vi "string parse mathematica list assosiated array -- V2.vi"(6 "pattern":string="^[\\t \\r \\n \\s \\, ]*\\\"(.+?)\\\"[\\t \\r \\n \\s]*\\-\\>[\\t \\r \\n \\s]*\\<\\|([^\\|]+)\\|\\>", 7 "action":T2=enum."create string", 8 "array of inds":dbl[](array[numeric]), 9 "array of IDs":string[](array[string]), 10 "Map IN":map{string, map{T1, dbl}}(c390), 11 "string IN":string="\n8048 -> <|\"\\[Zeta]\" -> 0.264284777894, \"\\[Tau]1\" -> 0.029921918685, \n   \"\\[Tau]S\" -> 0.192386764745, \"\\[Tau]N\" -> 0.181403587913, \n   \"\\[Tau]C\" -> 0.001052808010, \"\\[Kappa]0\" -> 0.000000000660, \n   \"mm1\" -> 0.000000000000, \"mm2\" -> 0.000000000000, \n   \"mm3\" -> 0.000000000000, \"T\" -> 0.170000000000, \n   \"B\" -> 12, \"\\[Theta]\" -> 0.000000000000|>, \n8049 -> <|\"\\[Zeta]\" -> 0.201102232421, \"\\[Tau]1\" -> 0.027404257658, \n   \"\\[Tau]S\" -> 0.119081991530, \"\\[Tau]N\" -> 0.102233037825, \n   \"\\[Tau]C\" -> 0.001034759526, \"\\[Kappa]0\" -> 0.000000000924, \n   \"mm1\" -> 0.000000000000, \"mm2\" -> 0.000000000000, \n   \"mm3\" -> 0.000000000000, \"T\" -> 0.200000000000, \n   \"B\" -> 12, \"\\[Theta]\" -> 0.000000000000|>, \n8050 -> <|\"\\[Zeta]\" -> 0.169063131197, \"\\[Tau]1\" -> 0.023551252455, \n   \"\\[Tau]S\" -> 0.088556796938, \"\\[Tau]N\" -> 0.073591360902, \n   \"\\[Tau]C\" -> 0.001008773464, \"\\[Kappa]0\" -> 0.000000001052, \n   \"mm1\" -> 0.000000000000, \"mm2\" -> 0.000000000000, \n   \"mm3\" -> 0.000000000000, \"T\" -> 0.220000000000, \n   \"B\" -> 12, \"\\[Theta]\" -> 0.000000000000|>, \n8051 -> <|\"\\[Zeta]\" -> 0.091539753140, \"\\[Tau]1\" -> 0.021589342173, \n   \"\\[Tau]S\" -> 0.069591266812, \"\\[Tau]N\" -> 0.024713101747, \n   \"\\[Tau]C\" -> 0.001578835918, \"\\[Kappa]0\" -> 0.000000001376, \n   \"mm1\" -> 0.000000000000, \"mm2\" -> 0.000000000000, \n   \"mm3\" -> 0.000000000000, \"T\" -> 0.280000000000, \n   \"B\" -> 12, \"\\[Theta]\" -> 0.000000000000|>, \n8052 -> <|\"\\[Zeta]\" -> 0.064241434685, \"\\[Tau]1\" -> 0.021883189624, \n   \"\\[Tau]S\" -> 0.054526069267, \"\\[Tau]N\" -> 0.012051949674, \n   \"\\[Tau]C\" -> 0.001858120134, \"\\[Kappa]0\" -> 0.000000001749, \n   \"mm1\" -> 0.000000000000, \"mm2\" -> 0.000000000000, \n   \"mm3\" -> 0.000000000000, \"T\" -> 0.330000000000, \n   \"B\" -> 12, \"\\[Theta]\" -> 0.000000000000|>, \n8053 -> <|\"\\[Zeta]\" -> 0.046671238462, \"\\[Tau]1\" -> 0.021035137247, \n   \"\\[Tau]S\" -> 0.044251032051, \"\\[Tau]N\" -> 0.006393660877, \n   \"\\[Tau]C\" -> 0.002341606240, \"\\[Kappa]0\" -> 0.000000002165, \n   \"mm1\" -> 0.000000000000, \"mm2\" -> 0.000000000000, \n   \"mm3\" -> 0.000000000000, \"T\" -> 0.400000000000, \n   \"B\" -> 12, \"\\[Theta]\" -> 0.000000000000|>, \n 8054 -> <|\"\\[Zeta]\" -> 0.036507468942, \"\\[Tau]1\" -> 0.016809078537, \n   \"\\[Tau]S\" -> 0.036180977899, \"\\[Tau]N\" -> 0.004191377428, \n   \"\\[Tau]C\" -> 0.002304673955, \"\\[Kappa]0\" -> 0.000000002675, \n   \"mm1\" -> 0.000000000000, \"mm2\" -> 0.000000000000, \n   \"mm3\" -> 0.000000000000, \"T\" -> 0.480000000000, \n   \"B\" -> 12, \"\\[Theta]\" -> 0.000000000000|>, \n 8055 -> <|\"\\[Zeta]\" -> 0.030833243094, \"\\[Tau]1\" -> 0.018820733306, \n   \"\\[Tau]S\" -> 0.030309186701, \"\\[Tau]N\" -> 0.002241639015, \n   \"\\[Tau]C\" -> 0.002272740822, \"\\[Kappa]0\" -> 0.000000003352, \n   \"mm1\" -> 0.000000000000, \"mm2\" -> 0.000000000000, \n   \"mm3\" -> 0.000000000000, \"T\" -> 0.580000000000, \n   \"B\" -> 12, \"\\[Theta]\" -> 0.000000000000|>, \n 8056 -> <|\"\\[Zeta]\" -> 0.019920170845, \"\\[Tau]1\" -> 0.016368892412, \n   \"\\[Tau]S\" -> 0.030579536580, \"\\[Tau]N\" -> 0.001736017565, \n   \"\\[Tau]C\" -> 0.004971418152, \"\\[Kappa]0\" -> 0.000000004410, \n   \"mm1\" -> 0.000000000000, \"mm2\" -> 0.000000000000, \n   \"mm3\" -> 0.000000000000, \"T\" -> 0.680000000000, \n   \"B\" -> 12, \"\\[Theta]\" -> 0.000000000000|>, \n 8057 -> <|\"\\[Zeta]\" -> 0.017558473054, \"\\[Tau]1\" -> 0.014545104284, \n   \"\\[Tau]S\" -> 0.022979681288, \"\\[Tau]N\" -> 0.000840829385, \n   \"\\[Tau]C\" -> 0.005228030240, \"\\[Kappa]0\" -> 0.000000006068, \n   \"mm1\" -> 0.000000000000, \"mm2\" -> 0.000000000000, \n   \"mm3\" -> 0.000000000000, \"T\" -> 0.910000000000, \n   \"B\" -> 12, \"\\[Theta]\" -> 0.000000000000|>, \n 8058 -> <|\"\\[Zeta]\" -> 0.011916480594, \"\\[Tau]1\" -> 0.012551282481, \n   \"\\[Tau]S\" -> 0.018233218660, \"\\[Tau]N\" -> 0.000345702746, \n   \"\\[Tau]C\" -> 0.004699451527, \"\\[Kappa]0\" -> 0.000000008451, \n   \"mm1\" -> 0.000000000000, \"mm2\" -> 0.000000000000, \n   \"mm3\" -> 0.000000000000, \"T\" -> 1.230000000000, \n   \"B\" -> 12, \"\\[Theta]\" -> 0.000000000000|>, \n 8059 -> <|\"\\[Zeta]\" -> 0.012831327568, \"\\[Tau]1\" -> 0.013315909415, \n   \"\\[Tau]S\" -> 0.012590836847, \"\\[Tau]N\" -> 0.000065003013, \n   \"\\[Tau]C\" -> 0.005276356243, \"\\[Kappa]0\" -> 0.000000013610, \n   \"mm1\" -> 0.000000000000, \"mm2\" -> 0.000000000000, \n   \"mm3\" -> 0.000000000000, \"T\" -> 1.970000000000, \n   \"B\" -> 12, \"\\[Theta]\" -> 0.000000000000|>, \n 8060 -> <|\"\\[Zeta]\" -> 0.019774146838, \"\\[Tau]1\" -> 0.013257273421, \n   \"\\[Tau]S\" -> 0.007064131508, \"\\[Tau]N\" -> 0.000028000819, \n   \"\\[Tau]C\" -> 0.006942241845, \"\\[Kappa]0\" -> 0.000000023477, \n   \"mm1\" -> 0.000000000000, \"mm2\" -> 0.000000000000, \n   \"mm3\" -> 0.000000000000, \"T\" -> 3.190000000000, \n   \"B\" -> 12, \"\\[Theta]\" -> 0.000000000000|>, \n 8061 -> <|\"\\[Zeta]\" -> 0.029251354442, \"\\[Tau]1\" -> 0.014634751206, \n   \"\\[Tau]S\" -> 0.003873958746, \"\\[Tau]N\" -> 0.000007000487, \n   \"\\[Tau]C\" -> 0.006827504775, \"\\[Kappa]0\" -> 0.000000056438, \n   \"mm1\" -> 0.000000000000, \"mm2\" -> 0.000000000000, \n   \"mm3\" -> 0.000000000000, \"T\" -> 5.820000000000, \n   \"B\" -> 12, \"\\[Theta]\" -> 0.000000000000 |>, \n   \n 8070 -> <|\"\\[Zeta]\" -> 0.192260325342, \"\\[Tau]1\" -> 0.068971960572, \n   \"\\[Tau]S\" -> 0.034724103146, \"\\[Tau]N\" -> 0.116916926394, \n   \"\\[Tau]C\" -> 0.001339007531, \"\\[Kappa]0\" -> 0.000000000920, \n   \"mm1\" -> 0.000000000000, \"mm2\" -> 0.000000000000, \n   \"mm3\" -> 0.000000000000, \"T\" -> 0.200000000000, \n   \"B\" -> 12, \"\\[Theta]\" -> 90.000000000000 |>, \n   \n 8071 -> <|\"\\[Zeta]\" -> 0.287121975239, \"\\[Tau]1\" -> 0.116231019165, \n   \"\\[Tau]S\" -> 0.066964365948, \"\\[Tau]N\" -> 1.031943818405, \n   \"\\[Tau]C\" -> 0.001579683432, \"\\[Kappa]0\" -> 0.000000000546, \n   \"mm1\" -> 0.000000000000, \"mm2\" -> 0.000000000000, \n   \"mm3\" -> 0.000000000000, \"T\" -> 0.140000000000, \n   \"B\" -> 12, \"\\[Theta]\" -> 90.000000000000 |>, \n   \n 8072 -> <|\"\\[Zeta]\" -> 0.256563977847, \"\\[Tau]1\" -> 0.091128230148, \n   \"\\[Tau]S\" -> 0.042349271948, \"\\[Tau]N\" -> 0.264223732455, \n   \"\\[Tau]C\" -> 0.001175524600, \"\\[Kappa]0\" -> 0.000000000659, \n   \"mm1\" -> 0.000000000000, \"mm2\" -> 0.000000000000, \n   \"mm3\" -> 0.000000000000, \"T\" -> 0.180000000000, \n   \"B\" -> 12, \"\\[Theta]\" -> 90.000000000000|>, \n 8073 -> <|\"\\[Zeta]\" -> 0.166463706425, \"\\[Tau]1\" -> 0.068258677765, \n   \"\\[Tau]S\" -> 0.032169678694, \"\\[Tau]N\" -> 0.089325850968, \n   \"\\[Tau]C\" -> 0.001296501731, \"\\[Kappa]0\" -> 0.000000001072, \n   \"mm1\" -> 0.000000000000, \"mm2\" -> 0.000000000000, \n   \"mm3\" -> 0.000000000000, \"T\" -> 0.220000000000, \n   \"B\" -> 12, \"\\[Theta]\" -> 90.000000000000|>, \n 8074 -> <|\"\\[Zeta]\" -> 0.096966986681, \"\\[Tau]1\" -> 0.051268159149, \n   \"\\[Tau]S\" -> 0.027100433808, \"\\[Tau]N\" -> 0.035158364681, \n   \"\\[Tau]C\" -> 0.001794012368, \"\\[Kappa]0\" -> 0.000000001377, \n   \"mm1\" -> 0.000000000000, \"mm2\" -> 0.000000000000, \n   \"mm3\" -> 0.000000000000, \"T\" -> 0.270000000000, \n   \"B\" -> 12, \"\\[Theta]\" -> 90.000000000000|>, \n 8075 -> <|\"\\[Zeta]\" -> 0.069751073871, \"\\[Tau]1\" -> 0.043839592936, \n   \"\\[Tau]S\" -> 0.023745040482, \"\\[Tau]N\" -> 0.017573258627, \n   \"\\[Tau]C\" -> 0.001911807541, \"\\[Kappa]0\" -> 0.000000001743, \n   \"mm1\" -> 0.000000000000, \"mm2\" -> 0.000000000000, \n   \"mm3\" -> 0.000000000000, \"T\" -> 0.330000000000, \n   \"B\" -> 12, \"\\[Theta]\" -> 90.000000000000|>, \n 8076 -> <|\"\\[Zeta]\" -> 0.051456166730, \"\\[Tau]1\" -> 0.036962114127, \n   \"\\[Tau]S\" -> 0.021589166615, \"\\[Tau]N\" -> 0.010172333923, \n   \"\\[Tau]C\" -> 0.002367575609, \"\\[Kappa]0\" -> 0.000000002122, \n   \"mm1\" -> 0.000000000000, \"mm2\" -> 0.000000000000, \n   \"mm3\" -> 0.000000000000, \"T\" -> 0.390000000000, \n   \"B\" -> 12, \"\\[Theta]\" -> 90.000000000000|>, \n 8077 -> <|\"\\[Zeta]\" -> 0.038526442831, \"\\[Tau]1\" -> 0.026952038906, \n   \"\\[Tau]S\" -> 0.019853633024, \"\\[Tau]N\" -> 0.005229312619, \n   \"\\[Tau]C\" -> 0.002387050238, \"\\[Kappa]0\" -> 0.000000002669, \n   \"mm1\" -> 0.000000000000, \"mm2\" -> 0.000000000000, \n   \"mm3\" -> 0.000000000000, \"T\" -> 0.480000000000, \n   \"B\" -> 12, \"\\[Theta]\" -> 90.000000000000|>, \n 8078 -> <|\"\\[Zeta]\" -> 0.031217986851, \"\\[Tau]1\" -> 0.022324330444, \n   \"\\[Tau]S\" -> 0.018861062526, \"\\[Tau]N\" -> 0.002718571339, \n   \"\\[Tau]C\" -> 0.002455004531, \"\\[Kappa]0\" -> 0.000000003343, \n   \"mm1\" -> 0.000000000000, \"mm2\" -> 0.000000000000, \n   \"mm3\" -> 0.000000000000, \"T\" -> 0.580000000000, \n   \"B\" -> 12, \"\\[Theta]\" -> 90.000000000000|>, \n 8079 -> <|\"\\[Zeta]\" -> 0.020568815513, \"\\[Tau]1\" -> 0.023045965648, \n   \"\\[Tau]S\" -> 0.020791387386, \"\\[Tau]N\" -> 0.002229171297, \n   \"\\[Tau]C\" -> 0.004427475438, \"\\[Kappa]0\" -> 0.000000004398, \n   \"mm1\" -> 0.000000000000, \"mm2\" -> 0.000000000000, \n   \"mm3\" -> 0.000000000000, \"T\" -> 0.680000000000, \n   \"B\" -> 12, \"\\[Theta]\" -> 90.000000000000|>, \n 8080 -> <|\"\\[Zeta]\" -> 0.016159836955, \"\\[Tau]1\" -> 0.019958638777, \n   \"\\[Tau]S\" -> 0.018730096307, \"\\[Tau]N\" -> 0.000899236968, \n   \"\\[Tau]C\" -> 0.005152267403, \"\\[Kappa]0\" -> 0.000000006087, \n   \"mm1\" -> 0.000000000000, \"mm2\" -> 0.000000000000, \n   \"mm3\" -> 0.000000000000, \"T\" -> 0.910000000000, \n   \"B\" -> 12, \"\\[Theta]\" -> 90.000000000000|>, \n 8081 -> <|\"\\[Zeta]\" -> 0.014495870556, \"\\[Tau]1\" -> 0.019990087457, \n   \"\\[Tau]S\" -> 0.016832201384, \"\\[Tau]N\" -> 0.000455517238, \n   \"\\[Tau]C\" -> 0.005555782498, \"\\[Kappa]0\" -> 0.000000008420, \n   \"mm1\" -> 0.000000000000, \"mm2\" -> 0.000000000000, \n   \"mm3\" -> 0.000000000000, \"T\" -> 1.230000000000, \n   \"B\" -> 12, \"\\[Theta]\" -> 90.000000000000|>, \n 8082 -> <|\"\\[Zeta]\" -> 0.014043763709, \"\\[Tau]1\" -> 0.018292068543, \n   \"\\[Tau]S\" -> 0.011311396743, \"\\[Tau]N\" -> 0.000128802259, \n   \"\\[Tau]C\" -> 0.008087849636, \"\\[Kappa]0\" -> 0.000000014258, \n   \"mm1\" -> 0.000000000000, \"mm2\" -> 0.000000000000, \n   \"mm3\" -> 0.000000000000, \"T\" -> 2.050000000000, \n   \"B\" -> 12, \"\\[Theta]\" -> 90.000000000000|>, \n 8083 -> <|\"\\[Zeta]\" -> 0.016187684631, \"\\[Tau]1\" -> 0.018325345271, \n   \"\\[Tau]S\" -> 0.007510087776, \"\\[Tau]N\" -> 0.000028419157, \n   \"\\[Tau]C\" -> 0.008115463080, \"\\[Kappa]0\" -> 0.000000024747, \n   \"mm1\" -> 0.000000000000, \"mm2\" -> 0.000000000000, \n   \"mm3\" -> 0.000000000000, \"T\" -> 3.310000000000, \n   \"B\" -> 12, \"\\[Theta]\" -> 90.000000000000|>, \n 8084 -> <|\"\\[Zeta]\" -> 0.027897403691, \"\\[Tau]1\" -> 0.014639690770, \n   \"\\[Tau]S\" -> 0.004105291179, \"\\[Tau]N\" -> 0.000006999171, \n   \"\\[Tau]C\" -> 0.007414449545, \"\\[Kappa]0\" -> 0.000000059701, \n   \"mm1\" -> 0.000000000000, \"mm2\" -> 0.000000000000, \n   \"mm3\" -> 0.000000000000, \"T\" -> 6.000000000000, \n   \"B\" -> 12, \"\\[Theta]\" -> 90.000000000000|>,") -> (2 "Map OUT":map{string, map{T1, dbl}}(c390), 3 "string out":string="  \"IDS0158_210310_RAW_cal__ref_\" ->   <| \"ζ\"->  0.331549170129  , \"τ1\"-> 0.031957261989  , \"τS\"-> 0.245155954508  , \"τN\"-> 0.327332604975  , \"τC\"-> 0.001044440547  , \"κ0\"-> 0.000000000511  , \"mm1\"-> 0.000000000000  , \"mm2\"-> 0.000000000000  , \"mm3\"-> 0.000000000000  , \"T\"->  0.140000000000  , \"B\"-> 12.000000000000  , \"θ\"-> 0.000000000000  , \"Reoff\"-> 0.000000000000  ,  \"Imoff\"-> 0.000000000000  |>   , \r\"IDS0158_210310_RAW_cal__sam_\" ->   <| \"ζ\"->  0.286336668596  , \"τ1\"-> 0.037477267671  , \"τS\"-> 0.354459287884  , \"τN\"-> 0.444916383639  , \"τC\"-> 0.001225600579  , \"κ0\"-> 0.000000000596  , \"mm1\"-> 0.000000000000  , \"mm2\"-> 0.000000000000  , \"mm3\"-> 0.000000000000  , \"T\"->  0.140000000000  , \"B\"-> 12.000000000000  , \"θ\"-> 0.000000000000  , \"Reoff\"-> 0.000000000000  ,  \"Imoff\"-> 0.000000000000  |>   , \r\"IDS0159_210310_RAW_cal__ref_\" ->   <| \"ζ\"->  0.269623663752  , \"τ1\"-> 0.029946823009  , \"τS\"-> 0.193020268264  , \"τN\"-> 0.181925572107  , \"τC\"-> 0.001029221853  , \"κ0\"-> 0.000000000645  , \"mm1\"-> 0.000000000000  , \"mm2\"-> 0.000000000000  , \"mm3\"-> 0.000000000000  , \"T\"->  0.170000000000  , \"B\"-> 12.000000000000  , \"θ\"-> 0.000000000000  , \"Reoff\"-> 0.000000000000  ,  \"Imoff\"-> 0.000000000000  |>   , \r\"IDS0159_210310_RAW_cal__sam_\" ->   <| \"ζ\"->  0.219100303741  , \"τ1\"-> 0.028643012604  , \"τS\"-> 0.279362928811  , \"τN\"-> 0.246156444058  , \"τC\"-> 0.001272401549  , \"κ0\"-> 0.000000000760  , \"mm1\"-> 0.000000000000  , \"mm2\"-> 0.000000000000  , \"mm3\"-> 0.000000000000  , \"T\"->  0.170000000000  , \"B\"-> 12.000000000000  , \"θ\"-> 0.000000000000  , \"Reoff\"-> 0.000000000000  ,  \"Imoff\"-> 0.000000000000  |>   , \r\"IDS0160_210310_RAW_cal__ref_\" ->   <| \"ζ\"->  0.207047266456  , \"τ1\"-> 0.027475093360  , \"τS\"-> 0.117497913331  , \"τN\"-> 0.102020652890  , \"τC\"-> 0.000950950989  , \"κ0\"-> 0.000000000918  , \"mm1\"-> 0.000000000000  , \"mm2\"-> 0.000000000000  , \"mm3\"-> 0.000000000000  , \"T\"->  0.200000000000  , \"B\"-> 12.000000000000  , \"θ\"-> 0.000000000000  , \"Reoff\"-> 0.000000000000  ,  \"Imoff\"-> 0.000000000000  |>   , \r\"IDS0160_210310_RAW_cal__sam_\" ->   <| \"ζ\"->  0.170488637524  , \"τ1\"-> 0.029234231120  , \"τS\"-> 0.149095458227  , \"τN\"-> 0.151792620275  , \"τC\"-> 0.001113424175  , \"κ0\"-> 0.000000001042  , \"mm1\"-> 0.000000000000  , \"mm2\"-> 0.000000000000  , \"mm3\"-> 0.000000000000  , \"T\"->  0.200000000000  , \"B\"-> 12.000000000000  , \"θ\"-> 0.000000000000  , \"Reoff\"-> 0.000000000000  ,  \"Imoff\"-> 0.000000000000  |>   , \r\"IDS0161_210310_RAW_cal__ref_\" ->   <| \"ζ\"->  0.165418845287  , \"τ1\"-> 0.025256902580  , \"τS\"-> 0.095232124148  , \"τN\"-> 0.068477414693  , \"τC\"-> 0.001100413424  , \"κ0\"-> 0.000000001058  , \"mm1\"-> 0.000000000000  , \"mm2\"-> 0.000000000000  , \"mm3\"-> 0.000000000000  , \"T\"->  0.220000000000  , \"B\"-> 12.000000000000  , \"θ\"-> 0.000000000000  , \"Reoff\"-> 0.000000000000  ,  \"Imoff\"-> 0.000000000000  |>   , \r\"IDS0161_210310_RAW_cal__sam_\" ->   <| \"ζ\"->  0.130531197151  , \"τ1\"-> 0.025704482770  , \"τS\"-> 0.129606657196  , \"τN\"-> 0.091602369165  , \"τC\"-> 0.001441379995  , \"κ0\"-> 0.000000001211  , \"mm1\"-> 0.000000000000  , \"mm2\"-> 0.000000000000  , \"mm3\"-> 0.000000000000  , \"T\"->  0.220000000000  , \"B\"-> 12.000000000000  , \"θ\"-> 0.000000000000  , \"Reoff\"-> 0.000000000000  ,  \"Imoff\"-> 0.000000000000  |>   , \r\"IDS0162_210310_RAW_cal__ref_\" ->   <| \"ζ\"->  0.094488415983  , \"τ1\"-> 0.023440091411  , \"τS\"-> 0.070629137621  , \"τN\"-> 0.023695223047  , \"τC\"-> 0.001462465509  , \"κ0\"-> 0.000000001371  , \"mm1\"-> 0.000000000000  , \"mm2\"-> 0.000000000000  , \"mm3\"-> 0.000000000000  , \"T\"->  0.280000000000  , \"B\"-> 12.000000000000  , \"θ\"-> 0.000000000000  , \"Reoff\"-> 0.000000000000  ,  \"Imoff\"-> 0.000000000000  |>   , \r\"IDS0162_210310_RAW_cal__sam_\" ->   <| \"ζ\"->  0.078258046754  , \"τ1\"-> 0.028009840731  , \"τS\"-> 0.092122038762  , \"τN\"-> 0.030129595899  , \"τC\"-> 0.001641062244  , \"κ0\"-> 0.000000001543  , \"mm1\"-> 0.000000000000  , \"mm2\"-> 0.000000000000  , \"mm3\"-> 0.000000000000  , \"T\"->  0.280000000000  , \"B\"-> 12.000000000000  , \"θ\"-> 0.000000000000  , \"Reoff\"-> 0.000000000000  ,  \"Imoff\"-> 0.000000000000  |>   , \r\"IDS0163_210310_RAW_cal__ref_\" ->   <| \"ζ\"->  0.066045279838  , \"τ1\"-> 0.021690723483  , \"τS\"-> 0.054398710223  , \"τN\"-> 0.012159058060  , \"τC\"-> 0.001677829713  , \"κ0\"-> 0.000000001745  , \"mm1\"-> 0.000000000000  , \"mm2\"-> 0.000000000000  , \"mm3\"-> 0.000000000000  , \"T\"->  0.330000000000  , \"B\"-> 12.000000000000  , \"θ\"-> 0.000000000000  , \"Reoff\"-> 0.000000000000  ,  \"Imoff\"-> 0.000000000000  |>   , \r\"IDS0163_210310_RAW_cal__sam_\" ->   <| \"ζ\"->  0.054088186012  , \"τ1\"-> 0.023838802615  , \"τS\"-> 0.069079396629  , \"τN\"-> 0.016435267456  , \"τC\"-> 0.002025071743  , \"κ0\"-> 0.000000001955  , \"mm1\"-> 0.000000000000  , \"mm2\"-> 0.000000000000  , \"mm3\"-> 0.000000000000  , \"T\"->  0.330000000000  , \"B\"-> 12.000000000000  , \"θ\"-> 0.000000000000  , \"Reoff\"-> 0.000000000000  ,  \"Imoff\"-> 0.000000000000  |>   , \r\"IDS0164_210310_RAW_cal__ref_\" ->   <| \"ζ\"->  0.046429657722  , \"τ1\"-> 0.021005913305  , \"τS\"-> 0.044250298502  , \"τN\"-> 0.006399419767  , \"τC\"-> 0.002349605146  , \"κ0\"-> 0.000000002166  , \"mm1\"-> 0.000000000000  , \"mm2\"-> 0.000000000000  , \"mm3\"-> 0.000000000000  , \"T\"->  0.400000000000  , \"B\"-> 12.000000000000  , \"θ\"-> 0.000000000000  , \"Reoff\"-> 0.000000000000  ,  \"Imoff\"-> 0.000000000000  |>   , \r\"IDS0164_210310_RAW_cal__sam_\" ->   <| \"ζ\"->  0.039314966212  , \"τ1\"-> 0.020712803909  , \"τS\"-> 0.055413767550  , \"τN\"-> 0.008474403424  , \"τC\"-> 0.002674063387  , \"κ0\"-> 0.000000002415  , \"mm1\"-> 0.000000000000  , \"mm2\"-> 0.000000000000  , \"mm3\"-> 0.000000000000  , \"T\"->  0.400000000000  , \"B\"-> 12.000000000000  , \"θ\"-> 0.000000000000  , \"Reoff\"-> 0.000000000000  ,  \"Imoff\"-> 0.000000000000  |>   , \r\"IDS0165_210310_RAW_cal__ref_\" ->   <| \"ζ\"->  0.033449822896  , \"τ1\"-> 0.018946770596  , \"τS\"-> 0.035864277160  , \"τN\"-> 0.004007639534  , \"τC\"-> 0.003128970761  , \"κ0\"-> 0.000000002686  , \"mm1\"-> 0.000000000000  , \"mm2\"-> 0.000000000000  , \"mm3\"-> 0.000000000000  , \"T\"->  0.480000000000  , \"B\"-> 12.000000000000  , \"θ\"-> 0.000000000000  , \"Reoff\"-> 0.000000000000  ,  \"Imoff\"-> 0.000000000000  |>   , \r\"IDS0165_210310_RAW_cal__sam_\" ->   <| \"ζ\"->  0.031945976845  , \"τ1\"-> 0.019000922826  , \"τS\"-> 0.045624146388  , \"τN\"-> 0.005314716063  , \"τC\"-> 0.002488383471  , \"κ0\"-> 0.000000002954  , \"mm1\"-> 0.000000000000  , \"mm2\"-> 0.000000000000  , \"mm3\"-> 0.000000000000  , \"T\"->  0.480000000000  , \"B\"-> 12.000000000000  , \"θ\"-> 0.000000000000  , \"Reoff\"-> 0.000000000000  ,  \"Imoff\"-> 0.000000000000  |>   , \r\"IDS0166_210310_RAW_cal__ref_\" ->   <| \"ζ\"->  0.026131121682  , \"τ1\"-> 0.018837612836  , \"τS\"-> 0.029051745056  , \"τN\"-> 0.002477027845  , \"τC\"-> 0.003638595201  , \"κ0\"-> 0.000000003369  , \"mm1\"-> 0.000000000000  , \"mm2\"-> 0.000000000000  , \"mm3\"-> 0.000000000000  , \"T\"->  0.580000000000  , \"B\"-> 12.000000000000  , \"θ\"-> 0.000000000000  , \"Reoff\"-> 0.000000000000  ,  \"Imoff\"-> 0.000000000000  |>   , \r\"IDS0166_210310_RAW_cal__sam_\" ->   <| \"ζ\"->  0.023031239946  , \"τ1\"-> 0.018268814012  , \"τS\"-> 0.037269400776  , \"τN\"-> 0.002696792890  , \"τC\"-> 0.003257395394  , \"κ0\"-> 0.000000003720  , \"mm1\"-> 0.000000000000  , \"mm2\"-> 0.000000000000  , \"mm3\"-> 0.000000000000  , \"T\"->  0.580000000000  , \"B\"-> 12.000000000000  , \"θ\"-> 0.000000000000  , \"Reoff\"-> 0.000000000000  ,  \"Imoff\"-> 0.000000000000  |>   , \r\"IDS0167_210310_RAW_cal__ref_\" ->   <| \"ζ\"->  0.026557278794  , \"τ1\"-> 0.016933945977  , \"τS\"-> 0.022881111855  , \"τN\"-> 0.001392473895  , \"τC\"-> 0.004119437148  , \"κ0\"-> 0.000000003981  , \"mm1\"-> 0.000000000000  , \"mm2\"-> 0.000000000000  , \"mm3\"-> 0.000000000000  , \"T\"->  0.680000000000  , \"B\"-> 12.000000000000  , \"θ\"-> 0.000000000000  , \"Reoff\"-> 0.000000000000  ,  \"Imoff\"-> 0.000000000000  |>   , \r\"IDS0167_210310_RAW_cal__sam_\" ->   <| \"ζ\"->  0.019920170845  , \"τ1\"-> 0.016368892412  , \"τS\"-> 0.030579536580  , \"τN\"-> 0.001736017565  , \"τC\"-> 0.004971418152  , \"κ0\"-> 0.000000004410  , \"mm1\"-> 0.000000000000  , \"mm2\"-> 0.000000000000  , \"mm3\"-> 0.000000000000  , \"T\"->  0.680000000000  , \"B\"-> 12.000000000000  , \"θ\"-> 0.000000000000  , \"Reoff\"-> 0.000000000000  ,  \"Imoff\"-> 0.000000000000  |>   , \r\"IDS0168_210310_RAW_cal__ref_\" ->   <| \"ζ\"->  0.022041296958  , \"τ1\"-> 0.014045615335  , \"τS\"-> 0.018889590451  , \"τN\"-> 0.000813465770  , \"τC\"-> 0.004122617309  , \"κ0\"-> 0.000000005540  , \"mm1\"-> 0.000000000000  , \"mm2\"-> 0.000000000000  , \"mm3\"-> 0.000000000000  , \"T\"->  0.910000000000  , \"B\"-> 12.000000000000  , \"θ\"-> 0.000000000000  , \"Reoff\"-> 0.000000000000  ,  \"Imoff\"-> 0.000000000000  |>   , \r\"IDS0168_210310_RAW_cal__sam_\" ->   <| \"ζ\"->  0.017558473054  , \"τ1\"-> 0.014545104284  , \"τS\"-> 0.022979681288  , \"τN\"-> 0.000840829385  , \"τC\"-> 0.005228030240  , \"κ0\"-> 0.000000006068  , \"mm1\"-> 0.000000000000  , \"mm2\"-> 0.000000000000  , \"mm3\"-> 0.000000000000  , \"T\"->  0.910000000000  , \"B\"-> 12.000000000000  , \"θ\"-> 0.000000000000  , \"Reoff\"-> 0.000000000000  ,  \"Imoff\"-> 0.000000000000  |>   , \r\"IDS0169_210310_RAW_cal__ref_\" ->   <| \"ζ\"->  0.021090283514  , \"τ1\"-> 0.013945744068  , \"τS\"-> 0.014386606899  , \"τN\"-> 0.000345175874  , \"τC\"-> 0.004902956629  , \"κ0\"-> 0.000000007742  , \"mm1\"-> 0.000000000000  , \"mm2\"-> 0.000000000000  , \"mm3\"-> 0.000000000000  , \"T\"->  1.230000000000  , \"B\"-> 12.000000000000  , \"θ\"-> 0.000000000000  , \"Reoff\"-> 0.000000000000  ,  \"Imoff\"-> 0.000000000000  |>   , \r\"IDS0169_210310_RAW_cal__sam_\" ->   <| \"ζ\"->  0.011916480594  , \"τ1\"-> 0.012551282481  , \"τS\"-> 0.018233218660  , \"τN\"-> 0.000345702746  , \"τC\"-> 0.004699451527  , \"κ0\"-> 0.000000008451  , \"mm1\"-> 0.000000000000  , \"mm2\"-> 0.000000000000  , \"mm3\"-> 0.000000000000  , \"T\"->  1.230000000000  , \"B\"-> 12.000000000000  , \"θ\"-> 0.000000000000  , \"Reoff\"-> 0.000000000000  ,  \"Imoff\"-> 0.000000000000  |>   , \r\"IDS0170_210310_RAW_cal__ref_\" ->   <| \"ζ\"->  0.021449250230  , \"τ1\"-> 0.014564522147  , \"τS\"-> 0.008878867204  , \"τN\"-> 0.000064984242  , \"τC\"-> 0.006207353748  , \"κ0\"-> 0.000000012530  , \"mm1\"-> 0.000000000000  , \"mm2\"-> 0.000000000000  , \"mm3\"-> 0.000000000000  , \"T\"->  1.970000000000  , \"B\"-> 12.000000000000  , \"θ\"-> 0.000000000000  , \"Reoff\"-> 0.000000000000  ,  \"Imoff\"-> 0.000000000000  |>   , \r\"IDS0170_210310_RAW_cal__sam_\" ->   <| \"ζ\"->  0.012831327568  , \"τ1\"-> 0.013315909415  , \"τS\"-> 0.012590836847  , \"τN\"-> 0.000065003013  , \"τC\"-> 0.005276356243  , \"κ0\"-> 0.000000013610  , \"mm1\"-> 0.000000000000  , \"mm2\"-> 0.000000000000  , \"mm3\"-> 0.000000000000  , \"T\"->  1.970000000000  , \"B\"-> 12.000000000000  , \"θ\"-> 0.000000000000  , \"Reoff\"-> 0.000000000000  ,  \"Imoff\"-> 0.000000000000  |>   , \r\"IDS0171_210310_RAW_cal__ref_\" ->   <| \"ζ\"->  0.024633693577  , \"τ1\"-> 0.014940694735  , \"τS\"-> 0.006137734482  , \"τN\"-> 0.000014567254  , \"τC\"-> 0.005080683927  , \"κ0\"-> 0.000000022488  , \"mm1\"-> 0.000000000000  , \"mm2\"-> 0.000000000000  , \"mm3\"-> 0.000000000000  , \"T\"->  3.190000000000  , \"B\"-> 12.000000000000  , \"θ\"-> 0.000000000000  , \"Reoff\"-> 0.000000000000  ,  \"Imoff\"-> 0.000000000000  |>   , \r\"IDS0171_210310_RAW_cal__sam_\" ->   <| \"ζ\"->  0.019774146838  , \"τ1\"-> 0.013257273421  , \"τS\"-> 0.007064131508  , \"τN\"-> 0.000028000819  , \"τC\"-> 0.006942241845  , \"κ0\"-> 0.000000023477  , \"mm1\"-> 0.000000000000  , \"mm2\"-> 0.000000000000  , \"mm3\"-> 0.000000000000  , \"T\"->  3.190000000000  , \"B\"-> 12.000000000000  , \"θ\"-> 0.000000000000  , \"Reoff\"-> 0.000000000000  ,  \"Imoff\"-> 0.000000000000  |>   , \r\"IDS0172_210310_RAW_cal__ref_\" ->   <| \"ζ\"->  0.027835388666  , \"τ1\"-> 0.013976390421  , \"τS\"-> 0.003539188638  , \"τN\"-> 0.000003774856  , \"τC\"-> 0.004420299329  , \"κ0\"-> 0.000000055482  , \"mm1\"-> 0.000000000000  , \"mm2\"-> 0.000000000000  , \"mm3\"-> 0.000000000000  , \"T\"->  5.800000000000  , \"B\"-> 12.000000000000  , \"θ\"-> 0.000000000000  , \"Reoff\"-> 0.000000000000  ,  \"Imoff\"-> 0.000000000000  |>   , \r\"IDS0172_210310_RAW_cal__sam_\" ->   <| \"ζ\"->  0.029251354442  , \"τ1\"-> 0.014634751206  , \"τS\"-> 0.003873958746  , \"τN\"-> 0.000007000487  , \"τC\"-> 0.006827504775  , \"κ0\"-> 0.000000056438  , \"mm1\"-> 0.000000000000  , \"mm2\"-> 0.000000000000  , \"mm3\"-> 0.000000000000  , \"T\"->  5.800000000000  , \"B\"-> 12.000000000000  , \"θ\"-> 0.000000000000  , \"Reoff\"-> 0.000000000000  ,  \"Imoff\"-> 0.000000000000  |>   , \r\"IDS0181_210310_RAW_cal__ref_\" ->   <| \"ζ\"->  0.194847779603  , \"τ1\"-> 0.071300022200  , \"τS\"-> 0.034370433557  , \"τN\"-> 0.000031210012  , \"τC\"-> 0.001245041457  , \"κ0\"-> 0.000000000909  , \"mm1\"-> 0.000000000000  , \"mm2\"-> 0.000000000000  , \"mm3\"-> 0.000000000000  , \"T\"->  0.179000000000  , \"B\"-> 12.000000000000  , \"θ\"-> 90.000000000000  , \"Reoff\"-> -60594059.405940592300  ,  \"Imoff\"-> 0.000000000000  |>   , \r\"IDS0181_210310_RAW_cal__sam_\" ->   <| \"ζ\"->  0.161975781729  , \"τ1\"-> 0.073089805113  , \"τS\"-> 0.045018408115  , \"τN\"-> 0.161987434028  , \"τC\"-> 0.001482104484  , \"κ0\"-> 0.000000001038  , \"mm1\"-> 0.000000000000  , \"mm2\"-> 0.000000000000  , \"mm3\"-> 0.000000000000  , \"T\"->  0.179000000000  , \"B\"-> 12.000000000000  , \"θ\"-> 90.000000000000  , \"Reoff\"-> 0.000000000000  ,  \"Imoff\"-> 0.000000000000  |>   , \r\"IDS0183_210310_RAW_cal__ref_\" ->   <| \"ζ\"->  0.368639553991  , \"τ1\"-> 0.116941860160  , \"τS\"-> 0.051705641175  , \"τN\"-> 0.670097053448  , \"τC\"-> 0.001215131262  , \"κ0\"-> 0.000000000441  , \"mm1\"-> 0.000000000000  , \"mm2\"-> 0.000000000000  , \"mm3\"-> 0.000000000000  , \"T\"->  0.120000000000  , \"B\"-> 12.000000000000  , \"θ\"-> 90.000000000000  , \"Reoff\"-> 0.000000000000  ,  \"Imoff\"-> 0.000000000000  |>   , \r\"IDS0183_210310_RAW_cal__sam_\" ->   <| \"ζ\"->  0.300863384227  , \"τ1\"-> 0.104924004009  , \"τS\"-> 0.071070599729  , \"τN\"-> 0.992887187112  , \"τC\"-> 0.001721587800  , \"κ0\"-> 0.000000000548  , \"mm1\"-> 0.000000000000  , \"mm2\"-> 0.000000000000  , \"mm3\"-> 0.000000000000  , \"T\"->  0.120000000000  , \"B\"-> 12.000000000000  , \"θ\"-> 90.000000000000  , \"Reoff\"-> 0.000000000000  ,  \"Imoff\"-> 0.000000000000  |>   , \r\"IDS0184_210310_RAW_cal__ref_\" ->   <| \"ζ\"->  0.260731272629  , \"τ1\"-> 0.088447317905  , \"τS\"-> 0.043671964304  , \"τN\"-> 0.000045653762  , \"τC\"-> 0.001151280234  , \"κ0\"-> 0.000000000662  , \"mm1\"-> 0.000000000000  , \"mm2\"-> 0.000000000000  , \"mm3\"-> 0.000000000000  , \"T\"->  0.148000000000  , \"B\"-> 12.000000000000  , \"θ\"-> 90.000000000000  , \"Reoff\"-> -60594059.405940592300  ,  \"Imoff\"-> 0.000000000000  |>   , \r\"IDS0184_210310_RAW_cal__sam_\" ->   <| \"ζ\"->  0.215697702358  , \"τ1\"-> 0.095971807771  , \"τS\"-> 0.069319630290  , \"τN\"-> 0.366712218878  , \"τC\"-> 0.001526252261  , \"κ0\"-> 0.000000000784  , \"mm1\"-> 0.000000000000  , \"mm2\"-> 0.000000000000  , \"mm3\"-> 0.000000000000  , \"T\"->  0.148000000000  , \"B\"-> 12.000000000000  , \"θ\"-> 90.000000000000  , \"Reoff\"-> 0.000000000000  ,  \"Imoff\"-> 0.000000000000  |>   , \r\"IDS0185_210310_RAW_cal__ref_\" ->   <| \"ζ\"->  0.194847779603  , \"τ1\"-> 0.071300022200  , \"τS\"-> 0.034370433557  , \"τN\"-> 0.000025767219  , \"τC\"-> 0.197000000000  , \"κ0\"-> 0.000000000909  , \"mm1\"-> 0.000000000000  , \"mm2\"-> 0.000000000000  , \"mm3\"-> 0.000000000000  , \"T\"->  0.197000000000  , \"B\"-> 12.000000000000  , \"θ\"-> 90.000000000000  , \"Reoff\"-> -60594059.405940592300  ,  \"Imoff\"-> 0.000000000000  |>   , \r\"IDS0185_210310_RAW_cal__sam_\" ->   <| \"ζ\"->  0.139117463690  , \"τ1\"-> 0.070330410174  , \"τS\"-> 0.040829719954  , \"τN\"-> 0.122434321115  , \"τC\"-> 0.001436112939  , \"κ0\"-> 0.000000001208  , \"mm1\"-> 0.000000000000  , \"mm2\"-> 0.000000000000  , \"mm3\"-> 0.000000000000  , \"T\"->  0.197000000000  , \"B\"-> 12.000000000000  , \"θ\"-> 90.000000000000  , \"Reoff\"-> 0.000000000000  ,  \"Imoff\"-> 0.000000000000  |>   , \r\"IDS0186_210310_RAW_cal__ref_\" ->   <| \"ζ\"->  0.194847779603  , \"τ1\"-> 0.071300022200  , \"τS\"-> 0.034370433557  , \"τN\"-> 0.000016128772  , \"τC\"-> 0.249000000000  , \"κ0\"-> 0.000000000909  , \"mm1\"-> 0.000000000000  , \"mm2\"-> 0.000000000000  , \"mm3\"-> 0.000000000000  , \"T\"->  0.249000000000  , \"B\"-> 12.000000000000  , \"θ\"-> 90.000000000000  , \"Reoff\"-> -60594059.405940592300  ,  \"Imoff\"-> 0.000000000000  |>   , \r\"IDS0186_210310_RAW_cal__sam_\" ->   <| \"ζ\"->  0.079912790251  , \"τ1\"-> 0.053932962768  , \"τS\"-> 0.033847624645  , \"τN\"-> 0.047947649984  , \"τC\"-> 0.001828917906  , \"κ0\"-> 0.000000001546  , \"mm1\"-> 0.000000000000  , \"mm2\"-> 0.000000000000  , \"mm3\"-> 0.000000000000  , \"T\"->  0.249000000000  , \"B\"-> 12.000000000000  , \"θ\"-> 90.000000000000  , \"Reoff\"-> 0.000000000000  ,  \"Imoff\"-> 0.000000000000  |>   , \r\"IDS0187_210310_RAW_cal__ref_\" ->   <| \"ζ\"->  0.070401604603  , \"τ1\"-> 0.043684283216  , \"τS\"-> 0.023756676354  , \"τN\"-> 0.017570167589  , \"τC\"-> 0.001809460237  , \"κ0\"-> 0.000000001742  , \"mm1\"-> 0.000000000000  , \"mm2\"-> 0.000000000000  , \"mm3\"-> 0.000000000000  , \"T\"->  0.300000000000  , \"B\"-> 12.000000000000  , \"θ\"-> 90.000000000000  , \"Reoff\"-> 0.000000000000  ,  \"Imoff\"-> 0.000000000000  |>   , \r\"IDS0187_210310_RAW_cal__sam_\" ->   <| \"ζ\"->  0.057938569833  , \"τ1\"-> 0.045244527663  , \"τS\"-> 0.029709028064  , \"τN\"-> 0.023577376257  , \"τC\"-> 0.002006607539  , \"κ0\"-> 0.000000001948  , \"mm1\"-> 0.000000000000  , \"mm2\"-> 0.000000000000  , \"mm3\"-> 0.000000000000  , \"T\"->  0.300000000000  , \"B\"-> 12.000000000000  , \"θ\"-> 90.000000000000  , \"Reoff\"-> 0.000000000000  ,  \"Imoff\"-> 0.000000000000  |>   , \r\"IDS0188_210310_RAW_cal__ref_\" ->   <| \"ζ\"->  0.052039078112  , \"τ1\"-> 0.037833987996  , \"τS\"-> 0.021664376950  , \"τN\"-> 0.010364100672  , \"τC\"-> 0.002302914949  , \"κ0\"-> 0.000000002119  , \"mm1\"-> 0.000000000000  , \"mm2\"-> 0.000000000000  , \"mm3\"-> 0.000000000000  , \"T\"->  0.360000000000  , \"B\"-> 12.000000000000  , \"θ\"-> 90.000000000000  , \"Reoff\"-> 0.000000000000  ,  \"Imoff\"-> 0.000000000000  |>   , \r\"IDS0188_210310_RAW_cal__sam_\" ->   <| \"ζ\"->  0.044154556051  , \"τ1\"-> 0.038823125235  , \"τS\"-> 0.027069314930  , \"τN\"-> 0.013601990730  , \"τC\"-> 0.002287979276  , \"κ0\"-> 0.000000002359  , \"mm1\"-> 0.000000000000  , \"mm2\"-> 0.000000000000  , \"mm3\"-> 0.000000000000  , \"T\"->  0.360000000000  , \"B\"-> 12.000000000000  , \"θ\"-> 90.000000000000  , \"Reoff\"-> 0.000000000000  ,  \"Imoff\"-> 0.000000000000  |>   , \r\"IDS0189_210310_RAW_cal__ref_\" ->   <| \"ζ\"->  0.040584680050  , \"τ1\"-> 0.030359591877  , \"τS\"-> 0.019792901852  , \"τN\"-> 0.005324821183  , \"τC\"-> 0.002700986774  , \"κ0\"-> 0.000000002671  , \"mm1\"-> 0.000000000000  , \"mm2\"-> 0.000000000000  , \"mm3\"-> 0.000000000000  , \"T\"->  0.430000000000  , \"B\"-> 12.000000000000  , \"θ\"-> 90.000000000000  , \"Reoff\"-> 0.000000000000  ,  \"Imoff\"-> 0.000000000000  |>   , \r\"IDS0189_210310_RAW_cal__sam_\" ->   <| \"ζ\"->  0.032748569996  , \"τ1\"-> 0.031072007290  , \"τS\"-> 0.024343937548  , \"τN\"-> 0.006961654481  , \"τC\"-> 0.002967111565  , \"κ0\"-> 0.000000002964  , \"mm1\"-> 0.000000000000  , \"mm2\"-> 0.000000000000  , \"mm3\"-> 0.000000000000  , \"T\"->  0.430000000000  , \"B\"-> 12.000000000000  , \"θ\"-> 90.000000000000  , \"Reoff\"-> 0.000000000000  ,  \"Imoff\"-> 0.000000000000  |>   , \r\"IDS0190_210310_RAW_cal__ref_\" ->   <| \"ζ\"->  0.030700897923  , \"τ1\"-> 0.026935085078  , \"τS\"-> 0.018364864329  , \"τN\"-> 0.002898516959  , \"τC\"-> 0.003150649099  , \"κ0\"-> 0.000000003342  , \"mm1\"-> 0.000000000000  , \"mm2\"-> 0.000000000000  , \"mm3\"-> 0.000000000000  , \"T\"->  0.512000000000  , \"B\"-> 12.000000000000  , \"θ\"-> 90.000000000000  , \"Reoff\"-> 0.000000000000  ,  \"Imoff\"-> 0.000000000000  |>   , \r\"IDS0190_210310_RAW_cal__sam_\" ->   <| \"ζ\"->  0.027599263457  , \"τ1\"-> 0.026239105728  , \"τS\"-> 0.022370859308  , \"τN\"-> 0.003857632966  , \"τC\"-> 0.003499360499  , \"κ0\"-> 0.000000003681  , \"mm1\"-> 0.000000000000  , \"mm2\"-> 0.000000000000  , \"mm3\"-> 0.000000000000  , \"T\"->  0.512000000000  , \"B\"-> 12.000000000000  , \"θ\"-> 90.000000000000  , \"Reoff\"-> 0.000000000000  ,  \"Imoff\"-> 0.000000000000  |>   , \r\"IDS0191_210310_RAW_cal__ref_\" ->   <| \"ζ\"->  0.025322625458  , \"τ1\"-> 0.023401812401  , \"τS\"-> 0.017347416709  , \"τN\"-> 0.002020498851  , \"τC\"-> 0.003594259467  , \"κ0\"-> 0.000000003970  , \"mm1\"-> 0.000000000000  , \"mm2\"-> 0.000000000000  , \"mm3\"-> 0.000000000000  , \"T\"->  0.610000000000  , \"B\"-> 12.000000000000  , \"θ\"-> 90.000000000000  , \"Reoff\"-> 0.000000000000  ,  \"Imoff\"-> 0.000000000000  |>   , \r\"IDS0191_210310_RAW_cal__sam_\" ->   <| \"ζ\"->  0.020568815513  , \"τ1\"-> 0.023045965648  , \"τS\"-> 0.020791387386  , \"τN\"-> 0.002229171297  , \"τC\"-> 0.004427475438  , \"κ0\"-> 0.000000004398  , \"mm1\"-> 0.000000000000  , \"mm2\"-> 0.000000000000  , \"mm3\"-> 0.000000000000  , \"T\"->  0.610000000000  , \"B\"-> 12.000000000000  , \"θ\"-> 90.000000000000  , \"Reoff\"-> 0.000000000000  ,  \"Imoff\"-> 0.000000000000  |>   , \r\"IDS0192_210310_RAW_cal__ref_\" ->   <| \"ζ\"->  0.022100596026  , \"τ1\"-> 0.020519097823  , \"τS\"-> 0.015555141042  , \"τN\"-> 0.000889956832  , \"τC\"-> 0.004354791503  , \"κ0\"-> 0.000000005560  , \"mm1\"-> 0.000000000000  , \"mm2\"-> 0.000000000000  , \"mm3\"-> 0.000000000000  , \"T\"->  0.810000000000  , \"B\"-> 12.000000000000  , \"θ\"-> 90.000000000000  , \"Reoff\"-> 0.000000000000  ,  \"Imoff\"-> 0.000000000000  |>   , \r\"IDS0192_210310_RAW_cal__sam_\" ->   <| \"ζ\"->  0.016548170999  , \"τ1\"-> 0.020108887890  , \"τS\"-> 0.018558394948  , \"τN\"-> 0.001160732495  , \"τC\"-> 0.004746126241  , \"κ0\"-> 0.000000005882  , \"mm1\"-> 0.000000000000  , \"mm2\"-> 0.000000000000  , \"mm3\"-> 0.000000000000  , \"T\"->  0.810000000000  , \"B\"-> 12.000000000000  , \"θ\"-> 90.000000000000  , \"Reoff\"-> 0.000000000000  ,  \"Imoff\"-> 0.000000000000  |>   , \r\"IDS0193_210310_RAW_cal__ref_\" ->   <| \"ζ\"->  0.020969814378  , \"τ1\"-> 0.020016820130  , \"τS\"-> 0.013372894745  , \"τN\"-> 0.000454586591  , \"τC\"-> 0.005292751338  , \"κ0\"-> 0.000000007771  , \"mm1\"-> 0.000000000000  , \"mm2\"-> 0.000000000000  , \"mm3\"-> 0.000000000000  , \"T\"->  1.100000000000  , \"B\"-> 12.000000000000  , \"θ\"-> 90.000000000000  , \"Reoff\"-> 0.000000000000  ,  \"Imoff\"-> 0.000000000000  |>   , \r\"IDS0193_210310_RAW_cal__sam_\" ->   <| \"ζ\"->  0.014495870556  , \"τ1\"-> 0.019990087457  , \"τS\"-> 0.016832201384  , \"τN\"-> 0.000455517238  , \"τC\"-> 0.005555782498  , \"κ0\"-> 0.000000008420  , \"mm1\"-> 0.000000000000  , \"mm2\"-> 0.000000000000  , \"mm3\"-> 0.000000000000  , \"T\"->  1.100000000000  , \"B\"-> 12.000000000000  , \"θ\"-> 90.000000000000  , \"Reoff\"-> 0.000000000000  ,  \"Imoff\"-> 0.000000000000  |>   , \r\"IDS0194_210310_RAW_cal__ref_\" ->   <| \"ζ\"->  0.020900896759  , \"τ1\"-> 0.018288874472  , \"τS\"-> 0.009095511262  , \"τN\"-> 0.000107884456  , \"τC\"-> 0.006896232004  , \"κ0\"-> 0.000000013449  , \"mm1\"-> 0.000000000000  , \"mm2\"-> 0.000000000000  , \"mm3\"-> 0.000000000000  , \"T\"->  1.800000000000  , \"B\"-> 12.000000000000  , \"θ\"-> 90.000000000000  , \"Reoff\"-> 0.000000000000  ,  \"Imoff\"-> 0.000000000000  |>   , \r\"IDS0194_210310_RAW_cal__sam_\" ->   <| \"ζ\"->  0.014043763709  , \"τ1\"-> 0.018292068543  , \"τS\"-> 0.011311396743  , \"τN\"-> 0.000128802259  , \"τC\"-> 0.008087849636  , \"κ0\"-> 0.000000014258  , \"mm1\"-> 0.000000000000  , \"mm2\"-> 0.000000000000  , \"mm3\"-> 0.000000000000  , \"T\"->  1.800000000000  , \"B\"-> 12.000000000000  , \"θ\"-> 90.000000000000  , \"Reoff\"-> 0.000000000000  ,  \"Imoff\"-> 0.000000000000  |>   , \r\"IDS0195_210310_RAW_cal__ref_\" ->   <| \"ζ\"->  0.019765118173  , \"τ1\"-> 0.018324978618  , \"τS\"-> 0.006054329354  , \"τN\"-> 0.000028420666  , \"τC\"-> 0.006398306925  , \"κ0\"-> 0.000000023958  , \"mm1\"-> 0.000000000000  , \"mm2\"-> 0.000000000000  , \"mm3\"-> 0.000000000000  , \"T\"->  3.000000000000  , \"B\"-> 12.000000000000  , \"θ\"-> 90.000000000000  , \"Reoff\"-> 0.000000000000  ,  \"Imoff\"-> 0.000000000000  |>   , \r\"IDS0195_210310_RAW_cal__sam_\" ->   <| \"ζ\"->  0.016187684631  , \"τ1\"-> 0.018325345271  , \"τS\"-> 0.007510087776  , \"τN\"-> 0.000028419157  , \"τC\"-> 0.008115463080  , \"κ0\"-> 0.000000024747  , \"mm1\"-> 0.000000000000  , \"mm2\"-> 0.000000000000  , \"mm3\"-> 0.000000000000  , \"T\"->  3.000000000000  , \"B\"-> 12.000000000000  , \"θ\"-> 90.000000000000  , \"Reoff\"-> 0.000000000000  ,  \"Imoff\"-> 0.000000000000  |>   , \r\"IDS0196_210310_RAW_cal__ref_\" ->   <| \"ζ\"->  0.030164668817  , \"τ1\"-> 0.012822215558  , \"τS\"-> 0.004108197943  , \"τN\"-> 0.000006999504  , \"τC\"-> 0.004420975765  , \"κ0\"-> 0.000000058872  , \"mm1\"-> 0.000000000000  , \"mm2\"-> 0.000000000000  , \"mm3\"-> 0.000000000000  , \"T\"->  5.700000000000  , \"B\"-> 12.000000000000  , \"θ\"-> 90.000000000000  , \"Reoff\"-> 0.000000000000  ,  \"Imoff\"-> 0.000000000000  |>   , \r\"IDS0196_210310_RAW_cal__sam_\" ->   <| \"ζ\"->  0.027897403691  , \"τ1\"-> 0.014639690770  , \"τS\"-> 0.004105291179  , \"τN\"-> 0.000006999171  , \"τC\"-> 0.007414449545  , \"κ0\"-> 0.000000059701  , \"mm1\"-> 0.000000000000  , \"mm2\"-> 0.000000000000  , \"mm3\"-> 0.000000000000  , \"T\"->  5.700000000000  , \"B\"-> 12.000000000000  , \"θ\"-> 90.000000000000  , \"Reoff\"-> 0.000000000000  ,  \"Imoff\"-> 0.000000000000  |>   , \r\"IDS0208_210310_RAW_cal__ref_\" ->   <| \"ζ\"->  0.000000000000  , \"τ1\"-> 0.000000000000  , \"τS\"-> 0.000000000000  , \"τN\"-> 0.000000000000  , \"τC\"-> 0.000000000000  , \"κ0\"-> 0.000000000000  , \"mm1\"-> 0.000000000000  , \"mm2\"-> 0.000000000000  , \"mm3\"-> 0.000000000000  , \"T\"->  0.197000000000  , \"B\"-> 0.000000000000  , \"θ\"-> 0.000000000000  , \"Reoff\"-> 0.000000000000  ,  \"Imoff\"-> 0.000000000000  |>   , \r\"IDS0208_210310_RAW_cal__sam_\" ->   <| \"ζ\"->  0.000000000000  , \"τ1\"-> 0.000000000000  , \"τS\"-> 0.000000000000  , \"τN\"-> 0.000000000000  , \"τC\"-> 0.000000000000  , \"κ0\"-> 0.000000000000  , \"mm1\"-> 0.000000000000  , \"mm2\"-> 0.000000000000  , \"mm3\"-> 0.000000000000  , \"T\"->  0.197000000000  , \"B\"-> 0.000000000000  , \"θ\"-> 0.000000000000  , \"Reoff\"-> 0.000000000000  ,  \"Imoff\"-> 0.000000000000  |>   , \r\"IDS0209_210310_RAW_cal__ref_\" ->   <| \"ζ\"->  0.163571654798  , \"τ1\"-> 0.020520714675  , \"τS\"-> 0.073117323271  , \"τN\"-> 0.020627224399  , \"τC\"-> 0.001336341391  , \"κ0\"-> 0.000000001061  , \"mm1\"-> 0.000000000000  , \"mm2\"-> 0.000000000000  , \"mm3\"-> 0.000000000000  , \"T\"->  0.197000000000  , \"B\"-> 0.000000000000  , \"θ\"-> 0.000000000000  , \"Reoff\"-> 0.000000000000  ,  \"Imoff\"-> 0.000000000000  |>   , \r\"IDS0209_210310_RAW_cal__sam_\" ->   <| \"ζ\"->  0.132901556203  , \"τ1\"-> 0.022795175616  , \"τS\"-> 0.082481385864  , \"τN\"-> 0.041432545456  , \"τC\"-> 0.001408424074  , \"κ0\"-> 0.000000001182  , \"mm1\"-> 0.000000000000  , \"mm2\"-> 0.000000000000  , \"mm3\"-> 0.000000000000  , \"T\"->  0.197000000000  , \"B\"-> 0.000000000000  , \"θ\"-> 0.000000000000  , \"Reoff\"-> 0.000000000000  ,  \"Imoff\"-> 0.000000000000  |>   , \r\"IDS0210_210310_RAW_cal__ref_\" ->   <| \"ζ\"->  0.000000000000  , \"τ1\"-> 0.000000000000  , \"τS\"-> 0.000000000000  , \"τN\"-> 0.000000000000  , \"τC\"-> 0.000000000000  , \"κ0\"-> 0.000000000000  , \"mm1\"-> 0.000000000000  , \"mm2\"-> 0.000000000000  , \"mm3\"-> 0.000000000000  , \"T\"->  0.148000000000  , \"B\"-> 6.000000000000  , \"θ\"-> 0.000000000000  , \"Reoff\"-> 0.000000000000  ,  \"Imoff\"-> 0.000000000000  |>   , \r\"IDS0210_210310_RAW_cal__sam_\" ->   <| \"ζ\"->  0.000000000000  , \"τ1\"-> 0.000000000000  , \"τS\"-> 0.000000000000  , \"τN\"-> 0.000000000000  , \"τC\"-> 0.000000000000  , \"κ0\"-> 0.000000000000  , \"mm1\"-> 0.000000000000  , \"mm2\"-> 0.000000000000  , \"mm3\"-> 0.000000000000  , \"T\"->  0.148000000000  , \"B\"-> 6.000000000000  , \"θ\"-> 0.000000000000  , \"Reoff\"-> 0.000000000000  ,  \"Imoff\"-> 0.000000000000  |>   , \r\"IDS0211_210310_RAW_cal__ref_\" ->   <| \"ζ\"->  0.160882265826  , \"τ1\"-> 0.034919932965  , \"τS\"-> 0.043973777096  , \"τN\"-> 0.047289018614  , \"τC\"-> 0.001339652100  , \"κ0\"-> 0.000000001069  , \"mm1\"-> 0.000000000000  , \"mm2\"-> 0.000000000000  , \"mm3\"-> 0.000000000000  , \"T\"->  0.197000000000  , \"B\"-> 9.000000000000  , \"θ\"-> 0.000000000000  , \"Reoff\"-> 0.000000000000  ,  \"Imoff\"-> 0.000000000000  |>   , \r\"IDS0211_210310_RAW_cal__sam_\" ->   <| \"ζ\"->  0.132534999612  , \"τ1\"-> 0.042581417401  , \"τS\"-> 0.054103824371  , \"τN\"-> 0.072163013930  , \"τC\"-> 0.001421040158  , \"κ0\"-> 0.000000001190  , \"mm1\"-> 0.000000000000  , \"mm2\"-> 0.000000000000  , \"mm3\"-> 0.000000000000  , \"T\"->  0.197000000000  , \"B\"-> 9.000000000000  , \"θ\"-> 0.000000000000  , \"Reoff\"-> 0.000000000000  ,  \"Imoff\"-> 0.000000000000  |>   , \r\"IDS0212_210310_RAW_cal__ref_\" ->   <| \"ζ\"->  0.154351103049  , \"τ1\"-> 0.051844552801  , \"τS\"-> 0.034651211615  , \"τN\"-> 0.065884588100  , \"τC\"-> 0.001166375427  , \"κ0\"-> 0.000000001084  , \"mm1\"-> 0.000000000000  , \"mm2\"-> 0.000000000000  , \"mm3\"-> 0.000000000000  , \"T\"->  0.197000000000  , \"B\"-> 11.000000000000  , \"θ\"-> 0.000000000000  , \"Reoff\"-> 0.000000000000  ,  \"Imoff\"-> 0.000000000000  |>   , \r\"IDS0212_210310_RAW_cal__sam_\" ->   <| \"ζ\"->  0.124414912597  , \"τ1\"-> 0.052685716706  , \"τS\"-> 0.041788480794  , \"τN\"-> 0.092820346766  , \"τC\"-> 0.001183564004  , \"κ0\"-> 0.000000001217  , \"mm1\"-> 0.000000000000  , \"mm2\"-> 0.000000000000  , \"mm3\"-> 0.000000000000  , \"T\"->  0.197000000000  , \"B\"-> 11.000000000000  , \"θ\"-> 0.000000000000  , \"Reoff\"-> 0.000000000000  ,  \"Imoff\"-> 0.000000000000  |>   , \r\"IDS0213_210310_RAW_cal__ref_\" ->   <| \"ζ\"->  0.158514180755  , \"τ1\"-> 0.046388884826  , \"τS\"-> 0.038847986012  , \"τN\"-> 0.058494864948  , \"τC\"-> 0.001325817289  , \"κ0\"-> 0.000000001072  , \"mm1\"-> 0.000000000000  , \"mm2\"-> 0.000000000000  , \"mm3\"-> 0.000000000000  , \"T\"->  0.197000000000  , \"B\"-> 10.000000000000  , \"θ\"-> 0.000000000000  , \"Reoff\"-> 0.000000000000  ,  \"Imoff\"-> 0.000000000000  |>   , \r\"IDS0213_210310_RAW_cal__sam_\" ->   <| \"ζ\"->  0.130083148284  , \"τ1\"-> 0.046211117525  , \"τS\"-> 0.046173592526  , \"τN\"-> 0.081942172735  , \"τC\"-> 0.001380184863  , \"κ0\"-> 0.000000001209  , \"mm1\"-> 0.000000000000  , \"mm2\"-> 0.000000000000  , \"mm3\"-> 0.000000000000  , \"T\"->  0.197000000000  , \"B\"-> 10.000000000000  , \"θ\"-> 0.000000000000  , \"Reoff\"-> 0.000000000000  ,  \"Imoff\"-> 0.000000000000  |>   , \r\"IDS0214_210310_RAW_cal__ref_\" ->   <| \"ζ\"->  0.154362032240  , \"τ1\"-> 0.030258273194  , \"τS\"-> 0.049523350330  , \"τN\"-> 0.040015703513  , \"τC\"-> 0.001328953616  , \"κ0\"-> 0.000000001075  , \"mm1\"-> 0.000000000000  , \"mm2\"-> 0.000000000000  , \"mm3\"-> 0.000000000000  , \"T\"->  0.197000000000  , \"B\"-> 8.000000000000  , \"θ\"-> 0.000000000000  , \"Reoff\"-> 0.000000000000  ,  \"Imoff\"-> 0.000000000000  |>   , \r\"IDS0214_210310_RAW_cal__sam_\" ->   <| \"ζ\"->  0.126440702434  , \"τ1\"-> 0.034118036572  , \"τS\"-> 0.060921114440  , \"τN\"-> 0.059832148427  , \"τC\"-> 0.001404471084  , \"κ0\"-> 0.000000001199  , \"mm1\"-> 0.000000000000  , \"mm2\"-> 0.000000000000  , \"mm3\"-> 0.000000000000  , \"T\"->  0.197000000000  , \"B\"-> 8.000000000000  , \"θ\"-> 0.000000000000  , \"Reoff\"-> 0.000000000000  ,  \"Imoff\"-> 0.000000000000  |>   , \r\"IDS0215_210310_RAW_cal__ref_\" ->   <| \"ζ\"->  0.162645417184  , \"τ1\"-> 0.023693851446  , \"τS\"-> 0.062400062170  , \"τN\"-> 0.026326088223  , \"τC\"-> 0.001322053294  , \"κ0\"-> 0.000000001070  , \"mm1\"-> 0.000000000000  , \"mm2\"-> 0.000000000000  , \"mm3\"-> 0.000000000000  , \"T\"->  0.197000000000  , \"B\"-> 7.000000000000  , \"θ\"-> 0.000000000000  , \"Reoff\"-> 0.000000000000  ,  \"Imoff\"-> 0.000000000000  |>   , \r\"IDS0215_210310_RAW_cal__sam_\" ->   <| \"ζ\"->  0.131383255045  , \"τ1\"-> 0.026827335842  , \"τS\"-> 0.071725959535  , \"τN\"-> 0.047510049318  , \"τC\"-> 0.001407613780  , \"κ0\"-> 0.000000001187  , \"mm1\"-> 0.000000000000  , \"mm2\"-> 0.000000000000  , \"mm3\"-> 0.000000000000  , \"T\"->  0.197000000000  , \"B\"-> 7.000000000000  , \"θ\"-> 0.000000000000  , \"Reoff\"-> 0.000000000000  ,  \"Imoff\"-> 0.000000000000  |>   , \r\"IDS0216_210310_RAW_cal__ref_\" ->   <| \"ζ\"->  0.149904026692  , \"τ1\"-> 0.020347243982  , \"τS\"-> 0.075273674904  , \"τN\"-> 0.020640082408  , \"τC\"-> 0.001432916876  , \"κ0\"-> 0.000000001050  , \"mm1\"-> 0.000000000000  , \"mm2\"-> 0.000000000000  , \"mm3\"-> 0.000000000000  , \"T\"->  0.197000000000  , \"B\"-> 5.000000000000  , \"θ\"-> 0.000000000000  , \"Reoff\"-> 0.000000000000  ,  \"Imoff\"-> 0.000000000000  |>   , \r\"IDS0216_210310_RAW_cal__sam_\" ->   <| \"ζ\"->  0.125455081262  , \"τ1\"-> 0.021777951907  , \"τS\"-> 0.089086097551  , \"τN\"-> 0.033580911935  , \"τC\"-> 0.001437991682  , \"κ0\"-> 0.000000001167  , \"mm1\"-> 0.000000000000  , \"mm2\"-> 0.000000000000  , \"mm3\"-> 0.000000000000  , \"T\"->  0.197000000000  , \"B\"-> 5.000000000000  , \"θ\"-> 0.000000000000  , \"Reoff\"-> 0.000000000000  ,  \"Imoff\"-> 0.000000000000  |>   , \r\"IDS0217_210310_RAW_cal__ref_\" ->   <| \"ζ\"->  0.121305227705  , \"τ1\"-> 0.032098202143  , \"τS\"-> 0.011865067519  , \"τN\"-> 0.005878702730  , \"τC\"-> 0.002147559783  , \"κ0\"-> 0.000000001032  , \"mm1\"-> 0.000000000000  , \"mm2\"-> 0.000000000000  , \"mm3\"-> 0.000000000000  , \"T\"->  0.197000000000  , \"B\"-> 0.000000000000  , \"θ\"-> 0.000000000000  , \"Reoff\"-> 0.000000000000  ,  \"Imoff\"-> 0.000000000000  |>   , \r\"IDS0217_210310_RAW_cal__sam_\" ->   <| \"ζ\"->  0.101804363109  , \"τ1\"-> 0.031947692776  , \"τS\"-> 0.014125667853  , \"τN\"-> 0.006009042128  , \"τC\"-> 0.002323789932  , \"κ0\"-> 0.000000001168  , \"mm1\"-> 0.000000000000  , \"mm2\"-> 0.000000000000  , \"mm3\"-> 0.000000000000  , \"T\"->  0.197000000000  , \"B\"-> 0.000000000000  , \"θ\"-> 0.000000000000  , \"Reoff\"-> 0.000000000000  ,  \"Imoff\"-> 0.000000000000  |>   , \r\"IDS0218_210310_RAW_cal__ref_\" ->   <| \"ζ\"->  0.000000000000  , \"τ1\"-> 0.000000000000  , \"τS\"-> 0.000000000000  , \"τN\"-> 0.000000000000  , \"τC\"-> 0.000000000000  , \"κ0\"-> 0.000000000000  , \"mm1\"-> 0.000000000000  , \"mm2\"-> 0.000000000000  , \"mm3\"-> 0.000000000000  , \"T\"->  1.550000000000  , \"B\"-> 0.000000000000  , \"θ\"-> 0.000000000000  , \"Reoff\"-> 0.000000000000  ,  \"Imoff\"-> 0.000000000000  |>   , \r\"IDS0218_210310_RAW_cal__sam_\" ->   <| \"ζ\"->  0.000000000000  , \"τ1\"-> 0.000000000000  , \"τS\"-> 0.000000000000  , \"τN\"-> 0.000000000000  , \"τC\"-> 0.000000000000  , \"κ0\"-> 0.000000000000  , \"mm1\"-> 0.000000000000  , \"mm2\"-> 0.000000000000  , \"mm3\"-> 0.000000000000  , \"T\"->  1.550000000000  , \"B\"-> 0.000000000000  , \"θ\"-> 0.000000000000  , \"Reoff\"-> 0.000000000000  ,  \"Imoff\"-> 0.000000000000  |>   , \r\"IDS0219_210310_RAW_cal__ref_\" ->   <| \"ζ\"->  0.000000000000  , \"τ1\"-> 0.000000000000  , \"τS\"-> 0.000000000000  , \"τN\"-> 0.000000000000  , \"τC\"-> 0.000000000000  , \"κ0\"-> 0.000000000000  , \"mm1\"-> 0.000000000000  , \"mm2\"-> 0.000000000000  , \"mm3\"-> 0.000000000000  , \"T\"->  1.000000000000  , \"B\"-> 0.000000000000  , \"θ\"-> 0.000000000000  , \"Reoff\"-> 0.000000000000  ,  \"Imoff\"-> 0.000000000000  |>   , \r\"IDS0219_210310_RAW_cal__sam_\" ->   <| \"ζ\"->  0.000000000000  , \"τ1\"-> 0.000000000000  , \"τS\"-> 0.000000000000  , \"τN\"-> 0.000000000000  , \"τC\"-> 0.000000000000  , \"κ0\"-> 0.000000000000  , \"mm1\"-> 0.000000000000  , \"mm2\"-> 0.000000000000  , \"mm3\"-> 0.000000000000  , \"T\"->  1.000000000000  , \"B\"-> 0.000000000000  , \"θ\"-> 0.000000000000  , \"Reoff\"-> 0.000000000000  ,  \"Imoff\"-> 0.000000000000  |>   , \r\"IDS0220_210310_RAW_cal__ref_\" ->   <| \"ζ\"->  0.000000000000  , \"τ1\"-> 0.000000000000  , \"τS\"-> 0.000000000000  , \"τN\"-> 0.000000000000  , \"τC\"-> 0.000000000000  , \"κ0\"-> 0.000000000000  , \"mm1\"-> 0.000000000000  , \"mm2\"-> 0.000000000000  , \"mm3\"-> 0.000000000000  , \"T\"->  0.677000000000  , \"B\"-> 0.000000000000  , \"θ\"-> 0.000000000000  , \"Reoff\"-> 0.000000000000  ,  \"Imoff\"-> 0.000000000000  |>   , \r\"IDS0220_210310_RAW_cal__sam_\" ->   <| \"ζ\"->  0.000000000000  , \"τ1\"-> 0.000000000000  , \"τS\"-> 0.000000000000  , \"τN\"-> 0.000000000000  , \"τC\"-> 0.000000000000  , \"κ0\"-> 0.000000000000  , \"mm1\"-> 0.000000000000  , \"mm2\"-> 0.000000000000  , \"mm3\"-> 0.000000000000  , \"T\"->  0.677000000000  , \"B\"-> 0.000000000000  , \"θ\"-> 0.000000000000  , \"Reoff\"-> 0.000000000000  ,  \"Imoff\"-> 0.000000000000  |>   , \r\"IDS0224_210310_RAW_cal__ref_\" ->   <| \"ζ\"->  0.000000000000  , \"τ1\"-> 0.000000000000  , \"τS\"-> 0.000000000000  , \"τN\"-> 0.000000000000  , \"τC\"-> 0.000000000000  , \"κ0\"-> 0.000000000000  , \"mm1\"-> 0.000000000000  , \"mm2\"-> 0.000000000000  , \"mm3\"-> 0.000000000000  , \"T\"->  0.000000000000  , \"B\"-> 0.000000000000  , \"θ\"-> 0.000000000000  , \"Reoff\"-> 0.000000000000  ,  \"Imoff\"-> 0.000000000000  |>   , \r\"IDS0224_210310_RAW_cal__sam_\" ->   <| \"ζ\"->  0.000000000000  , \"τ1\"-> 0.000000000000  , \"τS\"-> 0.000000000000  , \"τN\"-> 0.000000000000  , \"τC\"-> 0.000000000000  , \"κ0\"-> 0.000000000000  , \"mm1\"-> 0.000000000000  , \"mm2\"-> 0.000000000000  , \"mm3\"-> 0.000000000000  , \"T\"->  0.000000000000  , \"B\"-> 0.000000000000  , \"θ\"-> 0.000000000000  , \"Reoff\"-> 0.000000000000  ,  \"Imoff\"-> 0.000000000000  |>   , \r\"IDS0293_210427_RAW_cal__ref_\" ->   <| \"ζ\"->  0.016384838586  , \"τ1\"-> 0.013784349529  , \"τS\"-> 0.011495286759  , \"τN\"-> 0.000117117954  , \"τC\"-> 0.004048153799  , \"κ0\"-> 0.000000013122  , \"mm1\"-> 0.000000000000  , \"mm2\"-> 0.000000000000  , \"mm3\"-> 0.000000000000  , \"T\"->  1.900000000000  , \"B\"-> 12.000000000000  , \"θ\"-> 30.000000000000  , \"Reoff\"-> 0.000000000000  ,  \"Imoff\"-> 0.000000000000  |>   , \r\"IDS0293_210427_RAW_cal__sam_\" ->   <| \"ζ\"->  0.009772435939  , \"τ1\"-> 0.020827345370  , \"τS\"-> 0.013809334085  , \"τN\"-> 0.000168485133  , \"τC\"-> 0.005555066716  , \"κ0\"-> 0.000000013930  , \"mm1\"-> 0.000000000000  , \"mm2\"-> 0.000000000000  , \"mm3\"-> 0.000000000000  , \"T\"->  1.900000000000  , \"B\"-> 12.000000000000  , \"θ\"-> 30.000000000000  , \"Reoff\"-> 0.000000000000  ,  \"Imoff\"-> 0.000000000000  |>   , \r\"IDS0294_210427_RAW_cal__ref_\" ->   <| \"ζ\"->  0.017975147456  , \"τ1\"-> 0.015573317032  , \"τS\"-> 0.016697357463  , \"τN\"-> 0.000401487663  , \"τC\"-> 0.004243374884  , \"κ0\"-> 0.000000007622  , \"mm1\"-> 0.000000000000  , \"mm2\"-> 0.000000000000  , \"mm3\"-> 0.000000000000  , \"T\"->  1.130000000000  , \"B\"-> 12.000000000000  , \"θ\"-> 30.000000000000  , \"Reoff\"-> 0.000000000000  ,  \"Imoff\"-> 0.000000000000  |>   , \r\"IDS0294_210427_RAW_cal__sam_\" ->   <| \"ζ\"->  0.010912011148  , \"τ1\"-> 0.020760977312  , \"τS\"-> 0.021106239637  , \"τN\"-> 0.000452316988  , \"τC\"-> 0.005003723454  , \"κ0\"-> 0.000000008194  , \"mm1\"-> 0.000000000000  , \"mm2\"-> 0.000000000000  , \"mm3\"-> 0.000000000000  , \"T\"->  1.130000000000  , \"B\"-> 12.000000000000  , \"θ\"-> 30.000000000000  , \"Reoff\"-> 0.000000000000  ,  \"Imoff\"-> 0.000000000000  |>   , \r\"IDS0295_210427_RAW_cal__ref_\" ->   <| \"ζ\"->  0.021360373560  , \"τ1\"-> 0.017226807214  , \"τS\"-> 0.021136224671  , \"τN\"-> 0.000857882935  , \"τC\"-> 0.004088468956  , \"κ0\"-> 0.000000005432  , \"mm1\"-> 0.000000000000  , \"mm2\"-> 0.000000000000  , \"mm3\"-> 0.000000000000  , \"T\"->  0.830000000000  , \"B\"-> 12.000000000000  , \"θ\"-> 30.000000000000  , \"Reoff\"-> 0.000000000000  ,  \"Imoff\"-> 0.000000000000  |>   , \r\"IDS0295_210427_RAW_cal__sam_\" ->   <| \"ζ\"->  0.013460153434  , \"τ1\"-> 0.020684726260  , \"τS\"-> 0.027140346721  , \"τN\"-> 0.000960302406  , \"τC\"-> 0.004517434882  , \"κ0\"-> 0.000000005889  , \"mm1\"-> 0.000000000000  , \"mm2\"-> 0.000000000000  , \"mm3\"-> 0.000000000000  , \"T\"->  0.830000000000  , \"B\"-> 12.000000000000  , \"θ\"-> 30.000000000000  , \"Reoff\"-> 0.000000000000  ,  \"Imoff\"-> 0.000000000000  |>   , \r\"IDS0296_210427_RAW_cal__ref_\" ->   <| \"ζ\"->  0.027756025784  , \"τ1\"-> 0.019742757718  , \"τS\"-> 0.026611973171  , \"τN\"-> 0.001398943183  , \"τC\"-> 0.003482574473  , \"κ0\"-> 0.000000003907  , \"mm1\"-> 0.000000000000  , \"mm2\"-> 0.000000000000  , \"mm3\"-> 0.000000000000  , \"T\"->  0.620000000000  , \"B\"-> 12.000000000000  , \"θ\"-> 30.000000000000  , \"Reoff\"-> 0.000000000000  ,  \"Imoff\"-> 0.000000000000  |>   , \r\"IDS0296_210427_RAW_cal__sam_\" ->   <| \"ζ\"->  0.016892016292  , \"τ1\"-> 0.020344757415  , \"τS\"-> 0.033845756966  , \"τN\"-> 0.001946817417  , \"τC\"-> 0.004013762913  , \"κ0\"-> 0.000000004252  , \"mm1\"-> 0.000000000000  , \"mm2\"-> 0.000000000000  , \"mm3\"-> 0.000000000000  , \"T\"->  0.620000000000  , \"B\"-> 12.000000000000  , \"θ\"-> 30.000000000000  , \"Reoff\"-> 0.000000000000  ,  \"Imoff\"-> 0.000000000000  |>   , \r\"IDS0297_210427_RAW_cal__ref_\" ->   <| \"ζ\"->  0.034775017342  , \"τ1\"-> 0.018923965005  , \"τS\"-> 0.030086686370  , \"τN\"-> 0.002286572055  , \"τC\"-> 0.002714831651  , \"κ0\"-> 0.000000003294  , \"mm1\"-> 0.000000000000  , \"mm2\"-> 0.000000000000  , \"mm3\"-> 0.000000000000  , \"T\"->  0.530000000000  , \"B\"-> 12.000000000000  , \"θ\"-> 30.000000000000  , \"Reoff\"-> 0.000000000000  ,  \"Imoff\"-> 0.000000000000  |>   , \r\"IDS0297_210427_RAW_cal__sam_\" ->   <| \"ζ\"->  0.021116250068  , \"τ1\"-> 0.020669239851  , \"τS\"-> 0.037941648749  , \"τN\"-> 0.003221866945  , \"τC\"-> 0.003619427775  , \"κ0\"-> 0.000000003553  , \"mm1\"-> 0.000000000000  , \"mm2\"-> 0.000000000000  , \"mm3\"-> 0.000000000000  , \"T\"->  0.530000000000  , \"B\"-> 12.000000000000  , \"θ\"-> 30.000000000000  , \"Reoff\"-> 0.000000000000  ,  \"Imoff\"-> 0.000000000000  |>   , \r\"IDS0298_210427_RAW_cal__ref_\" ->   <| \"ζ\"->  0.046396907778  , \"τ1\"-> 0.018912834926  , \"τS\"-> 0.034035556993  , \"τN\"-> 0.004466176128  , \"τC\"-> 0.002290347128  , \"κ0\"-> 0.000000002639  , \"mm1\"-> 0.000000000000  , \"mm2\"-> 0.000000000000  , \"mm3\"-> 0.000000000000  , \"T\"->  0.430000000000  , \"B\"-> 12.000000000000  , \"θ\"-> 30.000000000000  , \"Reoff\"-> 0.000000000000  ,  \"Imoff\"-> 0.000000000000  |>   , \r\"IDS0298_210427_RAW_cal__sam_\" ->   <| \"ζ\"->  0.028468689077  , \"τ1\"-> 0.020220821810  , \"τS\"-> 0.043529484347  , \"τN\"-> 0.005653540941  , \"τC\"-> 0.003150537442  , \"κ0\"-> 0.000000002855  , \"mm1\"-> 0.000000000000  , \"mm2\"-> 0.000000000000  , \"mm3\"-> 0.000000000000  , \"T\"->  0.430000000000  , \"B\"-> 12.000000000000  , \"θ\"-> 30.000000000000  , \"Reoff\"-> 0.000000000000  ,  \"Imoff\"-> 0.000000000000  |>   , \r\"IDS0299_210427_RAW_cal__ref_\" ->   <| \"ζ\"->  0.060257387765  , \"τ1\"-> 0.020933176342  , \"τS\"-> 0.038399909631  , \"τN\"-> 0.009014166994  , \"τC\"-> 0.001999715217  , \"κ0\"-> 0.000000002125  , \"mm1\"-> 0.000000000000  , \"mm2\"-> 0.000000000000  , \"mm3\"-> 0.000000000000  , \"T\"->  0.360000000000  , \"B\"-> 12.000000000000  , \"θ\"-> 30.000000000000  , \"Reoff\"-> 0.000000000000  ,  \"Imoff\"-> 0.000000000000  |>   , \r\"IDS0299_210427_RAW_cal__sam_\" ->   <| \"ζ\"->  0.036420486357  , \"τ1\"-> 0.020986681106  , \"τS\"-> 0.049149577509  , \"τN\"-> 0.011109585503  , \"τC\"-> 0.002819780093  , \"κ0\"-> 0.000000002299  , \"mm1\"-> 0.000000000000  , \"mm2\"-> 0.000000000000  , \"mm3\"-> 0.000000000000  , \"T\"->  0.360000000000  , \"B\"-> 12.000000000000  , \"θ\"-> 30.000000000000  , \"Reoff\"-> 0.000000000000  ,  \"Imoff\"-> 0.000000000000  |>   , \r\"IDS0300_210427_RAW_cal__ref_\" ->   <| \"ζ\"->  0.338385515343  , \"τ1\"-> 0.049005471612  , \"τS\"-> 0.154718584573  , \"τN\"-> 0.405362096342  , \"τC\"-> 0.001218418583  , \"κ0\"-> 0.000000000425  , \"mm1\"-> 0.000000000000  , \"mm2\"-> 0.000000000000  , \"mm3\"-> 0.000000000000  , \"T\"->  0.140000000000  , \"B\"-> 12.000000000000  , \"θ\"-> 30.000000000000  , \"Reoff\"-> 0.000000000000  ,  \"Imoff\"-> 0.000000000000  |>   , \r\"IDS0300_210427_RAW_cal__sam_\" ->   <| \"ζ\"->  0.211545693132  , \"τ1\"-> 0.029106147473  , \"τS\"-> 0.094475691604  , \"τN\"-> 0.369151052631  , \"τC\"-> 0.001396700790  , \"κ0\"-> 0.000000000537  , \"mm1\"-> 0.000000000000  , \"mm2\"-> 0.000000000000  , \"mm3\"-> 0.000000000000  , \"T\"->  0.140000000000  , \"B\"-> 12.000000000000  , \"θ\"-> 30.000000000000  , \"Reoff\"-> 0.000000000000  ,  \"Imoff\"-> 0.000000000000  |>   , \r\"IDS0301_210831_RAW_cal__ref_\" ->   <| \"ζ\"->  0.083856390991  , \"τ1\"-> 0.023882632275  , \"τS\"-> 0.042264558819  , \"τN\"-> 0.014926022610  , \"τC\"-> 0.001493479414  , \"κ0\"-> 0.000000001739  , \"mm1\"-> 0.000000000000  , \"mm2\"-> 0.000000000000  , \"mm3\"-> 0.000000000000  , \"T\"->  0.300000000000  , \"B\"-> 12.000000000000  , \"θ\"-> 30.000000000000  , \"Reoff\"-> 0.000000000000  ,  \"Imoff\"-> 0.000000000000  |>   , \r\"IDS0301_210831_RAW_cal__sam_\" ->   <| \"ζ\"->  0.050663808076  , \"τ1\"-> 0.024940898568  , \"τS\"-> 0.056803871413  , \"τN\"-> 0.018856862265  , \"τC\"-> 0.002133501904  , \"κ0\"-> 0.000000001888  , \"mm1\"-> 0.000000000000  , \"mm2\"-> 0.000000000000  , \"mm3\"-> 0.000000000000  , \"T\"->  0.300000000000  , \"B\"-> 12.000000000000  , \"θ\"-> 30.000000000000  , \"Reoff\"-> 0.000000000000  ,  \"Imoff\"-> 0.000000000000  |>   , \r\"IDS0302_210831_RAW_cal__ref_\" ->   <| \"ζ\"->  0.118191658932  , \"τ1\"-> 0.027786613255  , \"τS\"-> 0.049841575379  , \"τN\"-> 0.030683320319  , \"τC\"-> 0.001300754197  , \"κ0\"-> 0.000000001363  , \"mm1\"-> 0.000000000000  , \"mm2\"-> 0.000000000000  , \"mm3\"-> 0.000000000000  , \"T\"->  0.250000000000  , \"B\"-> 12.000000000000  , \"θ\"-> 30.000000000000  , \"Reoff\"-> 0.000000000000  ,  \"Imoff\"-> 0.000000000000  |>   , \r\"IDS0302_210831_RAW_cal__sam_\" ->   <| \"ζ\"->  0.072634365939  , \"τ1\"-> 0.028637109000  , \"τS\"-> 0.065061142288  , \"τN\"-> 0.040304243071  , \"τC\"-> 0.001622979999  , \"κ0\"-> 0.000000001498  , \"mm1\"-> 0.000000000000  , \"mm2\"-> 0.000000000000  , \"mm3\"-> 0.000000000000  , \"T\"->  0.250000000000  , \"B\"-> 12.000000000000  , \"θ\"-> 30.000000000000  , \"Reoff\"-> 0.000000000000  ,  \"Imoff\"-> 0.000000000000  |>   , \r\"IDS0303_210831_RAW_cal__ref_\" ->   <| \"ζ\"->  0.210185455037  , \"τ1\"-> 0.035884437188  , \"τS\"-> 0.076269858590  , \"τN\"-> 0.100000000000  , \"τC\"-> 0.001092094788  , \"κ0\"-> 0.000000001049  , \"mm1\"-> 0.000000000000  , \"mm2\"-> 0.000000000000  , \"mm3\"-> 0.000000000000  , \"T\"->  0.200000000000  , \"B\"-> 12.000000000000  , \"θ\"-> 30.000000000000  , \"Reoff\"-> 0.000000000000  ,  \"Imoff\"-> 0.000000000000  |>   , \r\"IDS0303_210831_RAW_cal__sam_\" ->   <| \"ζ\"->  0.128615765969  , \"τ1\"-> 0.032665502211  , \"τS\"-> 0.082694869013  , \"τN\"-> 0.105788373632  , \"τC\"-> 0.001439686784  , \"κ0\"-> 0.000000001168  , \"mm1\"-> 0.000000000000  , \"mm2\"-> 0.000000000000  , \"mm3\"-> 0.000000000000  , \"T\"->  0.200000000000  , \"B\"-> 12.000000000000  , \"θ\"-> 30.000000000000  , \"Reoff\"-> 0.000000000000  ,  \"Imoff\"-> 0.000000000000  |>   , \r\"IDS0304_210831_RAW_cal__ref_\" ->   <| \"ζ\"->  0.270205686716  , \"τ1\"-> 0.041964859676  , \"τS\"-> 0.093295997771  , \"τN\"-> 0.171907220186  , \"τC\"-> 0.001079705974  , \"κ0\"-> 0.000000000759  , \"mm1\"-> 0.000000000000  , \"mm2\"-> 0.000000000000  , \"mm3\"-> 0.000000000000  , \"T\"->  0.170000000000  , \"B\"-> 12.000000000000  , \"θ\"-> 30.000000000000  , \"Reoff\"-> 0.000000000000  ,  \"Imoff\"-> 0.000000000000  |>   , \r\"IDS0304_210831_RAW_cal__sam_\" ->   <| \"ζ\"->  0.156472219566  , \"τ1\"-> 0.031017925061  , \"τS\"-> 0.080872234530  , \"τN\"-> 0.219381306397  , \"τC\"-> 0.001437792153  , \"κ0\"-> 0.000000000867  , \"mm1\"-> 0.000000000000  , \"mm2\"-> 0.000000000000  , \"mm3\"-> 0.000000000000  , \"T\"->  0.170000000000  , \"B\"-> 12.000000000000  , \"θ\"-> 30.000000000000  , \"Reoff\"-> 0.000000000000  ,  \"Imoff\"-> 0.000000000000  |>   , \r\"IDS0305_210831_RAW_cal__ref_\" ->   <| \"ζ\"->  0.288872243536  , \"τ1\"-> 0.043051365220  , \"τS\"-> 0.113757726379  , \"τN\"-> 0.232280670982  , \"τC\"-> 0.001075362358  , \"κ0\"-> 0.000000000648  , \"mm1\"-> 0.000000000000  , \"mm2\"-> 0.000000000000  , \"mm3\"-> 0.000000000000  , \"T\"->  0.160000000000  , \"B\"-> 12.000000000000  , \"θ\"-> 30.000000000000  , \"Reoff\"-> 0.000000000000  ,  \"Imoff\"-> 0.000000000000  |>   , \r\"IDS0305_210831_RAW_cal__sam_\" ->   <| \"ζ\"->  0.162585495535  , \"τ1\"-> 0.037883389730  , \"τS\"-> 0.086562863191  , \"τN\"-> 0.241872534356  , \"τC\"-> 0.001506143871  , \"κ0\"-> 0.000000000791  , \"mm1\"-> 0.000000000000  , \"mm2\"-> 0.000000000000  , \"mm3\"-> 0.000000000000  , \"T\"->  0.160000000000  , \"B\"-> 12.000000000000  , \"θ\"-> 30.000000000000  , \"Reoff\"-> 0.000000000000  ,  \"Imoff\"-> 0.000000000000  |>   , \r\"IDS0306_210831_RAW_cal__ref_\" ->   <| \"ζ\"->  0.013593052641  , \"τ1\"-> 0.010989385662  , \"τS\"-> 0.007947176041  , \"τN\"-> 0.000037757079  , \"τC\"-> 0.003572854733  , \"κ0\"-> 0.000000023548  , \"mm1\"-> 0.000000000000  , \"mm2\"-> 0.000000000000  , \"mm3\"-> 0.000000000000  , \"T\"->  3.100000000000  , \"B\"-> 12.000000000000  , \"θ\"-> 30.000000000000  , \"Reoff\"-> 0.000000000000  ,  \"Imoff\"-> 0.000000000000  |>   , \r\"IDS0306_210831_RAW_cal__sam_\" ->   <| \"ζ\"->  0.010111127240  , \"τ1\"-> 0.020788755574  , \"τS\"-> 0.009968978424  , \"τN\"-> 0.000077788811  , \"τC\"-> 0.004598584548  , \"κ0\"-> 0.000000024346  , \"mm1\"-> 0.000000000000  , \"mm2\"-> 0.000000000000  , \"mm3\"-> 0.000000000000  , \"T\"->  3.100000000000  , \"B\"-> 12.000000000000  , \"θ\"-> 30.000000000000  , \"Reoff\"-> 0.000000000000  ,  \"Imoff\"-> 0.000000000000  |>   , \r\"IDS0310_210901_RAW_cal__ref_\" ->   <| \"ζ\"->  0.308289315544  , \"τ1\"-> 0.054346075620  , \"τS\"-> 0.066318547481  , \"τN\"-> 0.209207967486  , \"τC\"-> 0.001005266633  , \"κ0\"-> 0.000000000648  , \"mm1\"-> 0.000000000000  , \"mm2\"-> 0.000000000000  , \"mm3\"-> 0.000000000000  , \"T\"->  0.157000000000  , \"B\"-> 12.000000000000  , \"θ\"-> 45.000000000000  , \"Reoff\"-> 0.000000000000  ,  \"Imoff\"-> 0.000000000000  |>   , \r\"IDS0310_210901_RAW_cal__sam_\" ->   <| \"ζ\"->  0.295520923520  , \"τ1\"-> 0.054772440405  , \"τS\"-> 0.071814005451  , \"τN\"-> 0.249593767169  , \"τC\"-> 0.001103632155  , \"κ0\"-> 0.000000000625  , \"mm1\"-> 0.000000000000  , \"mm2\"-> 0.000000000000  , \"mm3\"-> 0.000000000000  , \"T\"->  0.157000000000  , \"B\"-> 12.000000000000  , \"θ\"-> 45.000000000000  , \"Reoff\"-> 0.000000000000  ,  \"Imoff\"-> 0.000000000000  |>   , \r\"IDS0311_210901_RAW_cal__ref_\" ->   <| \"ζ\"->  0.509291398058  , \"τ1\"-> 0.072489311123  , \"τS\"-> 0.090971238975  , \"τN\"-> 0.493344947632  , \"τC\"-> 0.000983845591  , \"κ0\"-> 0.000000000427  , \"mm1\"-> 0.000000000000  , \"mm2\"-> 0.000000000000  , \"mm3\"-> 0.000000000000  , \"T\"->  0.120000000000  , \"B\"-> 12.000000000000  , \"θ\"-> 45.000000000000  , \"Reoff\"-> 0.000000000000  ,  \"Imoff\"-> 0.000000000000  |>   , \r\"IDS0311_210901_RAW_cal__sam_\" ->   <| \"ζ\"->  0.523545279740  , \"τ1\"-> 0.065613539167  , \"τS\"-> 0.100000000000  , \"τN\"-> 0.424083114177  , \"τC\"-> 0.000911255863  , \"κ0\"-> 0.000000000418  , \"mm1\"-> 0.000000000000  , \"mm2\"-> 0.000000000000  , \"mm3\"-> 0.000000000000  , \"T\"->  0.120000000000  , \"B\"-> 12.000000000000  , \"θ\"-> 45.000000000000  , \"Reoff\"-> 0.000000000000  ,  \"Imoff\"-> 0.000000000000  |>   , \r\"IDS0312_210901_RAW_cal__ref_\" ->   <| \"ζ\"->  0.255987747016  , \"τ1\"-> 0.050915418179  , \"τS\"-> 0.056322890077  , \"τN\"-> 0.162539494258  , \"τC\"-> 0.001014478551  , \"κ0\"-> 0.000000000752  , \"mm1\"-> 0.000000000000  , \"mm2\"-> 0.000000000000  , \"mm3\"-> 0.000000000000  , \"T\"->  0.170000000000  , \"B\"-> 12.000000000000  , \"θ\"-> 45.000000000000  , \"Reoff\"-> 0.000000000000  ,  \"Imoff\"-> 0.000000000000  |>   , \r\"IDS0312_210901_RAW_cal__sam_\" ->   <| \"ζ\"->  0.273742116471  , \"τ1\"-> 0.052262909995  , \"τS\"-> 0.060554036646  , \"τN\"-> 0.154269705680  , \"τC\"-> 0.001074144337  , \"κ0\"-> 0.000000000753  , \"mm1\"-> 0.000000000000  , \"mm2\"-> 0.000000000000  , \"mm3\"-> 0.000000000000  , \"T\"->  0.170000000000  , \"B\"-> 12.000000000000  , \"θ\"-> 45.000000000000  , \"Reoff\"-> 0.000000000000  ,  \"Imoff\"-> 0.000000000000  |>   , \r\"IDS0313_210901_RAW_cal__ref_\" ->   <| \"ζ\"->  0.214174227031  , \"τ1\"-> 0.045371966885  , \"τS\"-> 0.046160741010  , \"τN\"-> 0.090352099204  , \"τC\"-> 0.001077653985  , \"κ0\"-> 0.000000001047  , \"mm1\"-> 0.000000000000  , \"mm2\"-> 0.000000000000  , \"mm3\"-> 0.000000000000  , \"T\"->  0.200000000000  , \"B\"-> 12.000000000000  , \"θ\"-> 45.000000000000  , \"Reoff\"-> 0.000000000000  ,  \"Imoff\"-> 0.000000000000  |>   , \r\"IDS0313_210901_RAW_cal__sam_\" ->   <| \"ζ\"->  0.215688135788  , \"τ1\"-> 0.043710888546  , \"τS\"-> 0.044756474141  , \"τN\"-> 0.090222547904  , \"τC\"-> 0.001049781785  , \"κ0\"-> 0.000000001047  , \"mm1\"-> 0.000000000000  , \"mm2\"-> 0.000000000000  , \"mm3\"-> 0.000000000000  , \"T\"->  0.200000000000  , \"B\"-> 12.000000000000  , \"θ\"-> 45.000000000000  , \"Reoff\"-> 0.000000000000  ,  \"Imoff\"-> 0.000000000000  |>   , \r\"IDS0314_210901_RAW_cal__ref_\" ->   <| \"ζ\"->  0.121938807235  , \"τ1\"-> 0.034207371807  , \"τS\"-> 0.036720955072  , \"τN\"-> 0.033836278502  , \"τC\"-> 0.001295467245  , \"κ0\"-> 0.000000001354  , \"mm1\"-> 0.000000000000  , \"mm2\"-> 0.000000000000  , \"mm3\"-> 0.000000000000  , \"T\"->  0.255000000000  , \"B\"-> 12.000000000000  , \"θ\"-> 45.000000000000  , \"Reoff\"-> 0.000000000000  ,  \"Imoff\"-> 0.000000000000  |>   , \r\"IDS0314_210901_RAW_cal__sam_\" ->   <| \"ζ\"->  0.118583992968  , \"τ1\"-> 0.035232851003  , \"τS\"-> 0.037458022816  , \"τN\"-> 0.033724509363  , \"τC\"-> 0.001440922263  , \"κ0\"-> 0.000000001360  , \"mm1\"-> 0.000000000000  , \"mm2\"-> 0.000000000000  , \"mm3\"-> 0.000000000000  , \"T\"->  0.255000000000  , \"B\"-> 12.000000000000  , \"θ\"-> 45.000000000000  , \"Reoff\"-> 0.000000000000  ,  \"Imoff\"-> 0.000000000000  |>   , \r\"IDS0315_210901_RAW_cal__ref_\" ->   <| \"ζ\"->  0.083994348522  , \"τ1\"-> 0.028454655874  , \"τS\"-> 0.032547522861  , \"τN\"-> 0.016695645368  , \"τC\"-> 0.001519868181  , \"κ0\"-> 0.000000001732  , \"mm1\"-> 0.000000000000  , \"mm2\"-> 0.000000000000  , \"mm3\"-> 0.000000000000  , \"T\"->  0.300000000000  , \"B\"-> 12.000000000000  , \"θ\"-> 45.000000000000  , \"Reoff\"-> 0.000000000000  ,  \"Imoff\"-> 0.000000000000  |>   , \r\"IDS0315_210901_RAW_cal__sam_\" ->   <| \"ζ\"->  0.085152769414  , \"τ1\"-> 0.029001116263  , \"τS\"-> 0.032604663993  , \"τN\"-> 0.016878763935  , \"τC\"-> 0.001443524845  , \"κ0\"-> 0.000000001728  , \"mm1\"-> 0.000000000000  , \"mm2\"-> 0.000000000000  , \"mm3\"-> 0.000000000000  , \"T\"->  0.300000000000  , \"B\"-> 12.000000000000  , \"θ\"-> 45.000000000000  , \"Reoff\"-> 0.000000000000  ,  \"Imoff\"-> 0.000000000000  |>   , \r\"IDS0316_210901_RAW_cal__ref_\" ->   <| \"ζ\"->  0.061161812807  , \"τ1\"-> 0.025679940958  , \"τS\"-> 0.030186846656  , \"τN\"-> 0.009745770789  , \"τC\"-> 0.001942458613  , \"κ0\"-> 0.000000002119  , \"mm1\"-> 0.000000000000  , \"mm2\"-> 0.000000000000  , \"mm3\"-> 0.000000000000  , \"T\"->  0.360000000000  , \"B\"-> 12.000000000000  , \"θ\"-> 45.000000000000  , \"Reoff\"-> 0.000000000000  ,  \"Imoff\"-> 0.000000000000  |>   , \r\"IDS0316_210901_RAW_cal__sam_\" ->   <| \"ζ\"->  0.061011838044  , \"τ1\"-> 0.025440548989  , \"τS\"-> 0.030028053978  , \"τN\"-> 0.010140731955  , \"τC\"-> 0.001895079687  , \"κ0\"-> 0.000000002115  , \"mm1\"-> 0.000000000000  , \"mm2\"-> 0.000000000000  , \"mm3\"-> 0.000000000000  , \"T\"->  0.360000000000  , \"B\"-> 12.000000000000  , \"θ\"-> 45.000000000000  , \"Reoff\"-> 0.000000000000  ,  \"Imoff\"-> 0.000000000000  |>   , \r\"IDS0317_210901_RAW_cal__ref_\" ->   <| \"ζ\"->  0.047188818117  , \"τ1\"-> 0.023281630947  , \"τS\"-> 0.027595934693  , \"τN\"-> 0.005357909158  , \"τC\"-> 0.002405018291  , \"κ0\"-> 0.000000002634  , \"mm1\"-> 0.000000000000  , \"mm2\"-> 0.000000000000  , \"mm3\"-> 0.000000000000  , \"T\"->  0.430000000000  , \"B\"-> 12.000000000000  , \"θ\"-> 45.000000000000  , \"Reoff\"-> 0.000000000000  ,  \"Imoff\"-> 0.000000000000  |>   , \r\"IDS0317_210901_RAW_cal__sam_\" ->   <| \"ζ\"->  0.046686299518  , \"τ1\"-> 0.021011215626  , \"τS\"-> 0.027633142317  , \"τN\"-> 0.005348477555  , \"τC\"-> 0.002098477650  , \"κ0\"-> 0.000000002635  , \"mm1\"-> 0.000000000000  , \"mm2\"-> 0.000000000000  , \"mm3\"-> 0.000000000000  , \"T\"->  0.430000000000  , \"B\"-> 12.000000000000  , \"θ\"-> 45.000000000000  , \"Reoff\"-> 0.000000000000  ,  \"Imoff\"-> 0.000000000000  |>   , \r\"IDS0318_210901_RAW_cal__ref_\" ->   <| \"ζ\"->  0.037288247068  , \"τ1\"-> 0.020701608824  , \"τS\"-> 0.025512873362  , \"τN\"-> 0.002622201076  , \"τC\"-> 0.002753838304  , \"κ0\"-> 0.000000003290  , \"mm1\"-> 0.000000000000  , \"mm2\"-> 0.000000000000  , \"mm3\"-> 0.000000000000  , \"T\"->  0.530000000000  , \"B\"-> 12.000000000000  , \"θ\"-> 45.000000000000  , \"Reoff\"-> 0.000000000000  ,  \"Imoff\"-> 0.000000000000  |>   , \r\"IDS0318_210901_RAW_cal__sam_\" ->   <| \"ζ\"->  0.035204330012  , \"τ1\"-> 0.021011523093  , \"τS\"-> 0.025247316079  , \"τN\"-> 0.002718647875  , \"τC\"-> 0.003091727575  , \"κ0\"-> 0.000000003296  , \"mm1\"-> 0.000000000000  , \"mm2\"-> 0.000000000000  , \"mm3\"-> 0.000000000000  , \"T\"->  0.530000000000  , \"B\"-> 12.000000000000  , \"θ\"-> 45.000000000000  , \"Reoff\"-> 0.000000000000  ,  \"Imoff\"-> 0.000000000000  |>   , \r\"IDS0319_210901_RAW_cal__ref_\" ->   <| \"ζ\"->  0.029057248634  , \"τ1\"-> 0.018506971535  , \"τS\"-> 0.023958337181  , \"τN\"-> 0.001609750825  , \"τC\"-> 0.003041346082  , \"κ0\"-> 0.000000003909  , \"mm1\"-> 0.000000000000  , \"mm2\"-> 0.000000000000  , \"mm3\"-> 0.000000000000  , \"T\"->  0.620000000000  , \"B\"-> 12.000000000000  , \"θ\"-> 45.000000000000  , \"Reoff\"-> 0.000000000000  ,  \"Imoff\"-> 0.000000000000  |>   , \r\"IDS0319_210901_RAW_cal__sam_\" ->   <| \"ζ\"->  0.030862035723  , \"τ1\"-> 0.019328530751  , \"τS\"-> 0.023568572597  , \"τN\"-> 0.001701966614  , \"τC\"-> 0.003453790534  , \"κ0\"-> 0.000000003906  , \"mm1\"-> 0.000000000000  , \"mm2\"-> 0.000000000000  , \"mm3\"-> 0.000000000000  , \"T\"->  0.620000000000  , \"B\"-> 12.000000000000  , \"θ\"-> 45.000000000000  , \"Reoff\"-> 0.000000000000  ,  \"Imoff\"-> 0.000000000000  |>   , \r\"IDS0320_210901_RAW_cal__ref_\" ->   <| \"ζ\"->  0.022379315068  , \"τ1\"-> 0.015662672554  , \"τS\"-> 0.020062485201  , \"τN\"-> 0.000750608517  , \"τC\"-> 0.004162319228  , \"κ0\"-> 0.000000005449  , \"mm1\"-> 0.000000000000  , \"mm2\"-> 0.000000000000  , \"mm3\"-> 0.000000000000  , \"T\"->  0.830000000000  , \"B\"-> 12.000000000000  , \"θ\"-> 45.000000000000  , \"Reoff\"-> 0.000000000000  ,  \"Imoff\"-> 0.000000000000  |>   , \r\"IDS0320_210901_RAW_cal__sam_\" ->   <| \"ζ\"->  0.023591124045  , \"τ1\"-> 0.014910006225  , \"τS\"-> 0.019342950404  , \"τN\"-> 0.000752972387  , \"τC\"-> 0.004900413232  , \"κ0\"-> 0.000000005453  , \"mm1\"-> 0.000000000000  , \"mm2\"-> 0.000000000000  , \"mm3\"-> 0.000000000000  , \"T\"->  0.830000000000  , \"B\"-> 12.000000000000  , \"θ\"-> 45.000000000000  , \"Reoff\"-> 0.000000000000  ,  \"Imoff\"-> 0.000000000000  |>   , \r\"IDS0321_210901_RAW_cal__ref_\" ->   <| \"ζ\"->  0.020614746765  , \"τ1\"-> 0.013682065369  , \"τS\"-> 0.016105139108  , \"τN\"-> 0.000397734649  , \"τC\"-> 0.005005824303  , \"κ0\"-> 0.000000007592  , \"mm1\"-> 0.000000000000  , \"mm2\"-> 0.000000000000  , \"mm3\"-> 0.000000000000  , \"T\"->  1.130000000000  , \"B\"-> 12.000000000000  , \"θ\"-> 45.000000000000  , \"Reoff\"-> 0.000000000000  ,  \"Imoff\"-> 0.000000000000  |>   , \r\"IDS0321_210901_RAW_cal__sam_\" ->   <| \"ζ\"->  0.020215154826  , \"τ1\"-> 0.014105227254  , \"τS\"-> 0.015660924043  , \"τN\"-> 0.000525137036  , \"τC\"-> 0.005447728357  , \"κ0\"-> 0.000000007594  , \"mm1\"-> 0.000000000000  , \"mm2\"-> 0.000000000000  , \"mm3\"-> 0.000000000000  , \"T\"->  1.130000000000  , \"B\"-> 12.000000000000  , \"θ\"-> 45.000000000000  , \"Reoff\"-> 0.000000000000  ,  \"Imoff\"-> 0.000000000000  |>   , \r\"IDS0322_210901_RAW_cal__ref_\" ->   <| \"ζ\"->  0.019557893298  , \"τ1\"-> 0.012446212333  , \"τS\"-> 0.011139553358  , \"τN\"-> 0.000114229396  , \"τC\"-> 0.005115315079  , \"κ0\"-> 0.000000013115  , \"mm1\"-> 0.000000000000  , \"mm2\"-> 0.000000000000  , \"mm3\"-> 0.000000000000  , \"T\"->  1.900000000000  , \"B\"-> 12.000000000000  , \"θ\"-> 45.000000000000  , \"Reoff\"-> 0.000000000000  ,  \"Imoff\"-> 0.000000000000  |>   , \r\"IDS0322_210901_RAW_cal__sam_\" ->   <| \"ζ\"->  0.018090572724  , \"τ1\"-> 0.013314780956  , \"τS\"-> 0.010820835010  , \"τN\"-> 0.000265552167  , \"τC\"-> 0.005393540417  , \"κ0\"-> 0.000000013100  , \"mm1\"-> 0.000000000000  , \"mm2\"-> 0.000000000000  , \"mm3\"-> 0.000000000000  , \"T\"->  1.900000000000  , \"B\"-> 12.000000000000  , \"θ\"-> 45.000000000000  , \"Reoff\"-> 0.000000000000  ,  \"Imoff\"-> 0.000000000000  |>   , \r\"IDS0323_210901_RAW_cal__ref_\" ->   <| \"ζ\"->  0.018290634783  , \"τ1\"-> 0.011707989393  , \"τS\"-> 0.007391181448  , \"τN\"-> 0.000042685582  , \"τC\"-> 0.004638632451  , \"κ0\"-> 0.000000023525  , \"mm1\"-> 0.000000000000  , \"mm2\"-> 0.000000000000  , \"mm3\"-> 0.000000000000  , \"T\"->  3.100000000000  , \"B\"-> 12.000000000000  , \"θ\"-> 45.000000000000  , \"Reoff\"-> 0.000000000000  ,  \"Imoff\"-> 0.000000000000  |>   , \r\"IDS0323_210901_RAW_cal__sam_\" ->   <| \"ζ\"->  0.019438138135  , \"τ1\"-> 0.013521019406  , \"τS\"-> 0.007253169401  , \"τN\"-> 0.000154824830  , \"τC\"-> 0.004746579385  , \"κ0\"-> 0.000000023466  , \"mm1\"-> 0.000000000000  , \"mm2\"-> 0.000000000000  , \"mm3\"-> 0.000000000000  , \"T\"->  3.100000000000  , \"B\"-> 12.000000000000  , \"θ\"-> 45.000000000000  , \"Reoff\"-> 0.000000000000  ,  \"Imoff\"-> 0.000000000000  |>   , \r\"IDS0324_210901_RAW_cal__ref_\" ->   <| \"ζ\"->  0.016342153608  , \"τ1\"-> 0.012470308436  , \"τS\"-> 0.004793459347  , \"τN\"-> 0.000012881713  , \"τC\"-> 0.003213848745  , \"κ0\"-> 0.000000058321  , \"mm1\"-> 0.000000000000  , \"mm2\"-> 0.000000000000  , \"mm3\"-> 0.000000000000  , \"T\"->  5.700000000000  , \"B\"-> 12.000000000000  , \"θ\"-> 45.000000000000  , \"Reoff\"-> 0.000000000000  ,  \"Imoff\"-> 0.000000000000  |>   , \r\"IDS0324_210901_RAW_cal__sam_\" ->   <| \"ζ\"->  0.018573189054  , \"τ1\"-> 0.013304612245  , \"τS\"-> 0.003723860844  , \"τN\"-> 0.000084829442  , \"τC\"-> 0.004309703632  , \"κ0\"-> 0.000000058362  , \"mm1\"-> 0.000000000000  , \"mm2\"-> 0.000000000000  , \"mm3\"-> 0.000000000000  , \"T\"->  5.700000000000  , \"B\"-> 12.000000000000  , \"θ\"-> 45.000000000000  , \"Reoff\"-> 0.000000000000  ,  \"Imoff\"-> 0.000000000000  |>   , \r\"IDS0330_210901_RAW_cal__ref_\" ->   <| \"ζ\"->  0.000000000000  , \"τ1\"-> 0.000000000000  , \"τS\"-> 0.000000000000  , \"τN\"-> 0.000000000000  , \"τC\"-> 0.000000000000  , \"κ0\"-> 0.000000000000  , \"mm1\"-> 0.000000000000  , \"mm2\"-> 0.000000000000  , \"mm3\"-> 0.000000000000  , \"T\"->  0.197000000000  , \"B\"-> 1.000000000000  , \"θ\"-> 90.000000000000  , \"Reoff\"-> 0.000000000000  ,  \"Imoff\"-> 0.000000000000  |>   , \r\"IDS0330_210901_RAW_cal__sam_\" ->   <| \"ζ\"->  0.000000000000  , \"τ1\"-> 0.000000000000  , \"τS\"-> 0.000000000000  , \"τN\"-> 0.000000000000  , \"τC\"-> 0.000000000000  , \"κ0\"-> 0.000000000000  , \"mm1\"-> 0.000000000000  , \"mm2\"-> 0.000000000000  , \"mm3\"-> 0.000000000000  , \"T\"->  0.197000000000  , \"B\"-> 1.000000000000  , \"θ\"-> 90.000000000000  , \"Reoff\"-> 0.000000000000  ,  \"Imoff\"-> 0.000000000000  |>   , \r\"IDS0331_210901_RAW_cal__ref_\" ->   <| \"ζ\"->  0.000000000000  , \"τ1\"-> 0.000000000000  , \"τS\"-> 0.000000000000  , \"τN\"-> 0.000000000000  , \"τC\"-> 0.000000000000  , \"κ0\"-> 0.000000000000  , \"mm1\"-> 0.000000000000  , \"mm2\"-> 0.000000000000  , \"mm3\"-> 0.000000000000  , \"T\"->  0.197000000000  , \"B\"-> 2.000000000000  , \"θ\"-> 90.000000000000  , \"Reoff\"-> 0.000000000000  ,  \"Imoff\"-> 0.000000000000  |>   , \r\"IDS0331_210901_RAW_cal__sam_\" ->   <| \"ζ\"->  0.000000000000  , \"τ1\"-> 0.000000000000  , \"τS\"-> 0.000000000000  , \"τN\"-> 0.000000000000  , \"τC\"-> 0.000000000000  , \"κ0\"-> 0.000000000000  , \"mm1\"-> 0.000000000000  , \"mm2\"-> 0.000000000000  , \"mm3\"-> 0.000000000000  , \"T\"->  0.197000000000  , \"B\"-> 2.000000000000  , \"θ\"-> 90.000000000000  , \"Reoff\"-> 0.000000000000  ,  \"Imoff\"-> 0.000000000000  |>   , \r\"IDS0335_210904_RAW_cal__ref_\" ->   <| \"ζ\"->  0.205618532862  , \"τ1\"-> 0.028612909720  , \"τS\"-> 0.084090311279  , \"τN\"-> 0.011152345581  , \"τC\"-> 0.001128858349  , \"κ0\"-> 0.000000001027  , \"mm1\"-> 0.000000000000  , \"mm2\"-> 0.000000000000  , \"mm3\"-> 0.000000000000  , \"T\"->  0.197000000000  , \"B\"-> 5.000000000000  , \"θ\"-> 90.000000000000  , \"Reoff\"-> 0.000000000000  ,  \"Imoff\"-> 0.000000000000  |>   , \r\"IDS0335_210904_RAW_cal__sam_\" ->   <| \"ζ\"->  0.126082356467  , \"τ1\"-> 0.023836839175  , \"τS\"-> 0.108299123409  , \"τN\"-> 0.016157535301  , \"τC\"-> 0.001495872883  , \"κ0\"-> 0.000000001129  , \"mm1\"-> 0.000000000000  , \"mm2\"-> 0.000000000000  , \"mm3\"-> 0.000000000000  , \"T\"->  0.197000000000  , \"B\"-> 5.000000000000  , \"θ\"-> 90.000000000000  , \"Reoff\"-> 0.000000000000  ,  \"Imoff\"-> 0.000000000000  |>   , \r\"IDS0336_210904_RAW_cal__ref_\" ->   <| \"ζ\"->  0.377660981852  , \"τ1\"-> 0.036159766180  , \"τS\"-> 0.243252714335  , \"τN\"-> 0.066015553792  , \"τC\"-> 0.001193553495  , \"κ0\"-> 0.000000000401  , \"mm1\"-> 0.000000000000  , \"mm2\"-> 0.000000000000  , \"mm3\"-> 0.000000000000  , \"T\"->  0.122000000000  , \"B\"-> 5.000000000000  , \"θ\"-> 90.000000000000  , \"Reoff\"-> 0.000000000000  ,  \"Imoff\"-> 0.000000000000  |>   , \r\"IDS0336_210904_RAW_cal__sam_\" ->   <| \"ζ\"->  0.192483765517  , \"τ1\"-> 0.026761797789  , \"τS\"-> 0.278068103221  , \"τN\"-> 0.092231648139  , \"τC\"-> 0.001612694918  , \"κ0\"-> 0.000000000500  , \"mm1\"-> 0.000000000000  , \"mm2\"-> 0.000000000000  , \"mm3\"-> 0.000000000000  , \"T\"->  0.122000000000  , \"B\"-> 5.000000000000  , \"θ\"-> 90.000000000000  , \"Reoff\"-> 0.000000000000  ,  \"Imoff\"-> 0.000000000000  |>   , \r\"IDS0337_210904_RAW_cal__ref_\" ->   <| \"ζ\"->  0.292301348133  , \"τ1\"-> 0.030611642987  , \"τS\"-> 0.124087101124  , \"τN\"-> 0.023664682612  , \"τC\"-> 0.001132116536  , \"κ0\"-> 0.000000000644  , \"mm1\"-> 0.000000000000  , \"mm2\"-> 0.000000000000  , \"mm3\"-> 0.000000000000  , \"T\"->  0.157000000000  , \"B\"-> 5.000000000000  , \"θ\"-> 90.000000000000  , \"Reoff\"-> 0.000000000000  ,  \"Imoff\"-> 0.000000000000  |>   , \r\"IDS0337_210904_RAW_cal__sam_\" ->   <| \"ζ\"->  0.176757536135  , \"τ1\"-> 0.025030443527  , \"τS\"-> 0.157985418261  , \"τN\"-> 0.029253173903  , \"τC\"-> 0.001444377194  , \"κ0\"-> 0.000000000743  , \"mm1\"-> 0.000000000000  , \"mm2\"-> 0.000000000000  , \"mm3\"-> 0.000000000000  , \"T\"->  0.157000000000  , \"B\"-> 5.000000000000  , \"θ\"-> 90.000000000000  , \"Reoff\"-> 0.000000000000  ,  \"Imoff\"-> 0.000000000000  |>   , \r\"IDS0338_210904_RAW_cal__ref_\" ->   <| \"ζ\"->  0.269368133659  , \"τ1\"-> 0.031385344058  , \"τS\"-> 0.109862526856  , \"τN\"-> 0.015552760916  , \"τC\"-> 0.001072566411  , \"κ0\"-> 0.000000000733  , \"mm1\"-> 0.000000000000  , \"mm2\"-> 0.000000000000  , \"mm3\"-> 0.000000000000  , \"T\"->  0.170000000000  , \"B\"-> 5.000000000000  , \"θ\"-> 90.000000000000  , \"Reoff\"-> 0.000000000000  ,  \"Imoff\"-> 0.000000000000  |>   , \r\"IDS0338_210904_RAW_cal__sam_\" ->   <| \"ζ\"->  0.157490327814  , \"τ1\"-> 0.025072576319  , \"τS\"-> 0.138913916780  , \"τN\"-> 0.024096402149  , \"τC\"-> 0.001407824448  , \"κ0\"-> 0.000000000841  , \"mm1\"-> 0.000000000000  , \"mm2\"-> 0.000000000000  , \"mm3\"-> 0.000000000000  , \"T\"->  0.170000000000  , \"B\"-> 5.000000000000  , \"θ\"-> 90.000000000000  , \"Reoff\"-> 0.000000000000  ,  \"Imoff\"-> 0.000000000000  |>   , \r\"IDS0339_210904_RAW_cal__ref_\" ->   <| \"ζ\"->  0.119576376746  , \"τ1\"-> 0.024981853669  , \"τS\"-> 0.059873041409  , \"τN\"-> 0.005204458221  , \"τC\"-> 0.001289686309  , \"κ0\"-> 0.000000001340  , \"mm1\"-> 0.000000000000  , \"mm2\"-> 0.000000000000  , \"mm3\"-> 0.000000000000  , \"T\"->  0.255000000000  , \"B\"-> 5.000000000000  , \"θ\"-> 90.000000000000  , \"Reoff\"-> 0.000000000000  ,  \"Imoff\"-> 0.000000000000  |>   , \r\"IDS0339_210904_RAW_cal__sam_\" ->   <| \"ζ\"->  0.071547151941  , \"τ1\"-> 0.023411099214  , \"τS\"-> 0.077624659702  , \"τN\"-> 0.006792929714  , \"τC\"-> 0.001758131380  , \"κ0\"-> 0.000000001477  , \"mm1\"-> 0.000000000000  , \"mm2\"-> 0.000000000000  , \"mm3\"-> 0.000000000000  , \"T\"->  0.255000000000  , \"B\"-> 5.000000000000  , \"θ\"-> 90.000000000000  , \"Reoff\"-> 0.000000000000  ,  \"Imoff\"-> 0.000000000000  |>   , \r\"IDS0340_210904_RAW_cal__ref_\" ->   <| \"ζ\"->  0.082683893253  , \"τ1\"-> 0.024702194699  , \"τS\"-> 0.049753720072  , \"τN\"-> 0.002517387539  , \"τC\"-> 0.001542602546  , \"κ0\"-> 0.000000001719  , \"mm1\"-> 0.000000000000  , \"mm2\"-> 0.000000000000  , \"mm3\"-> 0.000000000000  , \"T\"->  0.308000000000  , \"B\"-> 5.000000000000  , \"θ\"-> 90.000000000000  , \"Reoff\"-> 0.000000000000  ,  \"Imoff\"-> 0.000000000000  |>   , \r\"IDS0340_210904_RAW_cal__sam_\" ->   <| \"ζ\"->  0.049129914970  , \"τ1\"-> 0.024898573189  , \"τS\"-> 0.064441011576  , \"τN\"-> 0.003850324949  , \"τC\"-> 0.002205260995  , \"κ0\"-> 0.000000001876  , \"mm1\"-> 0.000000000000  , \"mm2\"-> 0.000000000000  , \"mm3\"-> 0.000000000000  , \"T\"->  0.308000000000  , \"B\"-> 5.000000000000  , \"θ\"-> 90.000000000000  , \"Reoff\"-> 0.000000000000  ,  \"Imoff\"-> 0.000000000000  |>   , \r\"IDS0341_210904_RAW_cal__ref_\" ->   <| \"ζ\"->  0.059616809183  , \"τ1\"-> 0.023939570797  , \"τS\"-> 0.042653632086  , \"τN\"-> 0.001786288241  , \"τC\"-> 0.001975926031  , \"κ0\"-> 0.000000002092  , \"mm1\"-> 0.000000000000  , \"mm2\"-> 0.000000000000  , \"mm3\"-> 0.000000000000  , \"T\"->  0.360000000000  , \"B\"-> 5.000000000000  , \"θ\"-> 90.000000000000  , \"Reoff\"-> 0.000000000000  ,  \"Imoff\"-> 0.000000000000  |>   , \r\"IDS0341_210904_RAW_cal__sam_\" ->   <| \"ζ\"->  0.036232012390  , \"τ1\"-> 0.027781521532  , \"τS\"-> 0.055391702939  , \"τN\"-> 0.001971026378  , \"τC\"-> 0.002721128929  , \"κ0\"-> 0.000000002279  , \"mm1\"-> 0.000000000000  , \"mm2\"-> 0.000000000000  , \"mm3\"-> 0.000000000000  , \"T\"->  0.360000000000  , \"B\"-> 5.000000000000  , \"θ\"-> 90.000000000000  , \"Reoff\"-> 0.000000000000  ,  \"Imoff\"-> 0.000000000000  |>   , \r\"IDS0342_210904_RAW_cal__ref_\" ->   <| \"ζ\"->  0.044217232361  , \"τ1\"-> 0.023574215500  , \"τS\"-> 0.035981580515  , \"τN\"-> 0.001074333911  , \"τC\"-> 0.002351862552  , \"κ0\"-> 0.000000002629  , \"mm1\"-> 0.000000000000  , \"mm2\"-> 0.000000000000  , \"mm3\"-> 0.000000000000  , \"T\"->  0.438000000000  , \"B\"-> 5.000000000000  , \"θ\"-> 90.000000000000  , \"Reoff\"-> 0.000000000000  ,  \"Imoff\"-> 0.000000000000  |>   , \r\"IDS0342_210904_RAW_cal__sam_\" ->   <| \"ζ\"->  0.029055572135  , \"τ1\"-> 0.027337777983  , \"τS\"-> 0.046740216600  , \"τN\"-> 0.000913387218  , \"τC\"-> 0.003013145103  , \"κ0\"-> 0.000000002847  , \"mm1\"-> 0.000000000000  , \"mm2\"-> 0.000000000000  , \"mm3\"-> 0.000000000000  , \"T\"->  0.438000000000  , \"B\"-> 5.000000000000  , \"θ\"-> 90.000000000000  , \"Reoff\"-> 0.000000000000  ,  \"Imoff\"-> 0.000000000000  |>   , \r\"IDS0343_210904_RAW_cal__ref_\" ->   <| \"ζ\"->  0.035878652194  , \"τ1\"-> 0.022884594376  , \"τS\"-> 0.030627660510  , \"τN\"-> 0.000467937158  , \"τC\"-> 0.002753754811  , \"κ0\"-> 0.000000003272  , \"mm1\"-> 0.000000000000  , \"mm2\"-> 0.000000000000  , \"mm3\"-> 0.000000000000  , \"T\"->  0.530000000000  , \"B\"-> 5.000000000000  , \"θ\"-> 90.000000000000  , \"Reoff\"-> 0.000000000000  ,  \"Imoff\"-> 0.000000000000  |>   , \r\"IDS0343_210904_RAW_cal__sam_\" ->   <| \"ζ\"->  0.023052185319  , \"τ1\"-> 0.024218669224  , \"τS\"-> 0.038947570428  , \"τN\"-> 0.000553100922  , \"τC\"-> 0.003936712296  , \"κ0\"-> 0.000000003540  , \"mm1\"-> 0.000000000000  , \"mm2\"-> 0.000000000000  , \"mm3\"-> 0.000000000000  , \"T\"->  0.530000000000  , \"B\"-> 5.000000000000  , \"θ\"-> 90.000000000000  , \"Reoff\"-> 0.000000000000  ,  \"Imoff\"-> 0.000000000000  |>   , \r\"IDS0344_210904_RAW_cal__ref_\" ->   <| \"ζ\"->  0.028793115659  , \"τ1\"-> 0.021896518366  , \"τS\"-> 0.026819338540  , \"τN\"-> 0.000265027076  , \"τC\"-> 0.003129703951  , \"κ0\"-> 0.000000003891  , \"mm1\"-> 0.000000000000  , \"mm2\"-> 0.000000000000  , \"mm3\"-> 0.000000000000  , \"T\"->  0.620000000000  , \"B\"-> 5.000000000000  , \"θ\"-> 90.000000000000  , \"Reoff\"-> 0.000000000000  ,  \"Imoff\"-> 0.000000000000  |>   , \r\"IDS0344_210904_RAW_cal__sam_\" ->   <| \"ζ\"->  0.019128182776  , \"τ1\"-> 0.023636717673  , \"τS\"-> 0.033826494614  , \"τN\"-> 0.000313261552  , \"τC\"-> 0.004366795222  , \"κ0\"-> 0.000000004225  , \"mm1\"-> 0.000000000000  , \"mm2\"-> 0.000000000000  , \"mm3\"-> 0.000000000000  , \"T\"->  0.620000000000  , \"B\"-> 5.000000000000  , \"θ\"-> 90.000000000000  , \"Reoff\"-> 0.000000000000  ,  \"Imoff\"-> 0.000000000000  |>   , \r\"IDS0346_210904_RAW_cal__ref_\" ->   <| \"ζ\"->  0.351410523880  , \"τ1\"-> 0.038660935015  , \"τS\"-> 0.057750106762  , \"τN\"-> 0.192483765517  , \"τC\"-> 0.000883347451  , \"κ0\"-> 0.000000000403  , \"mm1\"-> 0.000000000000  , \"mm2\"-> 0.000000000000  , \"mm3\"-> 0.000000000000  , \"T\"->  0.122000000000  , \"B\"-> 8.000000000000  , \"θ\"-> 90.000000000000  , \"Reoff\"-> 0.000000000000  ,  \"Imoff\"-> 0.000000000000  |>   , \r\"IDS0346_210904_RAW_cal__sam_\" ->   <| \"ζ\"->  0.000000000000  , \"τ1\"-> 0.000000000000  , \"τS\"-> 0.000000000000  , \"τN\"-> 0.000000000000  , \"τC\"-> 0.000000000000  , \"κ0\"-> 0.000000000000  , \"mm1\"-> 0.000000000000  , \"mm2\"-> 0.000000000000  , \"mm3\"-> 0.000000000000  , \"T\"->  0.122000000000  , \"B\"-> 8.000000000000  , \"θ\"-> 90.000000000000  , \"Reoff\"-> 0.000000000000  ,  \"Imoff\"-> 0.000000000000  |>   , \r\"IDS0347_210906_RAW_cal__ref_\" ->   <| \"ζ\"->  0.282365663511  , \"τ1\"-> 0.039144945999  , \"τS\"-> 0.059953399264  , \"τN\"-> 0.108048405778  , \"τC\"-> 0.001096068963  , \"κ0\"-> 0.000000000641  , \"mm1\"-> 0.000000000000  , \"mm2\"-> 0.000000000000  , \"mm3\"-> 0.000000000000  , \"T\"->  0.157000000000  , \"B\"-> 8.000000000000  , \"θ\"-> 90.000000000000  , \"Reoff\"-> 0.000000000000  ,  \"Imoff\"-> 0.000000000000  |>   , \r\"IDS0347_210906_RAW_cal__sam_\" ->   <| \"ζ\"->  0.000000000000  , \"τ1\"-> 0.000000000000  , \"τS\"-> 0.000000000000  , \"τN\"-> 0.000000000000  , \"τC\"-> 0.000000000000  , \"κ0\"-> 0.000000000000  , \"mm1\"-> 0.000000000000  , \"mm2\"-> 0.000000000000  , \"mm3\"-> 0.000000000000  , \"T\"->  0.157000000000  , \"B\"-> 8.000000000000  , \"θ\"-> 90.000000000000  , \"Reoff\"-> 0.000000000000  ,  \"Imoff\"-> 0.000000000000  |>   , \r\"IDS0348_210906_RAW_cal__ref_\" ->   <| \"ζ\"->  0.231232733983  , \"τ1\"-> 0.036430431380  , \"τS\"-> 0.054781597050  , \"τN\"-> 0.064844477869  , \"τC\"-> 0.001068830966  , \"κ0\"-> 0.000000000760  , \"mm1\"-> 0.000000000000  , \"mm2\"-> 0.000000000000  , \"mm3\"-> 0.000000000000  , \"T\"->  0.178000000000  , \"B\"-> 8.000000000000  , \"θ\"-> 90.000000000000  , \"Reoff\"-> 0.000000000000  ,  \"Imoff\"-> 0.000000000000  |>   , \r\"IDS0348_210906_RAW_cal__sam_\" ->   <| \"ζ\"->  0.000000000000  , \"τ1\"-> 0.000000000000  , \"τS\"-> 0.000000000000  , \"τN\"-> 0.000000000000  , \"τC\"-> 0.000000000000  , \"κ0\"-> 0.000000000000  , \"mm1\"-> 0.000000000000  , \"mm2\"-> 0.000000000000  , \"mm3\"-> 0.000000000000  , \"T\"->  0.178000000000  , \"B\"-> 8.000000000000  , \"θ\"-> 90.000000000000  , \"Reoff\"-> 0.000000000000  ,  \"Imoff\"-> 0.000000000000  |>   , \r\"IDS0349_210906_RAW_cal__ref_\" ->   <| \"ζ\"->  0.190485473901  , \"τ1\"-> 0.032323616024  , \"τS\"-> 0.052823523941  , \"τN\"-> 0.036537332757  , \"τC\"-> 0.001181014846  , \"κ0\"-> 0.000000001037  , \"mm1\"-> 0.000000000000  , \"mm2\"-> 0.000000000000  , \"mm3\"-> 0.000000000000  , \"T\"->  0.200000000000  , \"B\"-> 8.000000000000  , \"θ\"-> 90.000000000000  , \"Reoff\"-> 0.000000000000  ,  \"Imoff\"-> 0.000000000000  |>   , \r\"IDS0349_210906_RAW_cal__sam_\" ->   <| \"ζ\"->  0.000000000000  , \"τ1\"-> 0.000000000000  , \"τS\"-> 0.000000000000  , \"τN\"-> 0.000000000000  , \"τC\"-> 0.000000000000  , \"κ0\"-> 0.000000000000  , \"mm1\"-> 0.000000000000  , \"mm2\"-> 0.000000000000  , \"mm3\"-> 0.000000000000  , \"T\"->  0.200000000000  , \"B\"-> 8.000000000000  , \"θ\"-> 90.000000000000  , \"Reoff\"-> 0.000000000000  ,  \"Imoff\"-> 0.000000000000  |>   , \r\"IDS0350_210906_RAW_cal__ref_\" ->   <| \"ζ\"->  0.118733755426  , \"τ1\"-> 0.027090622935  , \"τS\"-> 0.042154952610  , \"τN\"-> 0.016299612233  , \"τC\"-> 0.001268322773  , \"κ0\"-> 0.000000001347  , \"mm1\"-> 0.000000000000  , \"mm2\"-> 0.000000000000  , \"mm3\"-> 0.000000000000  , \"T\"->  0.260000000000  , \"B\"-> 8.000000000000  , \"θ\"-> 90.000000000000  , \"Reoff\"-> 0.000000000000  ,  \"Imoff\"-> 0.000000000000  |>   , \r\"IDS0350_210906_RAW_cal__sam_\" ->   <| \"ζ\"->  0.000000000000  , \"τ1\"-> 0.000000000000  , \"τS\"-> 0.000000000000  , \"τN\"-> 0.000000000000  , \"τC\"-> 0.000000000000  , \"κ0\"-> 0.000000000000  , \"mm1\"-> 0.000000000000  , \"mm2\"-> 0.000000000000  , \"mm3\"-> 0.000000000000  , \"T\"->  0.260000000000  , \"B\"-> 8.000000000000  , \"θ\"-> 90.000000000000  , \"Reoff\"-> 0.000000000000  ,  \"Imoff\"-> 0.000000000000  |>   , \r\"IDS0351_210906_RAW_cal__ref_\" ->   <| \"ζ\"->  0.081031099964  , \"τ1\"-> 0.021876847581  , \"τS\"-> 0.037173038366  , \"τN\"-> 0.007845971856  , \"τC\"-> 0.001561862252  , \"κ0\"-> 0.000000001761  , \"mm1\"-> 0.000000000000  , \"mm2\"-> 0.000000000000  , \"mm3\"-> 0.000000000000  , \"T\"->  0.310000000000  , \"B\"-> 8.000000000000  , \"θ\"-> 90.000000000000  , \"Reoff\"-> 0.000000000000  ,  \"Imoff\"-> 0.000000000000  |>   , \r\"IDS0351_210906_RAW_cal__sam_\" ->   <| \"ζ\"->  0.000000000000  , \"τ1\"-> 0.000000000000  , \"τS\"-> 0.000000000000  , \"τN\"-> 0.000000000000  , \"τC\"-> 0.000000000000  , \"κ0\"-> 0.000000000000  , \"mm1\"-> 0.000000000000  , \"mm2\"-> 0.000000000000  , \"mm3\"-> 0.000000000000  , \"T\"->  0.310000000000  , \"B\"-> 8.000000000000  , \"θ\"-> 90.000000000000  , \"Reoff\"-> 0.000000000000  ,  \"Imoff\"-> 0.000000000000  |>   , \r\"IDS0352_210906_RAW_cal__ref_\" ->   <| \"ζ\"->  0.060336863550  , \"τ1\"-> 0.020607625563  , \"τS\"-> 0.034334079822  , \"τN\"-> 0.004923011954  , \"τC\"-> 0.001895452704  , \"κ0\"-> 0.000000002106  , \"mm1\"-> 0.000000000000  , \"mm2\"-> 0.000000000000  , \"mm3\"-> 0.000000000000  , \"T\"->  0.360000000000  , \"B\"-> 8.000000000000  , \"θ\"-> 90.000000000000  , \"Reoff\"-> 0.000000000000  ,  \"Imoff\"-> 0.000000000000  |>   , \r\"IDS0352_210906_RAW_cal__sam_\" ->   <| \"ζ\"->  0.000000000000  , \"τ1\"-> 0.000000000000  , \"τS\"-> 0.000000000000  , \"τN\"-> 0.000000000000  , \"τC\"-> 0.000000000000  , \"κ0\"-> 0.000000000000  , \"mm1\"-> 0.000000000000  , \"mm2\"-> 0.000000000000  , \"mm3\"-> 0.000000000000  , \"T\"->  0.360000000000  , \"B\"-> 8.000000000000  , \"θ\"-> 90.000000000000  , \"Reoff\"-> 0.000000000000  ,  \"Imoff\"-> 0.000000000000  |>   , \r\"IDS0353_210906_RAW_cal__ref_\" ->   <| \"ζ\"->  0.045012118583  , \"τ1\"-> 0.020623291685  , \"τS\"-> 0.031197986163  , \"τN\"-> 0.002724775132  , \"τC\"-> 0.002225741907  , \"κ0\"-> 0.000000002626  , \"mm1\"-> 0.000000000000  , \"mm2\"-> 0.000000000000  , \"mm3\"-> 0.000000000000  , \"T\"->  0.438000000000  , \"B\"-> 8.000000000000  , \"θ\"-> 90.000000000000  , \"Reoff\"-> 0.000000000000  ,  \"Imoff\"-> 0.000000000000  |>   , \r\"IDS0353_210906_RAW_cal__sam_\" ->   <| \"ζ\"->  0.000000000000  , \"τ1\"-> 0.000000000000  , \"τS\"-> 0.000000000000  , \"τN\"-> 0.000000000000  , \"τC\"-> 0.000000000000  , \"κ0\"-> 0.000000000000  , \"mm1\"-> 0.000000000000  , \"mm2\"-> 0.000000000000  , \"mm3\"-> 0.000000000000  , \"T\"->  0.438000000000  , \"B\"-> 8.000000000000  , \"θ\"-> 90.000000000000  , \"Reoff\"-> 0.000000000000  ,  \"Imoff\"-> 0.000000000000  |>   , \r\"IDS0354_210906_RAW_cal__ref_\" ->   <| \"ζ\"->  0.035878229865  , \"τ1\"-> 0.020618191238  , \"τS\"-> 0.028341492437  , \"τN\"-> 0.001542437572  , \"τC\"-> 0.002465046672  , \"κ0\"-> 0.000000003272  , \"mm1\"-> 0.000000000000  , \"mm2\"-> 0.000000000000  , \"mm3\"-> 0.000000000000  , \"T\"->  0.530000000000  , \"B\"-> 8.000000000000  , \"θ\"-> 90.000000000000  , \"Reoff\"-> 0.000000000000  ,  \"Imoff\"-> 0.000000000000  |>   , \r\"IDS0354_210906_RAW_cal__sam_\" ->   <| \"ζ\"->  0.000000000000  , \"τ1\"-> 0.000000000000  , \"τS\"-> 0.000000000000  , \"τN\"-> 0.000000000000  , \"τC\"-> 0.000000000000  , \"κ0\"-> 0.000000000000  , \"mm1\"-> 0.000000000000  , \"mm2\"-> 0.000000000000  , \"mm3\"-> 0.000000000000  , \"T\"->  0.530000000000  , \"B\"-> 8.000000000000  , \"θ\"-> 90.000000000000  , \"Reoff\"-> 0.000000000000  ,  \"Imoff\"-> 0.000000000000  |>   , \r\"IDS0355_210906_RAW_cal__ref_\" ->   <| \"ζ\"->  0.022259133140  , \"τ1\"-> 0.021062021806  , \"τS\"-> 0.021361272182  , \"τN\"-> 0.000526217477  , \"τC\"-> 0.003770290408  , \"κ0\"-> 0.000000005411  , \"mm1\"-> 0.000000000000  , \"mm2\"-> 0.000000000000  , \"mm3\"-> 0.000000000000  , \"T\"->  0.830000000000  , \"B\"-> 8.000000000000  , \"θ\"-> 90.000000000000  , \"Reoff\"-> 0.000000000000  ,  \"Imoff\"-> 0.000000000000  |>   , \r\"IDS0355_210906_RAW_cal__sam_\" ->   <| \"ζ\"->  0.000000000000  , \"τ1\"-> 0.000000000000  , \"τS\"-> 0.000000000000  , \"τN\"-> 0.000000000000  , \"τC\"-> 0.000000000000  , \"κ0\"-> 0.000000000000  , \"mm1\"-> 0.000000000000  , \"mm2\"-> 0.000000000000  , \"mm3\"-> 0.000000000000  , \"T\"->  0.830000000000  , \"B\"-> 8.000000000000  , \"θ\"-> 90.000000000000  , \"Reoff\"-> 0.000000000000  ,  \"Imoff\"-> 0.000000000000  |>   , \r\"IDS0359_210907_RAW_cal__ref_\" ->   <| \"ζ\"->  0.381003010305  , \"τ1\"-> 0.083336505244  , \"τS\"-> 0.050211621127  , \"τN\"-> 0.550745531665  , \"τC\"-> 0.000692694606  , \"κ0\"-> 0.000000000382  , \"mm1\"-> 0.000000000000  , \"mm2\"-> 0.000000000000  , \"mm3\"-> 0.000000000000  , \"T\"->  0.120000000000  , \"B\"-> 12.000000000000  , \"θ\"-> 60.000000000000  , \"Reoff\"-> 0.000000000000  ,  \"Imoff\"-> 0.000000000000  |>   , \r\"IDS0359_210907_RAW_cal__sam_\" ->   <| \"ζ\"->  0.000000000000  , \"τ1\"-> 0.000000000000  , \"τS\"-> 0.000000000000  , \"τN\"-> 0.000000000000  , \"τC\"-> 0.000000000000  , \"κ0\"-> 0.000000000000  , \"mm1\"-> 0.000000000000  , \"mm2\"-> 0.000000000000  , \"mm3\"-> 0.000000000000  , \"T\"->  0.120000000000  , \"B\"-> 12.000000000000  , \"θ\"-> 60.000000000000  , \"Reoff\"-> 0.000000000000  ,  \"Imoff\"-> 0.000000000000  |>   , \r\"IDS0360_210907_RAW_cal__ref_\" ->   <| \"ζ\"->  0.323840637004  , \"τ1\"-> 0.072581646931  , \"τS\"-> 0.047951414335  , \"τN\"-> 0.283785405218  , \"τC\"-> 0.000913184933  , \"κ0\"-> 0.000000000636  , \"mm1\"-> 0.000000000000  , \"mm2\"-> 0.000000000000  , \"mm3\"-> 0.000000000000  , \"T\"->  0.150000000000  , \"B\"-> 12.000000000000  , \"θ\"-> 60.000000000000  , \"Reoff\"-> 0.000000000000  ,  \"Imoff\"-> 0.000000000000  |>   , \r\"IDS0360_210907_RAW_cal__sam_\" ->   <| \"ζ\"->  0.000000000000  , \"τ1\"-> 0.000000000000  , \"τS\"-> 0.000000000000  , \"τN\"-> 0.000000000000  , \"τC\"-> 0.000000000000  , \"κ0\"-> 0.000000000000  , \"mm1\"-> 0.000000000000  , \"mm2\"-> 0.000000000000  , \"mm3\"-> 0.000000000000  , \"T\"->  0.150000000000  , \"B\"-> 12.000000000000  , \"θ\"-> 60.000000000000  , \"Reoff\"-> 0.000000000000  ,  \"Imoff\"-> 0.000000000000  |>   , \r\"IDS0361_210908_RAW_cal__ref_\" ->   <| \"ζ\"->  0.279940228007  , \"τ1\"-> 0.067057240536  , \"τS\"-> 0.048025817643  , \"τN\"-> 0.170011495172  , \"τC\"-> 0.001015047914  , \"κ0\"-> 0.000000000754  , \"mm1\"-> 0.000000000000  , \"mm2\"-> 0.000000000000  , \"mm3\"-> 0.000000000000  , \"T\"->  0.168000000000  , \"B\"-> 12.000000000000  , \"θ\"-> 60.000000000000  , \"Reoff\"-> 0.000000000000  ,  \"Imoff\"-> 0.000000000000  |>   , \r\"IDS0361_210908_RAW_cal__sam_\" ->   <| \"ζ\"->  0.000000000000  , \"τ1\"-> 0.000000000000  , \"τS\"-> 0.000000000000  , \"τN\"-> 0.000000000000  , \"τC\"-> 0.000000000000  , \"κ0\"-> 0.000000000000  , \"mm1\"-> 0.000000000000  , \"mm2\"-> 0.000000000000  , \"mm3\"-> 0.000000000000  , \"T\"->  0.168000000000  , \"B\"-> 12.000000000000  , \"θ\"-> 60.000000000000  , \"Reoff\"-> 0.000000000000  ,  \"Imoff\"-> 0.000000000000  |>   , \r\"IDS0362_210908_RAW_cal__ref_\" ->   <| \"ζ\"->  0.206594976212  , \"τ1\"-> 0.057885925979  , \"τS\"-> 0.038698575169  , \"τN\"-> 0.092347634602  , \"τC\"-> 0.001108131545  , \"κ0\"-> 0.000000001046  , \"mm1\"-> 0.000000000000  , \"mm2\"-> 0.000000000000  , \"mm3\"-> 0.000000000000  , \"T\"->  0.197000000000  , \"B\"-> 12.000000000000  , \"θ\"-> 60.000000000000  , \"Reoff\"-> 0.000000000000  ,  \"Imoff\"-> 0.000000000000  |>   , \r\"IDS0362_210908_RAW_cal__sam_\" ->   <| \"ζ\"->  0.000000000000  , \"τ1\"-> 0.000000000000  , \"τS\"-> 0.000000000000  , \"τN\"-> 0.000000000000  , \"τC\"-> 0.000000000000  , \"κ0\"-> 0.000000000000  , \"mm1\"-> 0.000000000000  , \"mm2\"-> 0.000000000000  , \"mm3\"-> 0.000000000000  , \"T\"->  0.197000000000  , \"B\"-> 12.000000000000  , \"θ\"-> 60.000000000000  , \"Reoff\"-> 0.000000000000  ,  \"Imoff\"-> 0.000000000000  |>   , \r\"IDS0363_210908_RAW_cal__ref_\" ->   <| \"ζ\"->  0.123216898961  , \"τ1\"-> 0.041424716624  , \"τS\"-> 0.030606562009  , \"τN\"-> 0.033679175657  , \"τC\"-> 0.001245281919  , \"κ0\"-> 0.000000001353  , \"mm1\"-> 0.000000000000  , \"mm2\"-> 0.000000000000  , \"mm3\"-> 0.000000000000  , \"T\"->  0.250000000000  , \"B\"-> 12.000000000000  , \"θ\"-> 60.000000000000  , \"Reoff\"-> 0.000000000000  ,  \"Imoff\"-> 0.000000000000  |>   , \r\"IDS0363_210908_RAW_cal__sam_\" ->   <| \"ζ\"->  0.000000000000  , \"τ1\"-> 0.000000000000  , \"τS\"-> 0.000000000000  , \"τN\"-> 0.000000000000  , \"τC\"-> 0.000000000000  , \"κ0\"-> 0.000000000000  , \"mm1\"-> 0.000000000000  , \"mm2\"-> 0.000000000000  , \"mm3\"-> 0.000000000000  , \"T\"->  0.250000000000  , \"B\"-> 12.000000000000  , \"θ\"-> 60.000000000000  , \"Reoff\"-> 0.000000000000  ,  \"Imoff\"-> 0.000000000000  |>   , \r\"IDS0364_210908_RAW_cal__ref_\" ->   <| \"ζ\"->  0.083979493288  , \"τ1\"-> 0.035863468022  , \"τS\"-> 0.027413945050  , \"τN\"-> 0.017174500536  , \"τC\"-> 0.001551957186  , \"κ0\"-> 0.000000001738  , \"mm1\"-> 0.000000000000  , \"mm2\"-> 0.000000000000  , \"mm3\"-> 0.000000000000  , \"T\"->  0.307000000000  , \"B\"-> 12.000000000000  , \"θ\"-> 60.000000000000  , \"Reoff\"-> 0.000000000000  ,  \"Imoff\"-> 0.000000000000  |>   , \r\"IDS0364_210908_RAW_cal__sam_\" ->   <| \"ζ\"->  0.000000000000  , \"τ1\"-> 0.000000000000  , \"τS\"-> 0.000000000000  , \"τN\"-> 0.000000000000  , \"τC\"-> 0.000000000000  , \"κ0\"-> 0.000000000000  , \"mm1\"-> 0.000000000000  , \"mm2\"-> 0.000000000000  , \"mm3\"-> 0.000000000000  , \"T\"->  0.307000000000  , \"B\"-> 12.000000000000  , \"θ\"-> 60.000000000000  , \"Reoff\"-> 0.000000000000  ,  \"Imoff\"-> 0.000000000000  |>   , \r\"IDS0365_210908_RAW_cal__ref_\" ->   <| \"ζ\"->  0.061526991224  , \"τ1\"-> 0.029624261727  , \"τS\"-> 0.025208021627  , \"τN\"-> 0.009698502183  , \"τC\"-> 0.001918212332  , \"κ0\"-> 0.000000002116  , \"mm1\"-> 0.000000000000  , \"mm2\"-> 0.000000000000  , \"mm3\"-> 0.000000000000  , \"T\"->  0.360000000000  , \"B\"-> 12.000000000000  , \"θ\"-> 60.000000000000  , \"Reoff\"-> 0.000000000000  ,  \"Imoff\"-> 0.000000000000  |>   , \r\"IDS0365_210908_RAW_cal__sam_\" ->   <| \"ζ\"->  0.000000000000  , \"τ1\"-> 0.000000000000  , \"τS\"-> 0.000000000000  , \"τN\"-> 0.000000000000  , \"τC\"-> 0.000000000000  , \"κ0\"-> 0.000000000000  , \"mm1\"-> 0.000000000000  , \"mm2\"-> 0.000000000000  , \"mm3\"-> 0.000000000000  , \"T\"->  0.360000000000  , \"B\"-> 12.000000000000  , \"θ\"-> 60.000000000000  , \"Reoff\"-> 0.000000000000  ,  \"Imoff\"-> 0.000000000000  |>   , \r\"IDS0366_210908_RAW_cal__ref_\" ->   <| \"ζ\"->  0.045515267447  , \"τ1\"-> 0.026001810196  , \"τS\"-> 0.023136668780  , \"τN\"-> 0.005224117981  , \"τC\"-> 0.002327400857  , \"κ0\"-> 0.000000002646  , \"mm1\"-> 0.000000000000  , \"mm2\"-> 0.000000000000  , \"mm3\"-> 0.000000000000  , \"T\"->  0.430000000000  , \"B\"-> 12.000000000000  , \"θ\"-> 60.000000000000  , \"Reoff\"-> 0.000000000000  ,  \"Imoff\"-> 0.000000000000  |>   , \r\"IDS0366_210908_RAW_cal__sam_\" ->   <| \"ζ\"->  0.000000000000  , \"τ1\"-> 0.000000000000  , \"τS\"-> 0.000000000000  , \"τN\"-> 0.000000000000  , \"τC\"-> 0.000000000000  , \"κ0\"-> 0.000000000000  , \"mm1\"-> 0.000000000000  , \"mm2\"-> 0.000000000000  , \"mm3\"-> 0.000000000000  , \"T\"->  0.430000000000  , \"B\"-> 12.000000000000  , \"θ\"-> 60.000000000000  , \"Reoff\"-> 0.000000000000  ,  \"Imoff\"-> 0.000000000000  |>   , \r\"IDS0367_210908_RAW_cal__ref_\" ->   <| \"ζ\"->  0.037324451442  , \"τ1\"-> 0.019605264024  , \"τS\"-> 0.021700560504  , \"τN\"-> 0.002800944156  , \"τC\"-> 0.002526998509  , \"κ0\"-> 0.000000003301  , \"mm1\"-> 0.000000000000  , \"mm2\"-> 0.000000000000  , \"mm3\"-> 0.000000000000  , \"T\"->  0.530000000000  , \"B\"-> 12.000000000000  , \"θ\"-> 60.000000000000  , \"Reoff\"-> 0.000000000000  ,  \"Imoff\"-> 0.000000000000  |>   , \r\"IDS0367_210908_RAW_cal__sam_\" ->   <| \"ζ\"->  0.000000000000  , \"τ1\"-> 0.000000000000  , \"τS\"-> 0.000000000000  , \"τN\"-> 0.000000000000  , \"τC\"-> 0.000000000000  , \"κ0\"-> 0.000000000000  , \"mm1\"-> 0.000000000000  , \"mm2\"-> 0.000000000000  , \"mm3\"-> 0.000000000000  , \"T\"->  0.530000000000  , \"B\"-> 12.000000000000  , \"θ\"-> 60.000000000000  , \"Reoff\"-> 0.000000000000  ,  \"Imoff\"-> 0.000000000000  |>   , \r\"IDS0368_210908_RAW_cal__ref_\" ->   <| \"ζ\"->  0.030581023885  , \"τ1\"-> 0.017326525290  , \"τS\"-> 0.020225378130  , \"τN\"-> 0.001703135365  , \"τC\"-> 0.003380889395  , \"κ0\"-> 0.000000003914  , \"mm1\"-> 0.000000000000  , \"mm2\"-> 0.000000000000  , \"mm3\"-> 0.000000000000  , \"T\"->  0.630000000000  , \"B\"-> 12.000000000000  , \"θ\"-> 60.000000000000  , \"Reoff\"-> 0.000000000000  ,  \"Imoff\"-> 0.000000000000  |>   , \r\"IDS0368_210908_RAW_cal__sam_\" ->   <| \"ζ\"->  0.000000000000  , \"τ1\"-> 0.000000000000  , \"τS\"-> 0.000000000000  , \"τN\"-> 0.000000000000  , \"τC\"-> 0.000000000000  , \"κ0\"-> 0.000000000000  , \"mm1\"-> 0.000000000000  , \"mm2\"-> 0.000000000000  , \"mm3\"-> 0.000000000000  , \"T\"->  0.630000000000  , \"B\"-> 12.000000000000  , \"θ\"-> 60.000000000000  , \"Reoff\"-> 0.000000000000  ,  \"Imoff\"-> 0.000000000000  |>   , \r\"IDS0369_210908_RAW_cal__ref_\" ->   <| \"ζ\"->  0.022212344829  , \"τ1\"-> 0.017343641344  , \"τS\"-> 0.018001662092  , \"τN\"-> 0.000711569404  , \"τC\"-> 0.004309595418  , \"κ0\"-> 0.000000005439  , \"mm1\"-> 0.000000000000  , \"mm2\"-> 0.000000000000  , \"mm3\"-> 0.000000000000  , \"T\"->  0.830000000000  , \"B\"-> 12.000000000000  , \"θ\"-> 60.000000000000  , \"Reoff\"-> 0.000000000000  ,  \"Imoff\"-> 0.000000000000  |>   , \r\"IDS0369_210908_RAW_cal__sam_\" ->   <| \"ζ\"->  0.000000000000  , \"τ1\"-> 0.000000000000  , \"τS\"-> 0.000000000000  , \"τN\"-> 0.000000000000  , \"τC\"-> 0.000000000000  , \"κ0\"-> 0.000000000000  , \"mm1\"-> 0.000000000000  , \"mm2\"-> 0.000000000000  , \"mm3\"-> 0.000000000000  , \"T\"->  0.830000000000  , \"B\"-> 12.000000000000  , \"θ\"-> 60.000000000000  , \"Reoff\"-> 0.000000000000  ,  \"Imoff\"-> 0.000000000000  |>   , \r\"IDS0370_210908_RAW_cal__ref_\" ->   <| \"ζ\"->  0.021569402950  , \"τ1\"-> 0.017921737944  , \"τS\"-> 0.015463128015  , \"τN\"-> 0.000390873619  , \"τC\"-> 0.004954240411  , \"κ0\"-> 0.000000007586  , \"mm1\"-> 0.000000000000  , \"mm2\"-> 0.000000000000  , \"mm3\"-> 0.000000000000  , \"T\"->  1.130000000000  , \"B\"-> 12.000000000000  , \"θ\"-> 60.000000000000  , \"Reoff\"-> 0.000000000000  ,  \"Imoff\"-> 0.000000000000  |>   , \r\"IDS0370_210908_RAW_cal__sam_\" ->   <| \"ζ\"->  0.000000000000  , \"τ1\"-> 0.000000000000  , \"τS\"-> 0.000000000000  , \"τN\"-> 0.000000000000  , \"τC\"-> 0.000000000000  , \"κ0\"-> 0.000000000000  , \"mm1\"-> 0.000000000000  , \"mm2\"-> 0.000000000000  , \"mm3\"-> 0.000000000000  , \"T\"->  1.130000000000  , \"B\"-> 12.000000000000  , \"θ\"-> 60.000000000000  , \"Reoff\"-> 0.000000000000  ,  \"Imoff\"-> 0.000000000000  |>   , \r\"IDS0371_210908_RAW_cal__ref_\" ->   <| \"ζ\"->  0.020664849580  , \"τ1\"-> 0.018108723176  , \"τS\"-> 0.010299896170  , \"τN\"-> 0.000079818017  , \"τC\"-> 0.006259144045  , \"κ0\"-> 0.000000013130  , \"mm1\"-> 0.000000000000  , \"mm2\"-> 0.000000000000  , \"mm3\"-> 0.000000000000  , \"T\"->  1.900000000000  , \"B\"-> 12.000000000000  , \"θ\"-> 60.000000000000  , \"Reoff\"-> 0.000000000000  ,  \"Imoff\"-> 0.000000000000  |>   , \r\"IDS0371_210908_RAW_cal__sam_\" ->   <| \"ζ\"->  0.000000000000  , \"τ1\"-> 0.000000000000  , \"τS\"-> 0.000000000000  , \"τN\"-> 0.000000000000  , \"τC\"-> 0.000000000000  , \"κ0\"-> 0.000000000000  , \"mm1\"-> 0.000000000000  , \"mm2\"-> 0.000000000000  , \"mm3\"-> 0.000000000000  , \"T\"->  1.900000000000  , \"B\"-> 12.000000000000  , \"θ\"-> 60.000000000000  , \"Reoff\"-> 0.000000000000  ,  \"Imoff\"-> 0.000000000000  |>   , \r\"IDS0372_210908_RAW_cal__ref_\" ->   <| \"ζ\"->  0.021592146431  , \"τ1\"-> 0.018093446545  , \"τS\"-> 0.007071841556  , \"τN\"-> 0.000029085223  , \"τC\"-> 0.005341206531  , \"κ0\"-> 0.000000023517  , \"mm1\"-> 0.000000000000  , \"mm2\"-> 0.000000000000  , \"mm3\"-> 0.000000000000  , \"T\"->  3.110000000000  , \"B\"-> 12.000000000000  , \"θ\"-> 60.000000000000  , \"Reoff\"-> 0.000000000000  ,  \"Imoff\"-> 0.000000000000  |>   , \r\"IDS0372_210908_RAW_cal__sam_\" ->   <| \"ζ\"->  0.000000000000  , \"τ1\"-> 0.000000000000  , \"τS\"-> 0.000000000000  , \"τN\"-> 0.000000000000  , \"τC\"-> 0.000000000000  , \"κ0\"-> 0.000000000000  , \"mm1\"-> 0.000000000000  , \"mm2\"-> 0.000000000000  , \"mm3\"-> 0.000000000000  , \"T\"->  3.110000000000  , \"B\"-> 12.000000000000  , \"θ\"-> 60.000000000000  , \"Reoff\"-> 0.000000000000  ,  \"Imoff\"-> 0.000000000000  |>   , \r\"IDS0373_210908_RAW_cal__ref_\" ->   <| \"ζ\"->  0.028148688120  , \"τ1\"-> 0.012706961955  , \"τS\"-> 0.003881518121  , \"τN\"-> 0.000007160132  , \"τC\"-> 0.004346615253  , \"κ0\"-> 0.000000058313  , \"mm1\"-> 0.000000000000  , \"mm2\"-> 0.000000000000  , \"mm3\"-> 0.000000000000  , \"T\"->  5.750000000000  , \"B\"-> 12.000000000000  , \"θ\"-> 60.000000000000  , \"Reoff\"-> 0.000000000000  ,  \"Imoff\"-> 0.000000000000  |>   , \r\"IDS0373_210908_RAW_cal__sam_\" ->   <| \"ζ\"->  0.000000000000  , \"τ1\"-> 0.000000000000  , \"τS\"-> 0.000000000000  , \"τN\"-> 0.000000000000  , \"τC\"-> 0.000000000000  , \"κ0\"-> 0.000000000000  , \"mm1\"-> 0.000000000000  , \"mm2\"-> 0.000000000000  , \"mm3\"-> 0.000000000000  , \"T\"->  5.750000000000  , \"B\"-> 12.000000000000  , \"θ\"-> 60.000000000000  , \"Reoff\"-> 0.000000000000  ,  \"Imoff\"-> 0.000000000000  |>   , \r\"IDS0377_210909_RAW_cal__ref_\" ->   <| \"ζ\"->  0.217996441376  , \"τ1\"-> 0.079837328848  , \"τS\"-> 0.035140385542  , \"τN\"-> 0.027062270101  , \"τC\"-> 0.001091238478  , \"κ0\"-> 0.000000001044  , \"mm1\"-> 0.000000000000  , \"mm2\"-> 0.000000000000  , \"mm3\"-> 0.000000000000  , \"T\"->  0.197000000000  , \"B\"-> 8.000000000000  , \"θ\"-> 0.000000000000  , \"Reoff\"-> 0.000000000000  ,  \"Imoff\"-> 0.000000000000  |>   , \r\"IDS0377_210909_RAW_cal__sam_\" ->   <| \"ζ\"->  0.132375437908  , \"τ1\"-> 0.085614291193  , \"τS\"-> 0.046888304266  , \"τN\"-> 0.035744833495  , \"τC\"-> 0.001504622490  , \"κ0\"-> 0.000000001156  , \"mm1\"-> 0.000000000000  , \"mm2\"-> 0.000000000000  , \"mm3\"-> 0.000000000000  , \"T\"->  0.197000000000  , \"B\"-> 8.000000000000  , \"θ\"-> 0.000000000000  , \"Reoff\"-> 0.000000000000  ,  \"Imoff\"-> 0.000000000000  |>   , \r\"IDS0378_210909_RAW_cal__ref_\" ->   <| \"ζ\"->  0.444097524539  , \"τ1\"-> 0.128858676931  , \"τS\"-> 0.109017650637  , \"τN\"-> 0.152310736136  , \"τC\"-> 0.001225116605  , \"κ0\"-> 0.000000000395  , \"mm1\"-> 0.000000000000  , \"mm2\"-> 0.000000000000  , \"mm3\"-> 0.000000000000  , \"T\"->  0.122000000000  , \"B\"-> 8.000000000000  , \"θ\"-> 0.000000000000  , \"Reoff\"-> 0.000000000000  ,  \"Imoff\"-> 0.000000000000  |>   , \r\"IDS0378_210909_RAW_cal__sam_\" ->   <| \"ζ\"->  0.278068103221  , \"τ1\"-> 0.118058810167  , \"τS\"-> 0.149294349958  , \"τN\"-> 0.128211590058  , \"τC\"-> 0.001553934408  , \"κ0\"-> 0.000000000522  , \"mm1\"-> 0.000000000000  , \"mm2\"-> 0.000000000000  , \"mm3\"-> 0.000000000000  , \"T\"->  0.122000000000  , \"B\"-> 8.000000000000  , \"θ\"-> 0.000000000000  , \"Reoff\"-> 0.000000000000  ,  \"Imoff\"-> 0.000000000000  |>   , \r\"IDS0379_210909_RAW_cal__ref_\" ->   <| \"ζ\"->  0.358674724692  , \"τ1\"-> 0.106557394659  , \"τS\"-> 0.062757387956  , \"τN\"-> 0.083491977845  , \"τC\"-> 0.001111110425  , \"κ0\"-> 0.000000000629  , \"mm1\"-> 0.000000000000  , \"mm2\"-> 0.000000000000  , \"mm3\"-> 0.000000000000  , \"T\"->  0.148000000000  , \"B\"-> 8.000000000000  , \"θ\"-> 0.000000000000  , \"Reoff\"-> 0.000000000000  ,  \"Imoff\"-> 0.000000000000  |>   , \r\"IDS0379_210909_RAW_cal__sam_\" ->   <| \"ζ\"->  0.225754480330  , \"τ1\"-> 0.098523892400  , \"τS\"-> 0.080528394696  , \"τN\"-> 0.096491011881  , \"τC\"-> 0.001394999535  , \"κ0\"-> 0.000000000751  , \"mm1\"-> 0.000000000000  , \"mm2\"-> 0.000000000000  , \"mm3\"-> 0.000000000000  , \"T\"->  0.148000000000  , \"B\"-> 8.000000000000  , \"θ\"-> 0.000000000000  , \"Reoff\"-> 0.000000000000  ,  \"Imoff\"-> 0.000000000000  |>   , \r\"IDS0380_210909_RAW_cal__ref_\" ->   <| \"ζ\"->  0.289033994940  , \"τ1\"-> 0.085284172773  , \"τS\"-> 0.050519531224  , \"τN\"-> 0.055850802998  , \"τC\"-> 0.001015487958  , \"κ0\"-> 0.000000000740  , \"mm1\"-> 0.000000000000  , \"mm2\"-> 0.000000000000  , \"mm3\"-> 0.000000000000  , \"T\"->  0.168000000000  , \"B\"-> 8.000000000000  , \"θ\"-> 0.000000000000  , \"Reoff\"-> 0.000000000000  ,  \"Imoff\"-> 0.000000000000  |>   , \r\"IDS0380_210909_RAW_cal__sam_\" ->   <| \"ζ\"->  0.175421092430  , \"τ1\"-> 0.089198304544  , \"τS\"-> 0.059713999657  , \"τN\"-> 0.066015553792  , \"τC\"-> 0.001291009219  , \"κ0\"-> 0.000000000858  , \"mm1\"-> 0.000000000000  , \"mm2\"-> 0.000000000000  , \"mm3\"-> 0.000000000000  , \"T\"->  0.168000000000  , \"B\"-> 8.000000000000  , \"θ\"-> 0.000000000000  , \"Reoff\"-> 0.000000000000  ,  \"Imoff\"-> 0.000000000000  |>   , \r\"IDS0381_210909_RAW_cal__ref_\" ->   <| \"ζ\"->  0.126932147164  , \"τ1\"-> 0.058068643235  , \"τS\"-> 0.026925290066  , \"τN\"-> 0.010981117446  , \"τC\"-> 0.001219952265  , \"κ0\"-> 0.000000001350  , \"mm1\"-> 0.000000000000  , \"mm2\"-> 0.000000000000  , \"mm3\"-> 0.000000000000  , \"T\"->  0.250000000000  , \"B\"-> 8.000000000000  , \"θ\"-> 0.000000000000  , \"Reoff\"-> 0.000000000000  ,  \"Imoff\"-> 0.000000000000  |>   , \r\"IDS0381_210909_RAW_cal__sam_\" ->   <| \"ζ\"->  0.078113399712  , \"τ1\"-> 0.055920008457  , \"τS\"-> 0.035460304856  , \"τN\"-> 0.012612271055  , \"τC\"-> 0.001663430483  , \"κ0\"-> 0.000000001497  , \"mm1\"-> 0.000000000000  , \"mm2\"-> 0.000000000000  , \"mm3\"-> 0.000000000000  , \"T\"->  0.250000000000  , \"B\"-> 8.000000000000  , \"θ\"-> 0.000000000000  , \"Reoff\"-> 0.000000000000  ,  \"Imoff\"-> 0.000000000000  |>   , \r\"IDS0382_210909_RAW_cal__ref_\" ->   <| \"ζ\"->  0.087249653273  , \"τ1\"-> 0.047168507247  , \"τS\"-> 0.024336865487  , \"τN\"-> 0.005605961335  , \"τC\"-> 0.001526895316  , \"κ0\"-> 0.000000001730  , \"mm1\"-> 0.000000000000  , \"mm2\"-> 0.000000000000  , \"mm3\"-> 0.000000000000  , \"T\"->  0.300000000000  , \"B\"-> 8.000000000000  , \"θ\"-> 0.000000000000  , \"Reoff\"-> 0.000000000000  ,  \"Imoff\"-> 0.000000000000  |>   , \r\"IDS0382_210909_RAW_cal__sam_\" ->   <| \"ζ\"->  0.054029770351  , \"τ1\"-> 0.051440847518  , \"τS\"-> 0.032079834642  , \"τN\"-> 0.007150632998  , \"τC\"-> 0.002202148776  , \"κ0\"-> 0.000000001884  , \"mm1\"-> 0.000000000000  , \"mm2\"-> 0.000000000000  , \"mm3\"-> 0.000000000000  , \"T\"->  0.300000000000  , \"B\"-> 8.000000000000  , \"θ\"-> 0.000000000000  , \"Reoff\"-> 0.000000000000  ,  \"Imoff\"-> 0.000000000000  |>   , \r\"IDS0383_210910_RAW_cal__ref_\" ->   <| \"ζ\"->  0.062586766538  , \"τ1\"-> 0.048322657274  , \"τS\"-> 0.023582446152  , \"τN\"-> 0.003596780616  , \"τC\"-> 0.001965770478  , \"κ0\"-> 0.000000002106  , \"mm1\"-> 0.000000000000  , \"mm2\"-> 0.000000000000  , \"mm3\"-> 0.000000000000  , \"T\"->  0.360000000000  , \"B\"-> 8.000000000000  , \"θ\"-> 0.000000000000  , \"Reoff\"-> 0.000000000000  ,  \"Imoff\"-> 0.000000000000  |>   , \r\"IDS0383_210910_RAW_cal__sam_\" ->   <| \"ζ\"->  0.038341835326  , \"τ1\"-> 0.050866858713  , \"τS\"-> 0.030652081909  , \"τN\"-> 0.004623805952  , \"τC\"-> 0.002823684758  , \"κ0\"-> 0.000000002289  , \"mm1\"-> 0.000000000000  , \"mm2\"-> 0.000000000000  , \"mm3\"-> 0.000000000000  , \"T\"->  0.360000000000  , \"B\"-> 8.000000000000  , \"θ\"-> 0.000000000000  , \"Reoff\"-> 0.000000000000  ,  \"Imoff\"-> 0.000000000000  |>   , \r\"IDS0384_210910_RAW_cal__ref_\" ->   <| \"ζ\"->  0.047320664202  , \"τ1\"-> 0.050730770684  , \"τS\"-> 0.023716512211  , \"τN\"-> 0.002200072160  , \"τC\"-> 0.002249629457  , \"κ0\"-> 0.000000002636  , \"mm1\"-> 0.000000000000  , \"mm2\"-> 0.000000000000  , \"mm3\"-> 0.000000000000  , \"T\"->  0.430000000000  , \"B\"-> 8.000000000000  , \"θ\"-> 0.000000000000  , \"Reoff\"-> 0.000000000000  ,  \"Imoff\"-> 0.000000000000  |>   , \r\"IDS0384_210910_RAW_cal__sam_\" ->   <| \"ζ\"->  0.029950572027  , \"τ1\"-> 0.044923259835  , \"τS\"-> 0.030416367718  , \"τN\"-> 0.002541256331  , \"τC\"-> 0.003331031560  , \"κ0\"-> 0.000000002858  , \"mm1\"-> 0.000000000000  , \"mm2\"-> 0.000000000000  , \"mm3\"-> 0.000000000000  , \"T\"->  0.430000000000  , \"B\"-> 8.000000000000  , \"θ\"-> 0.000000000000  , \"Reoff\"-> 0.000000000000  ,  \"Imoff\"-> 0.000000000000  |>   , \r\"IDS0385_210910_RAW_cal__ref_\" ->   <| \"ζ\"->  0.037147896010  , \"τ1\"-> 0.047226564206  , \"τS\"-> 0.024619467421  , \"τN\"-> 0.001310789285  , \"τC\"-> 0.002565709752  , \"κ0\"-> 0.000000003275  , \"mm1\"-> 0.000000000000  , \"mm2\"-> 0.000000000000  , \"mm3\"-> 0.000000000000  , \"T\"->  0.530000000000  , \"B\"-> 8.000000000000  , \"θ\"-> 0.000000000000  , \"Reoff\"-> 0.000000000000  ,  \"Imoff\"-> 0.000000000000  |>   , \r\"IDS0385_210910_RAW_cal__sam_\" ->   <| \"ζ\"->  0.024600756648  , \"τ1\"-> 0.043958236582  , \"τS\"-> 0.031312750224  , \"τN\"-> 0.001348105931  , \"τC\"-> 0.003635120795  , \"κ0\"-> 0.000000003548  , \"mm1\"-> 0.000000000000  , \"mm2\"-> 0.000000000000  , \"mm3\"-> 0.000000000000  , \"T\"->  0.530000000000  , \"B\"-> 8.000000000000  , \"θ\"-> 0.000000000000  , \"Reoff\"-> 0.000000000000  ,  \"Imoff\"-> 0.000000000000  |>   , \r\"IDS0386_210910_RAW_cal__ref_\" ->   <| \"ζ\"->  0.028995432115  , \"τ1\"-> 0.046559455187  , \"τS\"-> 0.026126949833  , \"τN\"-> 0.000676599034  , \"τC\"-> 0.003300199116  , \"κ0\"-> 0.000000003897  , \"mm1\"-> 0.000000000000  , \"mm2\"-> 0.000000000000  , \"mm3\"-> 0.000000000000  , \"T\"->  0.630000000000  , \"B\"-> 8.000000000000  , \"θ\"-> 0.000000000000  , \"Reoff\"-> 0.000000000000  ,  \"Imoff\"-> 0.000000000000  |>   , \r\"IDS0386_210910_RAW_cal__sam_\" ->   <| \"ζ\"->  0.019494767421  , \"τ1\"-> 0.040349410363  , \"τS\"-> 0.033202805363  , \"τN\"-> 0.000770756985  , \"τC\"-> 0.004303152006  , \"κ0\"-> 0.000000004241  , \"mm1\"-> 0.000000000000  , \"mm2\"-> 0.000000000000  , \"mm3\"-> 0.000000000000  , \"T\"->  0.630000000000  , \"B\"-> 8.000000000000  , \"θ\"-> 0.000000000000  , \"Reoff\"-> 0.000000000000  ,  \"Imoff\"-> 0.000000000000  |>   , \r\"IDS0387_210910_RAW_cal__ref_\" ->   <| \"ζ\"->  0.021158107821  , \"τ1\"-> 0.047181877660  , \"τS\"-> 0.030519366684  , \"τN\"-> 0.000257878410  , \"τC\"-> 0.004211881541  , \"κ0\"-> 0.000000005418  , \"mm1\"-> 0.000000000000  , \"mm2\"-> 0.000000000000  , \"mm3\"-> 0.000000000000  , \"T\"->  0.830000000000  , \"B\"-> 8.000000000000  , \"θ\"-> 0.000000000000  , \"Reoff\"-> 0.000000000000  ,  \"Imoff\"-> 0.000000000000  |>   , \r\"IDS0387_210910_RAW_cal__sam_\" ->   <| \"ζ\"->  0.013958531253  , \"τ1\"-> 0.040449551738  , \"τS\"-> 0.038075316972  , \"τN\"-> 0.000218997482  , \"τC\"-> 0.005348147372  , \"κ0\"-> 0.000000005866  , \"mm1\"-> 0.000000000000  , \"mm2\"-> 0.000000000000  , \"mm3\"-> 0.000000000000  , \"T\"->  0.830000000000  , \"B\"-> 8.000000000000  , \"θ\"-> 0.000000000000  , \"Reoff\"-> 0.000000000000  ,  \"Imoff\"-> 0.000000000000  |>   , \r\"IDS0388_210910_RAW_cal__ref_\" ->   <| \"ζ\"->  0.017074092265  , \"τ1\"-> 0.047215899415  , \"τS\"-> 0.039490388664  , \"τN\"-> 0.000122819272  , \"τC\"-> 0.004722965607  , \"κ0\"-> 0.000000007547  , \"mm1\"-> 0.000000000000  , \"mm2\"-> 0.000000000000  , \"mm3\"-> 0.000000000000  , \"T\"->  1.130000000000  , \"B\"-> 8.000000000000  , \"θ\"-> 0.000000000000  , \"Reoff\"-> 0.000000000000  ,  \"Imoff\"-> 0.000000000000  |>   , \r\"IDS0388_210910_RAW_cal__sam_\" ->   <| \"ζ\"->  0.011551866824  , \"τ1\"-> 0.040411227639  , \"τS\"-> 0.048181354691  , \"τN\"-> 0.000103559724  , \"τC\"-> 0.006232382617  , \"κ0\"-> 0.000000008161  , \"mm1\"-> 0.000000000000  , \"mm2\"-> 0.000000000000  , \"mm3\"-> 0.000000000000  , \"T\"->  1.130000000000  , \"B\"-> 8.000000000000  , \"θ\"-> 0.000000000000  , \"Reoff\"-> 0.000000000000  ,  \"Imoff\"-> 0.000000000000  |>   , \r\"IDS0389_210910_RAW_cal__ref_\" ->   <| \"ζ\"->  0.017157539727  , \"τ1\"-> 0.046379456311  , \"τS\"-> 0.015264158508  , \"τN\"-> 0.000057006071  , \"τC\"-> 0.004702188691  , \"κ0\"-> 0.000000010470  , \"mm1\"-> 0.000000000000  , \"mm2\"-> 0.000000000000  , \"mm3\"-> 0.000000000000  , \"T\"->  1.520000000000  , \"B\"-> 8.000000000000  , \"θ\"-> 0.000000000000  , \"Reoff\"-> 0.000000000000  ,  \"Imoff\"-> 0.000000000000  |>   , \r\"IDS0389_210910_RAW_cal__sam_\" ->   <| \"ζ\"->  0.011148198813  , \"τ1\"-> 0.038849151842  , \"τS\"-> 0.019213865355  , \"τN\"-> 0.000045035153  , \"τC\"-> 0.005536708133  , \"κ0\"-> 0.000000011229  , \"mm1\"-> 0.000000000000  , \"mm2\"-> 0.000000000000  , \"mm3\"-> 0.000000000000  , \"T\"->  1.520000000000  , \"B\"-> 8.000000000000  , \"θ\"-> 0.000000000000  , \"Reoff\"-> 0.000000000000  ,  \"Imoff\"-> 0.000000000000  |>   , \r\"IDS0390_210910_RAW_cal__ref_\" ->   <| \"ζ\"->  0.016425367394  , \"τ1\"-> 0.039829137916  , \"τS\"-> 0.010121167967  , \"τN\"-> 0.000033814494  , \"τC\"-> 0.004533563026  , \"κ0\"-> 0.000000013089  , \"mm1\"-> 0.000000000000  , \"mm2\"-> 0.000000000000  , \"mm3\"-> 0.000000000000  , \"T\"->  1.900000000000  , \"B\"-> 8.000000000000  , \"θ\"-> 0.000000000000  , \"Reoff\"-> 0.000000000000  ,  \"Imoff\"-> 0.000000000000  |>   , \r\"IDS0390_210910_RAW_cal__sam_\" ->   <| \"ζ\"->  0.010826949430  , \"τ1\"-> 0.038768037521  , \"τS\"-> 0.012925317198  , \"τN\"-> 0.000029157336  , \"τC\"-> 0.005196063884  , \"κ0\"-> 0.000000013864  , \"mm1\"-> 0.000000000000  , \"mm2\"-> 0.000000000000  , \"mm3\"-> 0.000000000000  , \"T\"->  1.900000000000  , \"B\"-> 8.000000000000  , \"θ\"-> 0.000000000000  , \"Reoff\"-> 0.000000000000  ,  \"Imoff\"-> 0.000000000000  |>   , \r\"IDS0391_210910_RAW_cal__ref_\" ->   <| \"ζ\"->  0.016160769926  , \"τ1\"-> 0.047360928893  , \"τS\"-> 0.041725389227  , \"τN\"-> 0.000076715950  , \"τC\"-> 0.004871049589  , \"κ0\"-> 0.000000008346  , \"mm1\"-> 0.000000000000  , \"mm2\"-> 0.000000000000  , \"mm3\"-> 0.000000000000  , \"T\"->  1.250000000000  , \"B\"-> 8.000000000000  , \"θ\"-> 0.000000000000  , \"Reoff\"-> 0.000000000000  ,  \"Imoff\"-> 0.000000000000  |>   , \r\"IDS0391_210910_RAW_cal__sam_\" ->   <| \"ζ\"->  0.010962610928  , \"τ1\"-> 0.040398807374  , \"τS\"-> 0.051328988590  , \"τN\"-> 0.000070281011  , \"τC\"-> 0.006422533164  , \"κ0\"-> 0.000000008958  , \"mm1\"-> 0.000000000000  , \"mm2\"-> 0.000000000000  , \"mm3\"-> 0.000000000000  , \"T\"->  1.250000000000  , \"B\"-> 8.000000000000  , \"θ\"-> 0.000000000000  , \"Reoff\"-> 0.000000000000  ,  \"Imoff\"-> 0.000000000000  |>   , \r\"IDS0392_210910_RAW_cal__ref_\" ->   <| \"ζ\"->  0.016250541117  , \"τ1\"-> 0.047393343666  , \"τS\"-> 0.029998719281  , \"τN\"-> 0.000076850447  , \"τC\"-> 0.004810494325  , \"κ0\"-> 0.000000009475  , \"mm1\"-> 0.000000000000  , \"mm2\"-> 0.000000000000  , \"mm3\"-> 0.000000000000  , \"T\"->  1.390000000000  , \"B\"-> 8.000000000000  , \"θ\"-> 0.000000000000  , \"Reoff\"-> 0.000000000000  ,  \"Imoff\"-> 0.000000000000  |>   , \r\"IDS0392_210910_RAW_cal__sam_\" ->   <| \"ζ\"->  0.010962610928  , \"τ1\"-> 0.040398807374  , \"τS\"-> 0.051328988590  , \"τN\"-> 0.000070281011  , \"τC\"-> 0.006422533164  , \"κ0\"-> 0.000000008958  , \"mm1\"-> 0.000000000000  , \"mm2\"-> 0.000000000000  , \"mm3\"-> 0.000000000000  , \"T\"->  1.390000000000  , \"B\"-> 8.000000000000  , \"θ\"-> 0.000000000000  , \"Reoff\"-> 0.000000000000  ,  \"Imoff\"-> 0.000000000000  |>   , \r\"IDS0393_210910_RAW_cal__ref_\" ->   <| \"ζ\"->  0.015227705493  , \"τ1\"-> 0.038797003927  , \"τS\"-> 0.007286355621  , \"τN\"-> 0.000013994204  , \"τC\"-> 0.003959851165  , \"κ0\"-> 0.000000023455  , \"mm1\"-> 0.000000000000  , \"mm2\"-> 0.000000000000  , \"mm3\"-> 0.000000000000  , \"T\"->  3.110000000000  , \"B\"-> 8.000000000000  , \"θ\"-> 0.000000000000  , \"Reoff\"-> 0.000000000000  ,  \"Imoff\"-> 0.000000000000  |>   , \r\"IDS0393_210910_RAW_cal__sam_\" ->   <| \"ζ\"->  0.010962610928  , \"τ1\"-> 0.040398807374  , \"τS\"-> 0.051328988590  , \"τN\"-> 0.000070281011  , \"τC\"-> 0.006422533164  , \"κ0\"-> 0.000000008958  , \"mm1\"-> 0.000000000000  , \"mm2\"-> 0.000000000000  , \"mm3\"-> 0.000000000000  , \"T\"->  3.110000000000  , \"B\"-> 8.000000000000  , \"θ\"-> 0.000000000000  , \"Reoff\"-> 0.000000000000  ,  \"Imoff\"-> 0.000000000000  |>   , \r\"IDS0394_210910_RAW_cal__ref_\" ->   <| \"ζ\"->  0.018884017265  , \"τ1\"-> 0.038756536887  , \"τS\"-> 0.005123025136  , \"τN\"-> 0.000004793994  , \"τC\"-> 0.002621800478  , \"κ0\"-> 0.000000058143  , \"mm1\"-> 0.000000000000  , \"mm2\"-> 0.000000000000  , \"mm3\"-> 0.000000000000  , \"T\"->  5.750000000000  , \"B\"-> 8.000000000000  , \"θ\"-> 0.000000000000  , \"Reoff\"-> 0.000000000000  ,  \"Imoff\"-> 0.000000000000  |>   , \r\"IDS0394_210910_RAW_cal__sam_\" ->   <| \"ζ\"->  0.010962610928  , \"τ1\"-> 0.040398807374  , \"τS\"-> 0.051328988590  , \"τN\"-> 0.000070281011  , \"τC\"-> 0.006422533164  , \"κ0\"-> 0.000000008958  , \"mm1\"-> 0.000000000000  , \"mm2\"-> 0.000000000000  , \"mm3\"-> 0.000000000000  , \"T\"->  5.750000000000  , \"B\"-> 8.000000000000  , \"θ\"-> 0.000000000000  , \"Reoff\"-> 0.000000000000  ,  \"Imoff\"-> 0.000000000000  |>   , \r\"IDS0395_210910_RAW_cal__ref_\" ->   <| \"ζ\"->  0.016101273075  , \"τ1\"-> 0.047373144247  , \"τS\"-> 0.040453117489  , \"τN\"-> 0.000076678480  , \"τC\"-> 0.005036745304  , \"κ0\"-> 0.000000008627  , \"mm1\"-> 0.000000000000  , \"mm2\"-> 0.000000000000  , \"mm3\"-> 0.000000000000  , \"T\"->  1.310000000000  , \"B\"-> 8.000000000000  , \"θ\"-> 0.000000000000  , \"Reoff\"-> 0.000000000000  ,  \"Imoff\"-> 0.000000000000  |>   , \r\"IDS0395_210910_RAW_cal__sam_\" ->   <| \"ζ\"->  0.010962610928  , \"τ1\"-> 0.040398807374  , \"τS\"-> 0.051328988590  , \"τN\"-> 0.000070281011  , \"τC\"-> 0.006422533164  , \"κ0\"-> 0.000000008958  , \"mm1\"-> 0.000000000000  , \"mm2\"-> 0.000000000000  , \"mm3\"-> 0.000000000000  , \"T\"->  1.310000000000  , \"B\"-> 8.000000000000  , \"θ\"-> 0.000000000000  , \"Reoff\"-> 0.000000000000  ,  \"Imoff\"-> 0.000000000000  |>   , \r")   [LabVIEW 2020]
uses:
  3-lorentzian-heat-response action.ctl
  3-lorentzian-parameters.ctl
  mathematica string map action.ctl
  3-lorentzian-heat-response -- V4.vi/142dd4c5-f9ed-c64b-bc14-a88e3e2c450a.vi
  <vilib>/Analysis/polynomials.llb/Multiply Polynomials.vi
  <vilib>/Analysis/polynomials.llb/Multiply Polynomials (DBL).vi
  <vilib>/Analysis/polynomials.llb/Polynomial Roots.vi
  <vilib>/Analysis/polynomials.llb/Polynomial Roots (DBL).vi
  <vilib>/Comparison/Less/Less Functor/Less Functor.lvclass
  <vilib>/regexp/Match Regular Expression.xnode
panel:
  out "after match":string
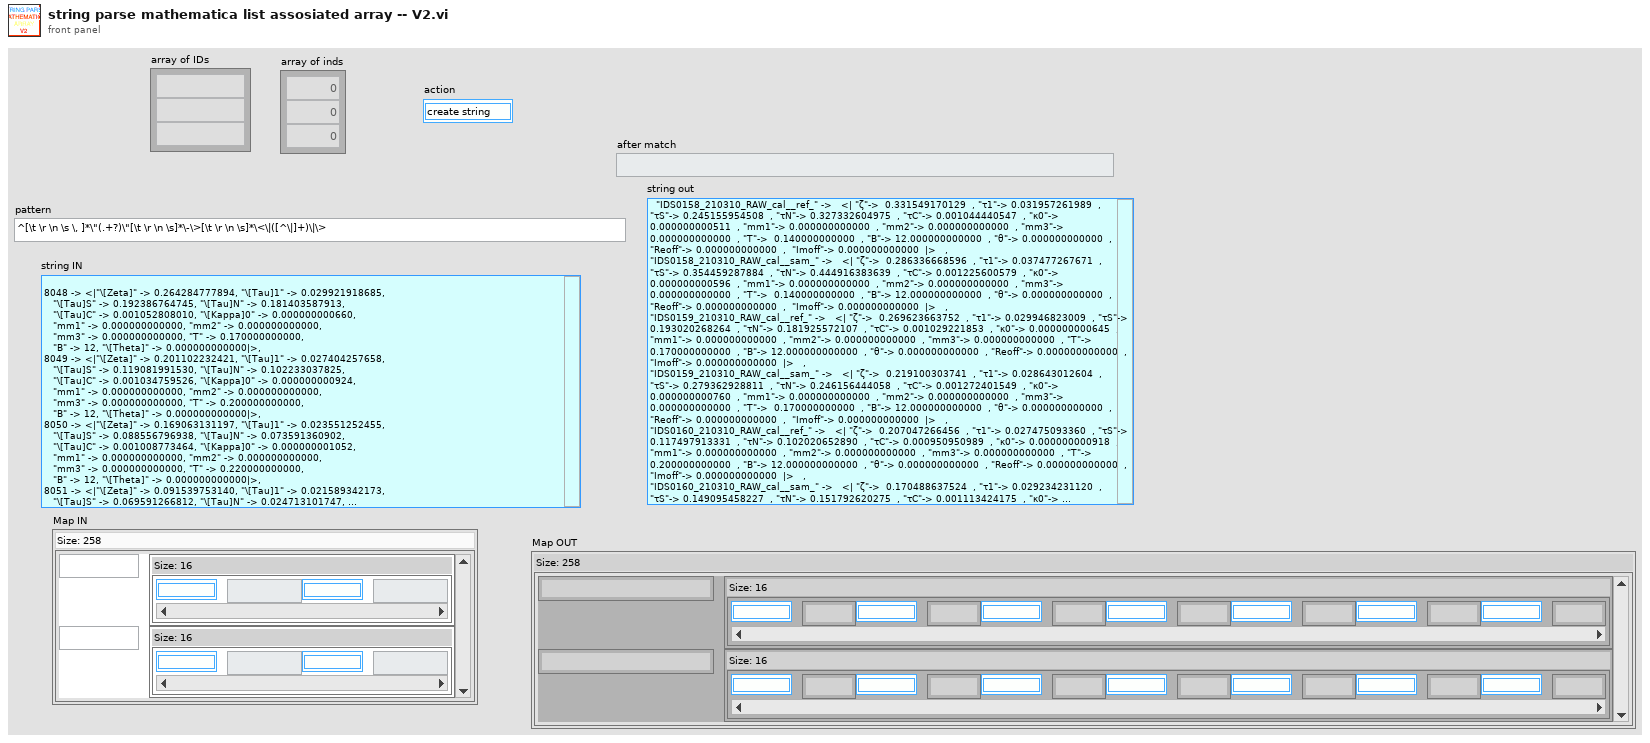
[diagram p1: front panel]
types:
  T1 = typedef "3-lorentzian-parameters.ctl" = enum16{"ζ", "τ1", "τS", "τN", "τC", "κ0", "m1", "m2", "m3", "T (K)", "B (T)", "θ (deg)", "side (S|R)", "set of (B|T)", "Re(offset)", "Im(offset)"}
  T2 = typedef "3-lorentzian-heat-response action.ctl" = enum16{"calc R", "create string", "calc m1m2m3", "dζ", "dT1", "dτS", "dτN", "dτC", "d-all", "dκ0", "T(K)", "m1", "m2", "m3", "parse string", "θ (deg)", "B (T)", "onlygrads", "newton", "create emty string"}
  T3 = typedef "mathematica string map action.ctl" = enum16{"create string", "calc m1m2m3", "parse string"}
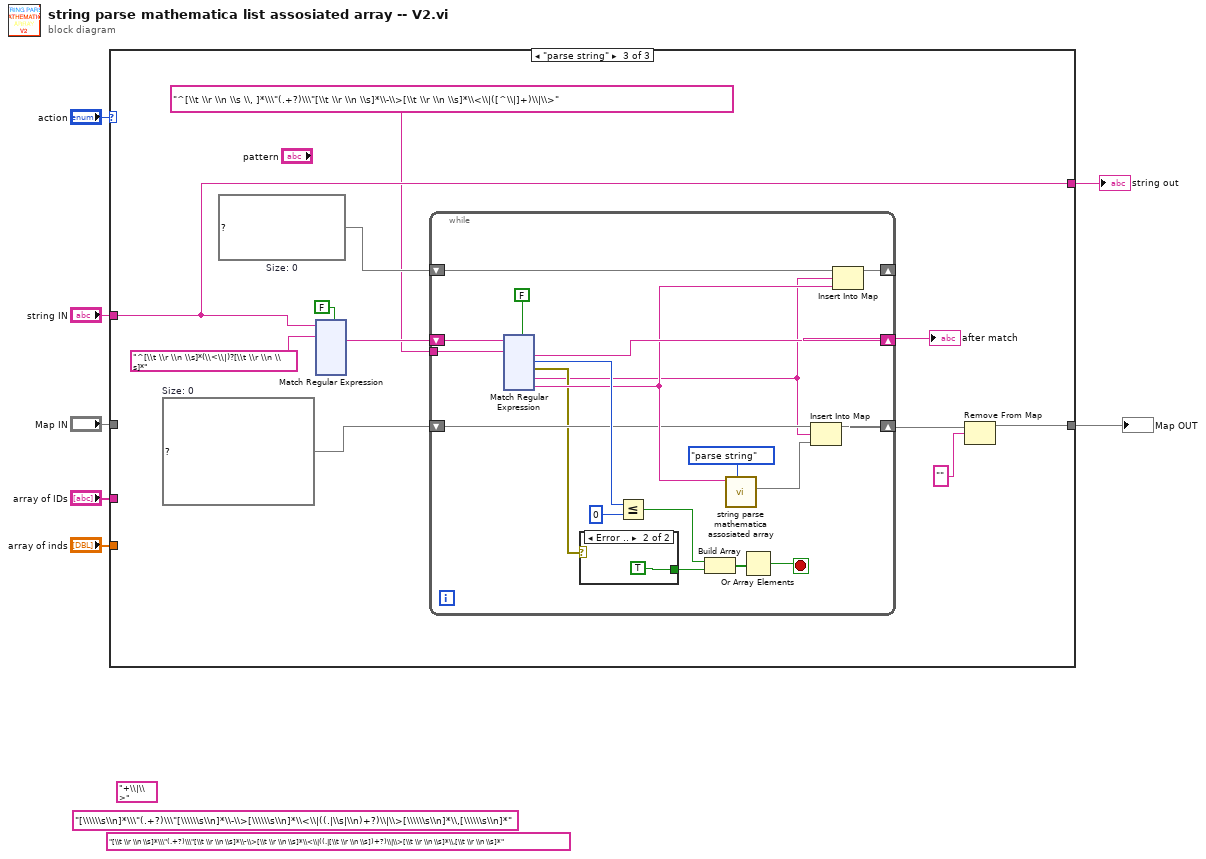
[diagram p0: block diagram]
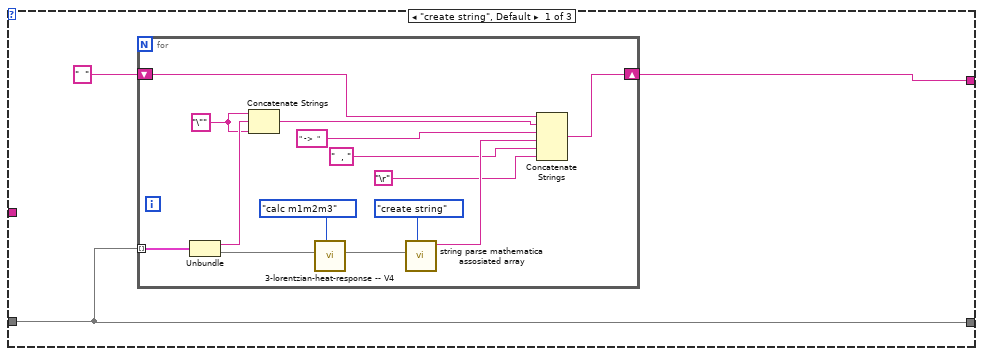
[diagram p2: hidden frame]
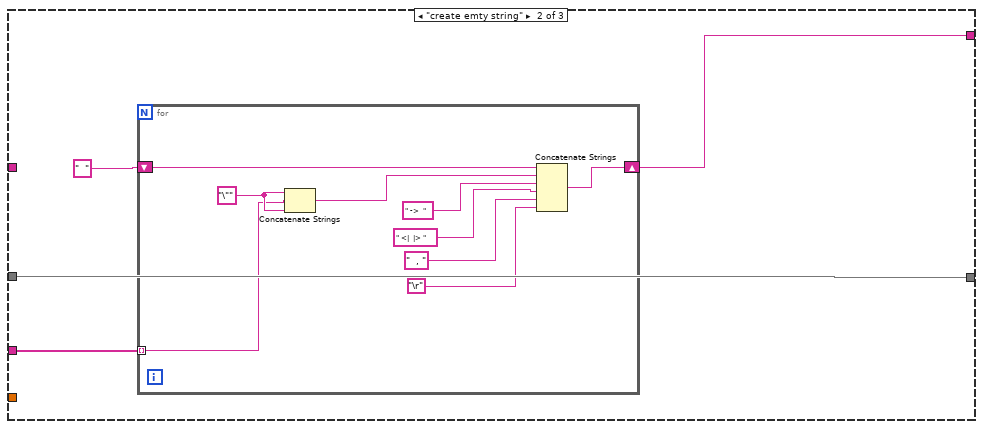
[diagram p3: hidden frame]
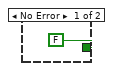
[diagram p4: hidden frame]
diagram:
  (unwired) "+\\|\\>" ("format string")
  (unwired) "[\\t \\r \\n \\s]*\\\"(.+?)\\\"[\\t \\r \\n \\s]*\\-\\>[\\t \\r \\n \\s]*\\<\\|((.|[\\t \\r \\n \\s])+?)\\|\\>[\\t \\r \\n \\s]*\\,[\\t \\r \\n \\s]*" ("pattern")
  (unwired) "[\\\\\\s\\n]*\\\"(.+?)\\\"[\\\\\\s\\n]*\\-\\>[\\\\\\s\\n]*\\<\\|((.|\\s|\\n)+?)\\|\\>[\\\\\\s\\n]*\\,[\\\\\\s\\n]*" ("pattern")
  n1 = case shown="\"parse string\"" "action" {
    tunnel: "string IN" -> [_ _ w41]
    tunnel: [w8 w26 w42] -> w2
    tunnel: "Map IN" -> [w8 w26 _]
    tunnel: [w10 w28 w41] -> w4
    tunnel: "array of inds" -> [_ _ _]
    tunnel: "array of IDs" -> [_ w25 _]
    frame "create string", Default {
      n2 = for {
        tunnel: w8 -> [w24] mode=indexing
        shift-right: [w18] -> w10
        shift-left: "  " ("all string") -> [w19]
        w11 = "\"" ("all string")
        n3 = Unbundle(w24) -> ("after match 3"=w13:string, "Map"=w16:map{T1, dbl})
        n4 = Concatenate Strings(w11, w13, w11) -> (w12:string)
        n5 = call "3-lorentzian-heat-response -- V4.vi"("action"=3-lorentzian-heat-response_action."calc m1m2m3", "Map IN"=w16) -> ("Map OUT"=w14:map{T1, dbl})  [unwired: 7 in, 2 out]
        n6 = call "string parse mathematica assosiated array.vi"("action"=mathematica_string_map_action."create string" ("derivative"), "map IN"=w14) -> ("String OUT"=w22:string)  [unwired: 8 in, 1 out]
        n7 = Concatenate Strings(w19, w12, " ->  " ("all string"), w22, "  , " ("all string"), "\r") -> (w18:string)
      }
    }
    frame "create emty string" {
      n8 = for {
        shift-right: [w34] -> w28
        shift-left: "  " ("all string") -> [w35]
        tunnel: w25 -> [w30] mode=indexing
        w31 = "\"" ("all string")
        n9 = Concatenate Strings(w31, w30, w31) -> (w29:string)
        n10 = Concatenate Strings(w35, w29, " ->  " ("all string"), " <|  |> " ("all string"), "  , " ("all string"), "\r") -> (w34:string)
      }
    }
    frame "parse string" {
      w44 = map{string, map{T1, dbl}} {}  # Size: 0
      w46 = map{string, string} {}  # Size: 0
      n11 = xnode "Match Regular Expression"("input string"=w41, "regular expression"="^[\\t \\r \\n \\s]*(\\<\\|)?[\\t \\r \\n \\s]*" ("format string"), "multiline? (F)"=FALSE) -> ("after match"=w47:string)  [unwired: 3 in, 6 out]
      n12 = while {
        shift-right: [w64] -> w45
        shift-left: w47 -> [w67]
        shift-right: [w62] -> _
        shift-left: w46 -> [w63]
        shift-right: [w57] -> w43
        shift-left: w44 -> [w59]
        tunnel: "^[\\t \\r \\n \\s \\, ]*\\\"(.+?)\\\"[\\t \\r \\n \\s]*\\-\\>[\\t \\r \\n \\s]*\\<\\|([^\\|]+)\\|\\>" ("pattern") -> [w49]
        stop <- w53 stop-if-true
        n13 = xnode "Match Regular Expression"("input string"=w67, "regular expression"=w49, "multiline? (F)"=FALSE) -> ("after match"=w64:string, "offset past match"=w66:i32, "error out"=w54:errorcluster, "submatch 1"=w50:string, "submatch 2"=w60:string)  [unwired: 3 in, 2 out]
        n14 = case shown="Error .." w54 {
          tunnel: [FALSE TRUE] -> w51
          frame No Error {
          }
          frame Error {
          }
        }
        n15 = Less Or Equal?(x=w66, y=0) -> (x <= y?=w55:bool)
        n16 = Build Array(w55, w51) -> (w52:bool[])
        n17 = call "string parse mathematica assosiated array.vi"("action"=mathematica_string_map_action."parse string" ("derivative"), "String in"=w60) -> ("Map OUT"=w58:map{T1, dbl})  [unwired: 8 in, 1 out]
        n18 = Or Array Elements(Boolean array=w52) -> (logical OR=w53:bool)
        n19 = Insert Into Map(map in=w59, key=w50, value=w58) -> (map out=w57:map{string, map{T1, dbl}})  [unwired: 2 out]
        n20 = Insert Into Map(map in=w63, key=w50, value=w60) -> (map out=w62:map{string, string})  [unwired: 2 out]
      }
      "after match" <- w45
      n21 = Remove From Map(10:"" ("format string"), 11:w43) -> (3:w42:map{string, map{T1, dbl}})  [unwired: 2 out]
    }
  }
  "string out" <- w4
  "Map OUT" <- w2
